vi "COD主界面（列队使用）.vi"() -> (8 "多列列表框":i32(listbox))   [LabVIEW 2016, in "斯坦道CODMn.lvlib"]
uses:
  <vilib>/Analysis/6fits.llb/Curve Fitting Criteria.ctl
  <vilib>/Utility/miscctls.llb/LVPointTypeDef.ctl
  <vilib>/Utility/config.llb/Read Key (I32).vi
  <vilib>/Utility/config.llb/Read Key (Double).vi
  <vilib>/Utility/config.llb/Read Key (Boolean).vi
  <vilib>/Utility/config.llb/Write Key (Double).vi
  <vilib>/Utility/config.llb/Write Key (Boolean).vi
  <vilib>/Utility/config.llb/Write Key (I32).vi
  <vilib>/Waveform/WDTFileIO.llb/Read Waveform from File.vi
  <vilib>/ptbypt/NI_PtbyPt.lvlib
  <vilib>/Utility/config.llb/NI_LVConfig.lvlib
  <vilib>/Analysis/NI_AALPro.lvlib
panel:
  in  "更新程序":bool
  out "进样无液体告警":bool
  out "校准内容显示":string
  out "60分钟超时报警":bool
  in  "远程校准量程":enum16{"L", "H"}(ring)
  in  "远程自动校准浓度":dbl
  in  "仪器参数":bool
  out "CODMn序列号":string
  out "CODMn软件版本：":string
  in  "标样核查量程选择":enum32{"H", "L", "AUTO"}(ring)=enum."AUTO"
  in  "标样浓度":dbl
  in  "零点核查量程选择":enum32{"H", "L", "AUTO"}(ring)=enum."AUTO"
  in  "零点核查浓度":dbl
  out "序列号":string
  in  "采水泵排液时间/s:":i32
  in  "采水泵润洗时间/s:":i32
  in  "采水泵沉淀时间/s:":i32
  in  "采水泵进样时间/s:":i32
  in  "常规版/认证版":enum16{"常规版", "认证版", "浮台版"}(ring)
  in  "释放串口":bool
  in  "打开串口":bool
  in  "保存参数":dbl[](array[numeric])
  out "报警数字":i16
  out "CODMn工作状态":T1(ring)
  out "ORP-K":string
  out "ORP-B":string
  out "ORP-A":string
  out "x = y?":bool
  out "稀释倍数解释":string
  in  "跨度量程选择":enum32{"H", "L", "AUTO"}(ring)=enum."AUTO"
  in  "跨度液浓度":dbl
  in  "水样：":dbl
  in  "蒸馏水：":dbl
  in  "标液：":dbl
  in  "零点核查样：":dbl
  in  "加标回收样：":dbl
  in  "草酸钠":dbl
  in  "高锰酸钾":dbl
  in  "硫酸":dbl
  out "量程解释说明":string
  in  "高切低阈值:":dbl
  in  "低切高阈值:":dbl
  in  "水样量程选择:":enum16{"L", "H", "自动切换测一次", "自动切换测两次"}(ring)
  in  "修正系数：":dbl
  in  "标准液浓度":dbl
  in  "温度":dbl
  in  "恒温时间":dbl
  in  "当前量程：":enum16{"L", "H"}(ring)
  in  "CODMn零点核查选择":enum16{"零点核查走纯水管", "零点核查走零漂管"}(ring)
  in  "锁定按钮":bool
  in  "低量程稀释倍数:":i8=1
  in  "高量程稀释倍数:":i8=2
  in  "一键写入":bool
  in  "测量模式(公式)":u16(ring)=1 items=["水样测试"=1, "标样核查"=2, "零点核查"=3, "跨度核查"=4, "空白测试"=5, "平行样"=6, "加标回收"=7]
  out "基本量程(显示)":string
  out "测量模式(显示)":string
  out "数据时间":string
  out "断电排液标记":bool
  out "COM":string
  in  "启用5":bool
  in  "校准5":bool
  in  "泵滴定数5":dbl
  in  "浓度5":dbl
  in  "启用4":bool
  in  "校准4":bool
  in  "泵滴定数4":dbl
  in  "浓度4":dbl
  out "波形时间":timestamp
  in  "历史波形":bool
  out "滴定数-ORP值":u16[](array[numeric]) caption="数组"
  in  "关闭 3":bool
  in  "滴定曲线":bool
  out "ORP滴定曲线":u16[](graph)
  out "空白测试标记":bool
  out "跨度核查标记":bool
  in  "量程选择":enum16{"低量程", "高量程", "0-2量程"}(ring)
  in  "手动控制":bool
  in  "选用水样":enum16{"葡萄糖", "草酸钠"}(ring)
  in  "方程系数":cluster{"K":dbl, "b":dbl, "X^2":dbl} {"X^2" format="%#.6g"; "b" format="%#.6g"; "K" format="%#.6g"}
  out "多项式系数":dbl[](array[numeric])
  out "XY图":cluster{"X Values":dbl[], "Y Values":dbl[]}[](graph)
  in  "模型":enum32{"线性", "多项式"}(ring)
  out "启动时间":timestamp format="%<%Y/%m/%d %H:%M:%S>T"
  in  "关闭 2":bool
  out "r^2":dbl format="%.8g"
  out "拟合公式":string
  out "b":dbl format="%#.4g"
  out "K":dbl format="%#.4f"
  in  "启用3":bool
  in  "启用2":bool
  in  "启用1":bool
  in  "校准3":bool
  in  "校准2":bool
  in  "校准1":bool
  in  "泵滴定数3":dbl
  in  "泵滴定数2":dbl
  in  "泵滴定数1":dbl
  in  "浓度3":dbl
  in  "浓度2":dbl
  in  "浓度1":dbl
  in  "写入":bool
  out "零点核查标记":bool
  out "排液故障":bool
  out "进水样超量程":bool
  out "标样核查标记":bool
  out "平行样测量":bool
  out "加标回收测量":bool
  out "质控样测量":bool
  out "待机":bool
  out "校标错误":bool
  out "校零错误":bool
  out "测量错误":bool
  out "草酸钠报警":bool
  out "高锰酸钾报警":bool
  out "加热故障":bool
  out "温控器故障":bool
  out "ORP故障":bool
  out "排液标记":bool
  out "故障标记":bool
  out "校标标记":bool
  out "校零标记":bool
  out "通讯状态":bool
  out "水样测量":bool
  in  "读取":bool
  in  "返回":bool
  in  "校准配置":bool
  in  "零点泵计量数 2":dbl
  in  "标度泵计量数 2":dbl
  out "标度滴定值":dbl
  out "零点滴定值":dbl
  in  "保存":bool
  in  "关闭":bool
  out "仪器时间":timestamp format="%<%Y/%m/%d %H:%M:%S>T"
  out "秒":u16
  out "分":u16
  out "COD浓度（mg/L)":dbl format="%.2g"
  out "进样管":dbl
  out "高锰酸钾":dbl
  out "草酸钠":dbl
  out "硫酸":dbl
  out "ORP显示":dbl
  out "温度":dbl
  out "加热":bool
  out "搅拌":bool
  out "进硫酸":bool
  out "进加标回收样":bool
  out "进零点核查样":bool
  out "进标液":bool
  out "进蒸馏水":bool
  out "进水样":bool
  out "进草酸钠":bool
  out "进高锰酸钾":bool
  out "定时启动":bool
  in  "启动":bool
  in  "故障清除":bool
  in  "参数配置":bool
  in  "停止":bool
  in  "单步启动":bool
  out "系统时间":timestamp
  in  "时间校准":bool
  out "模式（受控）":u16
  # "测量时间："
  # "mV"
  # "℃"
  # "注：遇到加热故障和排液故障时仪器不能正常启动，\n必须排查故障并点击报警清除按钮方可运行。"
  # "mg/L"
  # "基本参数设置"
  # "校零校标结果"
  # "泵计量参数设置"
  # "校零结果："
  # "校零滴定值："
  # "加热恒温温度(℃):"
  # "高锰酸钾："
  # "校标结果："
  # "标度滴定值："
  # "恒温时间(分钟):"
  # "草酸钠："
  # "零点泵计量值："
  # "标准液浓度(mg/L):"
  # "硫酸："
  # "标度泵计量值："
  # "跨度核查浓度："
  # "跨度量程选择："
  # "零点核查浓度："
  # "标样浓度："
  # "零点量程选择："
  # "标样量程选择："
  # "远程校准配置区"
  # "公式读取写入区"
  # "mg/L"
  # "是否启用"
  # "泵滴定数"
  # "浓度"
  # "辅\n助\n计\n算\n区"
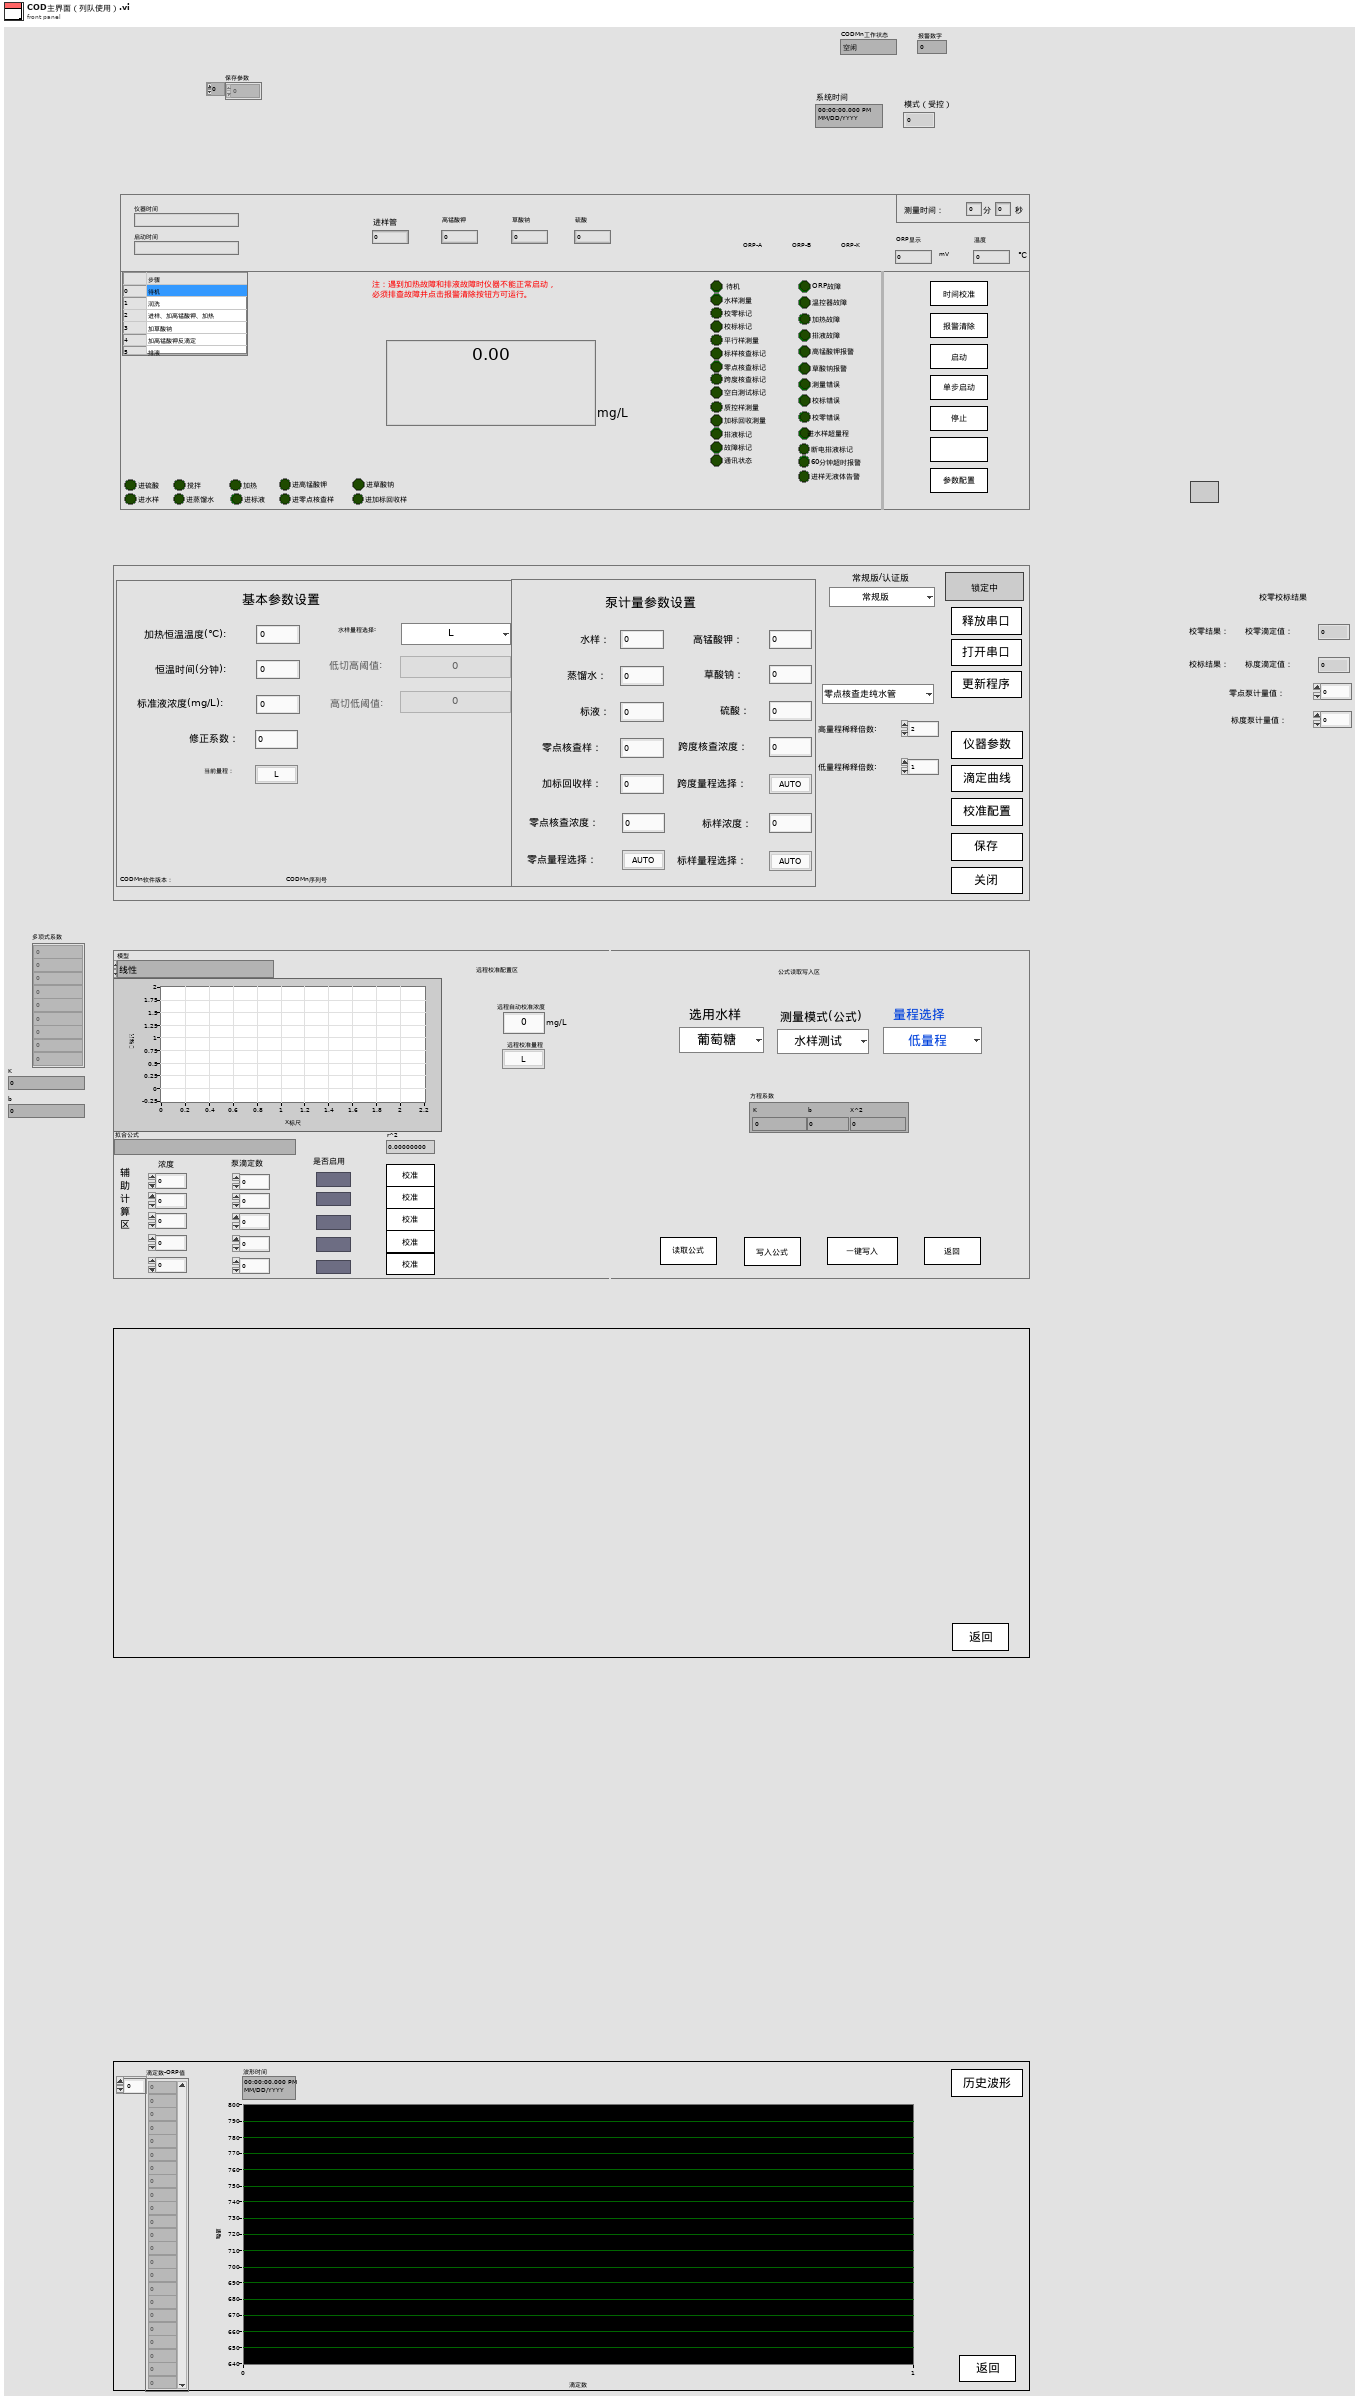
[diagram p1: front panel]
types:
  T1 = enum16{"空闲", "水样测试", "标样核查", "零点核查", "跨度核查", "空白测试", "平行样测试", "质控样", "空白校准", "标样校准", "加标回收"}
  T2 = typedef "NI_AALPro.lvlib/Curve Fitting Criteria.ctl" = u16
  T3 = cluster{"测量量程":dbl, "测量精度":dbl, "测量间隔":dbl, "消解温度":dbl, "消解时长":dbl, "空白校准时间":timestamp, "曲线截距":dbl, "曲线斜率":dbl, "测量检出限":dbl, "测量信号值":dbl, "线性相关系数":dbl, "二次多项式系数":dbl, "标样校准时间":timestamp, "单位":u16}
  T4 = enum8{"Enabled", "Disabled", "Disabled and Grayed Out"}
  T5 = typedef "LVPointTypeDef.ctl" = cluster{"Horizontal":i16, "Vertical":i16}
  T6 = typedef "NI_LVConfig.lvlib/Config Data RefNum.ctl" = refnum<k1>
  T7 = cluster{"时间":timestamp, "测量模式":string, "数据类型":string, "检测值":sgl, "单位":string, "数据标识":string, "因子编码":string, "标样参考值":sgl, "ORP-A":sgl, "ORP-B":sgl, "ORP-K":sgl, "COD滴定值":sgl, "高锰酸钾滴定数":sgl, "温度":sgl, "量程":sgl, "LastTime":timestamp}
  T8 = cluster{"因子编码":u32, "单位":u16, "标样参考值":sgl, "水样数据时间":timestamp, "水样实测值":sgl, "水样数据标识":string, "标样数据时间":timestamp, "标样实测值":sgl, "标样数据标识":string, "空白数据时间":timestamp, "空白实测值":sgl, "空白数据标识":string, "零点核查数据时间":timestamp, "零点核查实测值":sgl, "零点核查数据标识":string, "跨度核查数据时间":timestamp, "跨度核查实测值":sgl, "跨度核查数据标识":string, "加标回收数据时间":timestamp, "加标回收实测值":sgl, "加标回收数据标识":string, "平行样数据时间":timestamp, "平行样实测值":sgl, "平行样数据标识":string}
  T9 = cluster{"控制命令":enum16{"启动测量", "标样核查", "零点核查", "跨度核查", "空白测试", "平行样测试", "加标回收", "空白校准", "标样校准", "初始化（清洗）", "停止测试", "仪器重启", "校时", "模式设置", "测量间隔设置"}, "周期设置类型":enum16{"定点启动", "间隔启动"}, "定时功能启用":bool, "定时间隔":dbl, "24H周期设置":bool[], "零点核查时间":u16, "跨度核查时间":u16, "质控频次":enum16{"关闭", "每天", "星期一", "星期二", "星期三", "星期四", "星期五", "星期六", "星期日"}}
  T10 = cluster{"数组 2[0]":sgl, "数组 2[1]":sgl, "数组 2[2]":sgl, "数组 2[3]":sgl, "数组 2[4]":sgl, "数组 2[5]":sgl, "数组 2[6]":sgl, "数组 2[7]":sgl, "数组 2[8]":sgl, "数组 2[9]":sgl, "数组 2[10]":sgl, "数组 2[11]":sgl, "数组 2[12]":sgl, "数组 2[13]":sgl, "数组 2[14]":sgl, "数组 2[15]":sgl, "数组 2[16]":sgl, "数组 2[17]":sgl, "数组 2[18]":sgl, "数组 2[19]":sgl, "数组 2[20]":sgl, "数组 2[21]":sgl, "数组 2[22]":sgl, "数组 2[23]":sgl, "数组 2[24]":sgl, "数组 2[25]":sgl, "数组 2[26]":sgl, "数组 2[27]":sgl, "数组 2[28]":sgl, "数组 2[29]":sgl, "数组 2[30]":sgl, "数组 2[31]":sgl, "数组 2[32]":sgl, "数组 2[33]":sgl, "数组 2[34]":sgl, "数组 2[35]":sgl, "数组 2[36]":sgl, "数组 2[37]":sgl, "数组 2[38]":sgl, "数组 2[39]":sgl, "数组 2[40]":sgl, "数组 2[41]":sgl}
  T11 = cluster{"ORP故障":bool, "温控器故障":bool, "加热故障":bool, "高锰酸钾报警":bool, "草酸钠报警":bool, "测量错误":bool, "校零错误":bool, "校标错误":bool, " 进水样超量程":bool, "排液阀故障":bool, "60分钟超时报警":bool, "进样无液体报警":bool}
  T12 = cluster{"时间标识":timestamp, "参数":string, "日志信息":string, "流程参数":string}
  T13 = cluster{"控制命令":enum16{"启动测量", "标样核查", "零点核查", "跨度核查", "空白测试", "平行样测试", "加标回收", "空白校准", "标样校准", "初始化（清洗）", "停止测试", "仪器重启", "校时", "模式设置", "测量间隔设置"}, "周期设置类型":enum16{"定点启动", "间隔启动"}, "定时功能启用":bool, "定时间隔":dbl, "24H周期设置":bool[], "空白核查时间":u16, "跨度核查时间":u16, "质控频次":enum16{"关闭", "每天", "星期一", "星期二", "星期三", "星期四", "星期五", "星期六", "星期日"}}
  T14 = cluster{"确定":bool, "测量量程":dbl, "测量精度":dbl, "测量间隔":dbl, "消解温度":dbl, "消解时长":dbl, "空白校准时间":timestamp, "曲线截距":dbl, "曲线斜率":dbl, "测量检出限":dbl, "测量信号值":dbl, "线性相关系数":dbl, "二次多项式系数":dbl, "标样校准时间":timestamp, "单位":u16}
  T15 = cluster{"时间标识":timestamp, "设备":string, "日志信息":string, "流程参数":string}
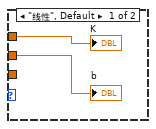
[diagram p5: hidden frame]
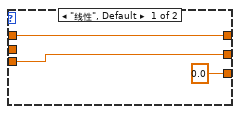
[diagram p7: hidden frame]
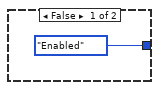
[diagram p8: hidden frame]
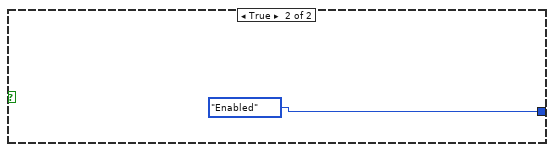
[diagram p9: hidden frame]
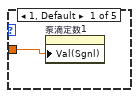
[diagram p14: hidden frame]
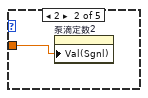
[diagram p15: hidden frame]
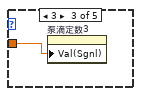
[diagram p16: hidden frame]
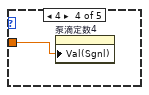
[diagram p17: hidden frame]
diagram:
  n1 = while {
    stop <- FALSE stop-if-true
    w84 = T2 0 items=["最小二乘", "最小绝对残差", "Bisquare"] ("method")
    # "计算线性、多项式公式、远程校准"
    n2 = local read "浓度1"() -> (w57:dbl)
    n3 = local read "浓度2"() -> (w86:dbl)
    n4 = local read "浓度3"() -> (w87:dbl)
    n5 = local read "浓度4"() -> (w79:dbl)
    n6 = local read "浓度5"() -> (w78:dbl)
    n7 = Build Array("泵滴定数1", "泵滴定数2", "泵滴定数3", "泵滴定数4", "泵滴定数5") -> (w85:dbl[])
    n8 = Build Array(w57, w86, w87, w79, w78) -> (w53:dbl[])
    n9 = Build Array("启用1", "启用2", "启用3", "启用4", "启用5") -> (w56:bool[])
    n10 = global read "CODMN外部API.vi" "远程反控校准CODMn"() -> (w54:bool)
    n11 = call "将启用的浓度作为新的浓度数组.vi"("启用布尔数组"=w56, "输入浓度数组"=w53) -> ("启用的浓度数组"=w55:dbl[])  [unwired: 13 in]
    n12 = Unbundle By Name("方程系数") -> ("K"=w65:dbl, "b"=w64:dbl, "X^2"=w63:dbl)
    n13 = case shown="\"多项式\"" "模型" {
      tunnel: w65 -> [w96 w99]
      tunnel: w64 -> [w95 w100]
      tunnel: w63 -> [_ w98]
      frame "线性", Default {
        "K" <- w96
        "b" <- w95
      }
      frame "多项式" {
        n14 = Build Array(w100, w99, w98) -> (→"多项式系数":dbl[])
      }
    }
    n15 = call "线性公式CODMn用.vi"("标液浓度"=w53, "监测浓度"=w85, "启用"=w56, "method"=w84, "模型"="模型", "精度"=6) -> ("拟合方程"=w71:string, "r^2"=→"r^2":dbl, "slope"=w69:dbl, "intercept"=w70:dbl, "XY图"=→"XY图":cluster{"X Values":dbl[], "Y Values":dbl[]}[], "Polynomial Coefficients"=w80:dbl[])  [unwired: 8 in]
    "拟合公式" <- w71
    n16 = call <vilib>:"Boolean Crossing PtByPt.vi"("direction"=enum16{"either", "false-true", "true-false"}."false-true", "input"=w54) -> ("crossing"=w52:bool)  [unwired: 1 in]
    n17 = case shown="真" w52 {
      tunnel: w53 -> [_ w90]
      frame False {
      }
      frame True {
        n18 = global read "CODMn断电保存全局变量.vi" "远程自动校准浓度"() -> (w91:dbl)
        n19 = Search 1D Array(1D array=w90, element=w91) -> (index of element=w92:i32)  [unwired: 1 in]
        n20 = case shown="0, 默认" w92 {
          selector: w92 -> [_ w94]
          frame -1 {
          }
          frame 0, Default {
            n21 = Increment(x=w94) -> (x+1=w93:i32)
            n22 = global write "COD内部交互全局.vi" "当前校准"(w93) -> ()
          }
        }
      }
    }
    n23 = feedback #1(w71) -> (w72:string)
    n24 = feedback-in #1(w71) -> ()
    n25 = Not Equal?(x=w71, y=w72) -> (x != y?=w68:bool)
    n26 = global write "COD内部交互全局.vi" "启用的浓度数组"(w55) -> ()
    n27 = case shown="真" w68 {
      tunnel: w80 -> [_ w107]
      tunnel: w70 -> [_ w108]
      tunnel: w69 -> [_ w109]
      frame False {
      }
      frame True {
        # "当公式发生改变时赋值到右侧公式"
        n28 = local read "模型"() -> (w110:enum32{"线性", "多项式"})
        n29 = case shown="\"多项式\"" w110 {
          tunnel: [w115 w117] -> w103
          tunnel: w109 -> [w115 _]
          tunnel: w108 -> [w114 _]
          tunnel: [w114 w118] -> w104
          tunnel: w107 -> [_ w119]
          tunnel: [0.0 ("数值") w116] -> w102
          frame "线性", Default {
          }
          frame "多项式" {
            # "B,K,X^2"
            n30 = Index Array(array=w119) -> (element #1=w118:dbl, element #2=w117:dbl, element #3=w116:dbl)  [unwired: 3 in]
          }
        }
        n31 = global read "CODMn断电保存全局变量.vi" "CODMn仪器参数"() -> (w106:T3)
        n32 = local read "r^2"() -> (w101:dbl)
        n33 = Bundle By Name(cluster=cluster{"K":dbl, "b":dbl, "X^2":dbl} {"K"=0.0, "b"=0.0, "X^2"=0.0} ("方程系数"), "K"=w103, "b"=w104, "X^2"=w102) -> (w111:cluster{"K":dbl, "b":dbl, "X^2":dbl})
        n34 = Bundle By Name(cluster=w106, "曲线截距"=w104, "曲线斜率"=w103, "二次多项式系数"=w102, "线性相关系数"=w101) -> (w105:T3)
        n35 = global write "CODMn断电保存全局变量.vi" "CODMn仪器参数"(w105) -> ()
        n36 = local write "方程系数"(w111) -> ()
      }
    }
    n37 = Wait (ms)(milliseconds to wait=u32 1000 ("等待时间（毫秒）")) -> ()  [unwired: 1 out]
  }
  n38 = while {
    stop <- FALSE stop-if-true
    n39 = global read "COD内部交互全局.vi" "待机"() -> (w121:bool)
    n40 = Wait (ms)(milliseconds to wait=u32 1000 ("等待时间（毫秒）")) -> ()  [unwired: 1 out]
    n41 = case shown="假" w121 {
      tunnel: [w136 T4."Enabled" ("禁用")] -> w123
      tunnel: [w135 _] -> w122
      frame False {
        # "运行中"
        n42 = global read "COD测量模式全局.vi" "测量模式"() -> (w140:string)
        n43 = global read "COD测量模式全局.vi" "测量模式"() -> (w141:string)
        n44 = Equal?(x=w140, y="校零") -> (x = y?=w138:bool)
        n45 = Equal?(x=w141, y="校标") -> (x = y?=w143:bool)
        n46 = Or(x=w138, y=w143) -> (x .or. y?=w137:bool)
        n47 = case shown="真" w137 {
          tunnel: [T4."Enabled" ("禁用") T4."Disabled and Grayed Out" ("禁用")] -> w136
          tunnel: [_ TRUE] -> w135
          frame False {
          }
          frame True {
          }
        }
      }
      frame True {
      }
    }
    n48 = control-ref of="量程选择"() -> (w129:refnum<vi>)
    n49 = property on="校准内容显示" class="Str"("Visible"=w122) -> ()  [unwired: 2 in, 2 out]
    n50 = control-ref of="选用水样"() -> (w130:refnum<vi>)
    n51 = control-ref of="校准5"() -> (w124:refnum<vi>)
    n52 = control-ref of="校准4"() -> (w125:refnum<vi>)
    n53 = control-ref of="校准3"() -> (w126:refnum<vi>)
    n54 = control-ref of="校准2"() -> (w127:refnum<vi>)
    n55 = control-ref of="校准1"() -> (w128:refnum<vi>)
    n56 = Build Array(w124, w125, w126, w127, w128, w130, w129) -> (w131:refnum<vi>[])
    n57 = for {
      tunnel: w131 -> [w134] mode=indexing
      tunnel: w123 -> [w133]
      n58 = property class="Ctl"(reference=w134, "DisabledEnum"=w133) -> ()  [unwired: 1 in, 2 out]
    }
  }
  n59 = while {
    stop <- FALSE stop-if-true
    # "滚动显示"
    n60 = global read "COD内部交互全局.vi" "待机"() -> (w148:bool)
    n61 = case shown="假" w148 {
      frame False {
        # "运行中"
        n62 = global read "COD内部交互全局.vi" "校准内容显示"() -> (w151:string)
        n63 = while {
          shift-right: [w153] -> _
          shift-left: w151 -> [w158]
          stop <- w152 stop-if-true
          (unwired) "仪器校准中!\n当前校准浓度为:3mg/L" ("校准内容显示")
          n64 = Wait (ms)(milliseconds to wait=u32 500 ("等待时间（毫秒）")) -> ()  [unwired: 1 out]
          n65 = Spreadsheet String To Array(delimiter (Tab)="\n" ("分隔符(Tab)"), format string="" ("格式字符串"), spreadsheet string=w158, array type (2D Dbl)=string[] []) -> (array=w161:string[])
          n66 = for {
            tunnel: w161 -> [w169] mode=indexing
            tunnel: [w167] -> _ mode=indexing
            shift-right: [w165] -> w156
            shift-left: "" ("格式字符串") -> [w166]
            n67 = call "字符串移位显示.vi"("字符框大小"=36, "字符串输入"=w169) -> ("移位后字符串"=w167:string)  [unwired: 8 in, 1 out]
            n68 = Concatenate Strings(w166, w167, "\n" ("分隔符(Tab)")) -> (w165:string)
          }
          n69 = String Length(string=w156) -> (length=w155:i32)
          n70 = Decrement(x=w155) -> (x-1=w154:i32)
          n71 = String Subset(string=w156, length (rest)=w154) -> (substring=w153:string)  [unwired: 1 in]
          "校准内容显示" <- w153
          n72 = global read "COD内部交互全局.vi" "待机"() -> (w152:bool)
        }
      }
      frame True {
      }
    }
    n73 = Wait (ms)(milliseconds to wait=u32 1000 ("等待时间（毫秒）")) -> ()  [unwired: 1 out]
  }
  n74 = while {
    stop <- FALSE stop-if-true
    # "数字键盘输入"
    n75 = event shown="[29] \"远程自动校准浓度\": 鼠标按下" {
      selector: _ -> [_ _ _ _ _ _ _ _ _ _ _ _ _ _ _ _ _ _ _ _ _ _ _ _ _ _ _ _ _ _]
      dyn-events: _ -> [_ _ _ _ _ _ _ _ _ _ _ _ _ _ _ _ _ _ _ _ _ _ _ _ _ _ _ _ _ _]
      timeout: _ -> [_ _ _ _ _ _ _ _ _ _ _ _ _ _ _ _ _ _ _ _ _ _ _ _ _ _ _ _ _ _]
      event Timeout {
        n76 = event-data() -> ()  [unwired: 1 in, 3 out]
      }
      event "温度": Mouse Down {
        n77 = event-data() -> ()  [unwired: 1 in, 8 out]
        n78 = local read "温度"() -> (w172:dbl)
        n79 = call "数字键盘.vi"("OldNumber"=w172) -> ("NewNumber"=w171:sgl)
        n80 = local write "温度"(w171) -> ()
      }
      event "恒温时间": Mouse Down {
        n81 = event-data() -> ()  [unwired: 1 in, 8 out]
        n82 = local read "恒温时间"() -> (w173:dbl)
        n83 = call "数字键盘.vi"("OldNumber"=w173) -> ("NewNumber"=w174:sgl)
        n84 = local write "恒温时间"(w174) -> ()
      }
      event "标准液浓度": Mouse Down {
        n85 = event-data() -> ()  [unwired: 1 in, 8 out]
        n86 = local read "标准液浓度"() -> (w176:dbl)
        n87 = call "数字键盘.vi"("OldNumber"=w176) -> ("NewNumber"=w175:sgl)
        n88 = local write "标准液浓度"(w175) -> ()
      }
      event "修正系数：": Mouse Down {
        n89 = event-data() -> ()  [unwired: 1 in, 8 out]
        n90 = local read "修正系数："() -> (w177:dbl)
        n91 = call "数字键盘.vi"("OldNumber"=w177) -> ("NewNumber"=w178:sgl)
        n92 = local write "修正系数："(w178) -> ()
      }
      event "水样：": Mouse Down {
        n93 = event-data() -> ()  [unwired: 1 in, 8 out]
        n94 = local read "水样："() -> (w179:dbl)
        n95 = call "数字键盘.vi"("OldNumber"=w179) -> ("NewNumber"=w180:sgl)
        n96 = local write "水样："(w180) -> ()
      }
      event "蒸馏水：": Mouse Down {
        n97 = event-data() -> ()  [unwired: 1 in, 8 out]
        n98 = local read "蒸馏水："() -> (w181:dbl)
        n99 = call "数字键盘.vi"("OldNumber"=w181) -> ("NewNumber"=w182:sgl)
        n100 = local write "蒸馏水："(w182) -> ()
      }
      event "标液：": Mouse Down {
        n101 = event-data() -> ()  [unwired: 1 in, 8 out]
        n102 = local read "标液："() -> (w183:dbl)
        n103 = call "数字键盘.vi"("OldNumber"=w183) -> ("NewNumber"=w184:sgl)
        n104 = local write "标液："(w184) -> ()
      }
      event "零点核查样：": Mouse Down {
        n105 = event-data() -> ()  [unwired: 1 in, 8 out]
        n106 = local read "零点核查样："() -> (w185:dbl)
        n107 = call "数字键盘.vi"("OldNumber"=w185) -> ("NewNumber"=w186:sgl)
        n108 = local write "零点核查样："(w186) -> ()
      }
      event "加标回收样：": Mouse Down {
        n109 = event-data() -> ()  [unwired: 1 in, 8 out]
        n110 = local read "加标回收样："() -> (w187:dbl)
        n111 = call "数字键盘.vi"("OldNumber"=w187) -> ("NewNumber"=w188:sgl)
        n112 = local write "加标回收样："(w188) -> ()
      }
      event "草酸钠": Mouse Down {
        n113 = event-data() -> ()  [unwired: 1 in, 8 out]
        n114 = local read "草酸钠"() -> (w189:dbl)
        n115 = call "数字键盘.vi"("OldNumber"=w189) -> ("NewNumber"=w190:sgl)
        n116 = local write "草酸钠"(w190) -> ()
      }
      event "高锰酸钾": Mouse Down {
        n117 = event-data() -> ()  [unwired: 1 in, 8 out]
        n118 = local read "高锰酸钾"() -> (w191:dbl)
        n119 = call "数字键盘.vi"("OldNumber"=w191) -> ("NewNumber"=w192:sgl)
        n120 = local write "高锰酸钾"(w192) -> ()
      }
      event "硫酸": Mouse Down {
        n121 = event-data() -> ()  [unwired: 1 in, 8 out]
        n122 = local read "硫酸"() -> (w193:dbl)
        n123 = call "数字键盘.vi"("OldNumber"=w193) -> ("NewNumber"=w194:sgl)
        n124 = local write "硫酸"(w194) -> ()
      }
      event "零点泵计量数 2": Mouse Down {
        n125 = event-data() -> ()  [unwired: 1 in, 8 out]
        n126 = local read "零点泵计量数 2"() -> (w195:dbl)
        n127 = call "数字键盘.vi"("OldNumber"=w195) -> ("NewNumber"=w196:sgl)
        n128 = local write "零点泵计量数 2"(w196) -> ()
      }
      event "标度泵计量数 2": Mouse Down {
        n129 = event-data() -> ()  [unwired: 1 in, 8 out]
        n130 = local read "标度泵计量数 2"() -> (w197:dbl)
        n131 = call "数字键盘.vi"("OldNumber"=w197) -> ("NewNumber"=w198:sgl)
        n132 = local write "标度泵计量数 2"(w198) -> ()
      }
      event "高量程稀释倍数:": Mouse Down {
        n133 = event-data() -> ()  [unwired: 1 in, 8 out]
        n134 = local read "高量程稀释倍数:"() -> (w200:i8)
        n135 = call "数字键盘.vi"("OldNumber"=w200) -> ("NewNumber"=w199:sgl)
        n136 = local write "高量程稀释倍数:"(w199) -> ()
      }
      event "低量程稀释倍数:": Mouse Down {
        n137 = event-data() -> ()  [unwired: 1 in, 8 out]
        n138 = local read "低量程稀释倍数:"() -> (w202:i8)
        n139 = call "数字键盘.vi"("OldNumber"=w202) -> ("NewNumber"=w201:sgl)
        n140 = local write "低量程稀释倍数:"(w201) -> ()
      }
      event "浓度1": Mouse Down {
        n141 = event-data() -> ()  [unwired: 1 in, 8 out]
        n142 = local read "浓度1"() -> (w204:dbl)
        n143 = call "数字键盘.vi"("OldNumber"=w204) -> ("NewNumber"=w203:sgl)
        n144 = property on="浓度1" class="DigNum (严格)"("Val(Sgnl)"=w203) -> ()  [unwired: 2 in, 2 out]
      }
      event "浓度2": Mouse Down {
        n145 = event-data() -> ()  [unwired: 1 in, 8 out]
        n146 = local read "浓度2"() -> (w206:dbl)
        n147 = call "数字键盘.vi"("OldNumber"=w206) -> ("NewNumber"=w205:sgl)
        n148 = property on="浓度2" class="DigNum (严格)"("Val(Sgnl)"=w205) -> ()  [unwired: 2 in, 2 out]
      }
      event "浓度3": Mouse Down {
        n149 = event-data() -> ()  [unwired: 1 in, 8 out]
        n150 = local read "浓度3"() -> (w208:dbl)
        n151 = call "数字键盘.vi"("OldNumber"=w208) -> ("NewNumber"=w207:sgl)
        n152 = property on="浓度3" class="DigNum (严格)"("Val(Sgnl)"=w207) -> ()  [unwired: 2 in, 2 out]
      }
      event "浓度4": Mouse Down {
        n153 = event-data() -> ()  [unwired: 1 in, 8 out]
        n154 = local read "浓度4"() -> (w210:dbl)
        n155 = call "数字键盘.vi"("OldNumber"=w210) -> ("NewNumber"=w209:sgl)
        n156 = property on="浓度4" class="DigNum (严格)"("Val(Sgnl)"=w209) -> ()  [unwired: 2 in, 2 out]
      }
      event "浓度5": Mouse Down {
        n157 = event-data() -> ()  [unwired: 1 in, 8 out]
        n158 = local read "浓度5"() -> (w212:dbl)
        n159 = call "数字键盘.vi"("OldNumber"=w212) -> ("NewNumber"=w211:sgl)
        n160 = property on="浓度5" class="DigNum (严格)"("Val(Sgnl)"=w211) -> ()  [unwired: 2 in, 2 out]
      }
      event "跨度液浓度", "零点核查浓度", "标样浓度": Mouse Down {
        n161 = event-data() -> ("CtlRef"=w216:refnum<vi>)  [unwired: 1 in, 7 out]
        n162 = property class="DigNum (严格)"(reference=w216) -> (reference out=w213:refnum<vi>, "Value"=w215:dbl)  [unwired: 1 in, 1 out]
        n163 = call "数字键盘.vi"("OldNumber"=w215) -> ("NewNumber"=w214:sgl)
        n164 = property class="DigNum (严格)"(reference=w213, "Val(Sgnl)"=w214) -> ()  [unwired: 1 in, 2 out]
      }
      event "泵滴定数1": Mouse Down {
        n165 = event-data() -> ()  [unwired: 1 in, 8 out]
        n166 = local read "泵滴定数1"() -> (w218:dbl)
        n167 = call "数字键盘.vi"("OldNumber"=w218) -> ("NewNumber"=w217:sgl)
        n168 = property on="泵滴定数1" class="DigNum (严格)"("Val(Sgnl)"=w217) -> ()  [unwired: 2 in, 2 out]
      }
      event "泵滴定数2": Mouse Down {
        n169 = event-data() -> ()  [unwired: 1 in, 8 out]
        n170 = local read "泵滴定数2"() -> (w220:dbl)
        n171 = call "数字键盘.vi"("OldNumber"=w220) -> ("NewNumber"=w219:sgl)
        n172 = property on="泵滴定数2" class="DigNum (严格)"("Val(Sgnl)"=w219) -> ()  [unwired: 2 in, 2 out]
      }
      event "泵滴定数3": Mouse Down {
        n173 = event-data() -> ()  [unwired: 1 in, 8 out]
        n174 = local read "泵滴定数3"() -> (w222:dbl)
        n175 = call "数字键盘.vi"("OldNumber"=w222) -> ("NewNumber"=w221:sgl)
        n176 = property on="泵滴定数3" class="DigNum (严格)"("Val(Sgnl)"=w221) -> ()  [unwired: 2 in, 2 out]
      }
      event "泵滴定数4": Mouse Down {
        n177 = event-data() -> ()  [unwired: 1 in, 8 out]
        n178 = local read "泵滴定数4"() -> (w224:dbl)
        n179 = call "数字键盘.vi"("OldNumber"=w224) -> ("NewNumber"=w223:sgl)
        n180 = property on="泵滴定数4" class="DigNum (严格)"("Val(Sgnl)"=w223) -> ()  [unwired: 2 in, 2 out]
      }
      event "泵滴定数5": Mouse Down {
        n181 = event-data() -> ()  [unwired: 1 in, 8 out]
        n182 = local read "泵滴定数5"() -> (w226:dbl)
        n183 = call "数字键盘.vi"("OldNumber"=w226) -> ("NewNumber"=w225:sgl)
        n184 = property on="泵滴定数5" class="DigNum (严格)"("Val(Sgnl)"=w225) -> ()  [unwired: 2 in, 2 out]
      }
      event "低切高阈值:", "高切低阈值:": Mouse Down {
        n185 = event-data() -> ("CtlRef"=w230:refnum<vi>)  [unwired: 1 in, 7 out]
        n186 = property class="DigNum (严格)"(reference=w230) -> (reference out=w229:refnum<vi>, "Value"=w228:dbl)  [unwired: 1 in, 1 out]
        n187 = call "数字键盘.vi"("OldNumber"=w228) -> ("NewNumber"=w227:sgl)
        n188 = property class="DigNum (严格)"(reference=w229, "Val(Sgnl)"=w227) -> ()  [unwired: 1 in, 2 out]
      }
      event "远程自动校准浓度": Mouse Down {
        n189 = event-data() -> ("CtlRef"=w231:refnum<vi>)  [unwired: 1 in, 7 out]
        n190 = One Button Dialog(message="请输入其中一个在拟合公式中的非零浓度，用于远程校标！" ("消息")) -> (true=w233:bool)  [unwired: 1 in]
        n191 = case shown="真" w233 {
          tunnel: w231 -> [_ w240]
          frame False {
          }
          frame True {
            n192 = property class="DigNum (严格)"(reference=w240) -> (reference out=w235:refnum<vi>, "Value"=w241:dbl)  [unwired: 1 in, 1 out]
            n193 = global read "COD内部交互全局.vi" "启用的浓度数组"() -> (w237:dbl[])
            n194 = call "数字键盘.vi"("OldNumber"=w241) -> ("NewNumber"=w234:sgl)
            n195 = Search 1D Array(1D array=w237, element=w234) -> (index of element=w238:i32)  [unwired: 1 in]
            n196 = Equal?(x=w238, y=-1) -> (x = y?=w236:bool)
            n197 = case shown="真" w236 {
              tunnel: w235 -> [w243 _]
              tunnel: w234 -> [w242 _]
              frame False {
                n198 = property class="DigNum (严格)"(reference=w243, "Val(Sgnl)"=w242) -> ()  [unwired: 1 in, 2 out]
              }
              frame True {
                n199 = One Button Dialog(message="该浓度不属于校准浓度范围，请重新输入！" ("消息")) -> ()  [unwired: 1 in, 1 out]
              }
            }
          }
        }
      }
    }
  }
  n200 = flat-sequence {
    tunnel: [w245] -> w1
    tunnel: [errorcluster {"status"=FALSE, "code"=0, "source"=""} ("错误输出")] -> w38
    frame #0 {
      w258 = "192.168.1.100" ("名称")
      n201 = global write "COD内部交互全局.vi" "量程切换次数"(u8 0 ("量程切换次数")) -> ()
      n202 = global write "COD内部交互全局.vi" "切换量程连续测两次"(FALSE ("切换量程连续测两次")) -> ()
      n203 = global read "COD内部交互全局.vi" "序列号:"() -> (w266:string)
      "序列号" <- w266
      n204 = property on="窗格" class="Pane"("Origin"=T5 {"Horizontal"=0, "Vertical"=0} ("原点")) -> ()  [unwired: 2 in, 2 out]
      n205 = Empty String/Path?(string/path=w266) -> (empty?=w267:bool)
      n206 = case shown="真" w267 {
        tunnel: w266 -> [w282 _]
        tunnel: [w281 "data\\Set.ini" ("名称或相对路径")] -> w246
        frame False {
          # "与生产用上位机交互"
          n207 = Concatenate Strings("data\\" ("字符串"), "序列号" ("字符串"), w282, "Set.ini" ("名称或相对路径")) -> (w281:string)
        }
        frame True {
        }
      }
      n208 = String To IP(1:w258) -> (0:w251:u32)
      n209 = IP To String(2:w251) -> (0:w254:string)  [unwired: 1 in]
      n210 = Not Equal?(x=w258, y=w254) -> (x != y?=w259:bool)
      n211 = Concatenate Strings("\\\\" ("字符串"), w254) -> (w253:string)
      n212 = global write "CODMN外部API.vi" "ping"(w259) -> ()
      n213 = String To Path(string=w253) -> (path=w261:path)
      n214 = Build Path(base path=w261, name or relative path=w246) -> (appended path=w255:path)
      n215 = local write "量程选择"(enum16{"低量程", "高量程", "0-2量程"}."低量程" ("量程选择")) -> ()
      n216 = local write "选用水样"(enum16{"葡萄糖", "草酸钠"}."葡萄糖" ("选用水样")) -> ()
      n217 = global write "COD内部交互全局.vi" "配置文件ini"(w246) -> ()
      n218 = case shown="假" w259 {
        tunnel: w255 -> [w272 w276]
        tunnel: [w272 w275] -> w256
        tunnel: [FALSE w274] -> w257
        frame False {
        }
        frame True {
          n219 = call <vilib>:"Check if File or Folder Exists.vi"("path"=w276) -> ("file or folder exists?"=w274:bool, "dup path"=w275:path)  [unwired: 8 in, 1 out]
        }
      }
      n220 = case shown="假" w257 {
        tunnel: w256 -> [_ w280]
        tunnel: [w278 w280] -> w260
        tunnel: w246 -> [w277 _]
        frame False {
          # "本地文件地址"
          n221 = call <vilib>:"Application Directory.vi"() -> ("Application Directory"=w279:path)
          n222 = Build Path(base path=w279, name or relative path=w277) -> (appended path=w278:path)
        }
        frame True {
          # "网络共享地址"
        }
      }
      n223 = global write "CODMN外部API.vi" "配置文件 path"(w260) -> ()
      n224 = call <vilib>:"Open Config Data.vi"("configuration file path"=w260) -> ("error out"=w247:errorcluster, "refnum"=w248:T6)  [unwired: 8 in, 1 out]
      n225 = vi-ref "斯坦道CODMn.lvlib:CODMn断电保存全局变量.vi"() -> (w262:refnum<vi>)
      n226 = call <userlib>:"Read Panel from INI__ogtk.vi"("error in (no error)"=w247, "VI ref"=w262, "refnum"=w248) -> ("error out"=w249:errorcluster, "refnum out"=w250:T6)  [unwired: 7 in]
      n227 = call <vilib>:"Close Config Data.vi"("error in (no error)"=w249, "refnum"=w250) -> ("error out"=w245:errorcluster)  [unwired: 8 in, 1 out]
      "稀释倍数解释" <- "稀释倍数解释：\n稀释倍数选择1，表示不稀释\n默认低量程系数倍数1，高量程系数倍数2\n则低量程为0~8，高量程为0~16" ("稀释倍数解释")
    }
  }
  n228 = while {
    stop <- FALSE stop-if-true
    # "赋值循环"
    n229 = flat-sequence {
      frame #0 {
        # "测量数据区"
        n230 = global read "COD内部交互全局.vi" "data"() -> (w531:T7)
        n231 = global read "CODMn断电保存全局变量.vi" "测量数据区"() -> (w525:T8)
        n232 = global read "COD测量模式全局.vi" "测量模式"() -> (w527:string)
        "测量模式(显示)" <- w527
        n233 = Unbundle By Name(w531) -> ("时间"=w530:timestamp, "检测值"=w529:sgl, "数据标识"=w528:string)
        n234 = case shown="\"空白测试\"" w527 {
          tunnel: w525 -> [w549 w554 w559 w564 w569 w574 w579 w584 w589 w594]
          tunnel: [w549 w553 w558 w560 w568 w573 w578 w583 w585 w593] -> w526
          tunnel: w530 -> [_ w552 w557 w563 w567 w572 w577 w582 w588 w592]
          tunnel: w529 -> [_ w551 w556 w562 w566 w571 w576 w581 w587 w591]
          tunnel: w528 -> [_ w550 w555 w561 w565 w570 w575 w580 w586 w590]
          frame "", Default {
          }
          frame "水样测试" {
            n235 = Bundle By Name(cluster=w554, "水样数据时间"=w552, "水样实测值"=w551, "水样数据标识"=w550) -> (w553:T8)
          }
          frame "标样核查" {
            n236 = Bundle By Name(cluster=w559, "标样数据时间"=w557, "标样实测值"=w556, "标样数据标识"=w555) -> (w558:T8)
          }
          frame "跨度核查" {
            n237 = Bundle By Name(cluster=w564, "跨度核查数据时间"=w563, "跨度核查实测值"=w562, "跨度核查数据标识"=w561) -> (w560:T8)
          }
          frame "零点核查" {
            n238 = Bundle By Name(cluster=w569, "零点核查数据时间"=w567, "零点核查实测值"=w566, "零点核查数据标识"=w565) -> (w568:T8)
          }
          frame "空白测试" {
            n239 = Bundle By Name(cluster=w574, "空白数据时间"=w572, "空白实测值"=w571, "空白数据标识"=w570) -> (w573:T8)
          }
          frame "加标回收" {
            n240 = Bundle By Name(cluster=w579, "加标回收数据时间"=w577, "加标回收实测值"=w576, "加标回收数据标识"=w575) -> (w578:T8)
          }
          frame "平行样" {
            n241 = Bundle By Name(cluster=w584, "平行样数据时间"=w582, "平行样实测值"=w581, "平行样数据标识"=w580) -> (w583:T8)
          }
          frame "校零" {
            n242 = Bundle By Name(cluster=w589, "空白数据时间"=w588, "空白实测值"=w587, "空白数据标识"=w586) -> (w585:T8)
          }
          frame "校标" {
            n243 = Bundle By Name(cluster=w594, "标样数据时间"=w592, "标样实测值"=w591, "标样数据标识"=w590) -> (w593:T8)
          }
        }
        n244 = Unbundle By Name(w525) -> ("水样实测值"=w522:sgl)
        n245 = feedback-in #2(w525) -> ()
        n246 = feedback #2(w525) -> (w524:T8)
        n247 = Unbundle By Name(w524) -> ("水样实测值"=w523:sgl)
        n248 = Not Equal?(x=w522, y=w523) -> (x != y?=w521:bool)
        n249 = case shown="真" w521 {
          frame False {
          }
          frame True {
            # "水样值发送改变存储本地"
            n250 = global read "CODMN外部API.vi" "ping"() -> (w533:bool)
            n251 = case shown="假" w533 {
              tunnel: [w545 w548] -> w532
              frame False {
                n252 = global read "COD内部交互全局.vi" "配置文件ini"() -> (w547:string)
                n253 = call <vilib>:"Application Directory.vi"() -> ("Application Directory"=w546:path)
                n254 = Build Path(base path=w546, name or relative path=w547) -> (appended path=w545:path)
              }
              frame True {
                n255 = global read "CODMN外部API.vi" "配置文件 path"() -> (w548:path)
              }
            }
            n256 = call <vilib>:"Open Config Data.vi"("configuration file path"=w532) -> ("error out"=w541:errorcluster, "refnum"=w544:T6)  [unwired: 8 in, 1 out]
            n257 = vi-ref "斯坦道CODMn.lvlib:CODMn断电保存全局变量.vi"() -> (w543:refnum<vi>)
            n258 = call <userlib>:"Write Panel to INI__ogtk.vi"("error in (no error)"=w541, "VI ref"=w543, "refnum"=w544) -> ("error out"=w540:errorcluster, "refnum out"=w542:T6)  [unwired: 7 in]
            n259 = call <vilib>:"Close Config Data.vi"("error in (no error)"=w540, "refnum"=w542) -> ("error out"=w535:errorcluster, "file path"=w534:path)  [unwired: 8 in]
            n260 = Open/Create/Replace File(file path (use dialog)=w534, error in=w535) -> (refnum out=w538:refnum<file>, error out=w539:errorcluster)  [unwired: 4 in, 1 out]
            n261 = Flush File(refnum=w538, error in=w539) -> (refnum out=w537:refnum<file>, error out=w536:errorcluster)
            n262 = Close File(refnum=w537, error in=w536) -> ()  [unwired: 2 out]
          }
        }
        n263 = global write "CODMn断电保存全局变量.vi" "测量数据区"(w526) -> ()
      }
    }
    n264 = flat-sequence {
      frame #0 {
        # "局部变量给内部交互用全局变量"
        n265 = local read "温度"() -> (w315:dbl)
        n266 = local read "COD浓度（mg/L)"() -> (w321:dbl)
        n267 = local read "CODMn工作状态"() -> (w324:T1)
        n268 = local read "多列列表框"() -> (w322:i32)
        n269 = local read "标准液浓度"() -> (w320:dbl)
        n270 = local read "高锰酸钾报警"() -> (w318:bool)
        n271 = local read "断电排液标记"() -> (w317:bool)
        n272 = local read "ORP显示"() -> (w314:dbl)
        n273 = local read "故障标记"() -> (w323:bool)
        n274 = local read "高锰酸钾"() -> (w316:dbl)
        n275 = global write "COD内部交互全局.vi" "实时温度"(w315) -> ()
        n276 = local read "待机"() -> (w319:bool)
        n277 = global write "运行时序全局变量.vi" "多列列表框"(w322) -> ()
        n278 = global write "COD内部交互全局.vi" "故障标记"(w323) -> ()
        n279 = global write "COD内部交互全局.vi" "ORP显示"(w314) -> ()
        n280 = global write "COD浓度全局变量.vi" "标准液浓度"(w320) -> ()
        n281 = global write "COD内部交互全局.vi" "高锰酸钾"(w316) -> ()
        n282 = global write "COD内部交互全局.vi" "待机"(w319) -> ()
        n283 = global write "COD测量模式全局.vi" "CODMn工作状态"(w324) -> ()
        n284 = global write "COD内部交互全局.vi" "高锰酸钾报警"(w318) -> ()
        n285 = global write "COD内部交互全局.vi" "断电排液标记"(w317) -> ()
        n286 = global write "COD浓度全局变量.vi" "COD浓度（mg/L)"(w321) -> ()
      }
    }
    n287 = flat-sequence {
      frame #0 {
        # "断电保存全局给局部变量"
        n288 = global read "CODMn断电保存全局变量.vi" "高切低阈值:"() -> (w609:dbl)
        n289 = global read "CODMn断电保存全局变量.vi" "低切高阈值:"() -> (w608:dbl)
        n290 = global read "CODMn断电保存全局变量.vi" "跨度液浓度"() -> (w606:dbl)
        n291 = global read "COD内部交互全局.vi" "波形时间"() -> (w595:timestamp)
        n292 = global read "CODMn断电保存全局变量.vi" "启动时间"() -> (→"启动时间":timestamp)
        n293 = global read "CODMn断电保存全局变量.vi" "标样浓度"() -> (w604:dbl)
        n294 = global read "CODMn断电保存全局变量.vi" "定时控制"() -> (w599:T9)
        n295 = global read "CODMn断电保存全局变量.vi" "CODMn跨度量程选择"() -> (w610:enum32{"H", "L", "AUTO"})
        n296 = global read "CODMn断电保存全局变量.vi" "标样核查量程选择"() -> (w601:enum32{"H", "L", "AUTO"})
        n297 = global read "CODMn断电保存全局变量.vi" "零点核查量程选择"() -> (w603:enum32{"H", "L", "AUTO"})
        n298 = global read "CODMn断电保存全局变量.vi" "测量模式(公式)"() -> (w611:u16)
        n299 = global read "COD内部交互全局.vi" "滴定数-ORP值"() -> (→"滴定数-ORP值":u16[])
        n300 = global read "CODMn断电保存全局变量.vi" "常规版/认证版"() -> (w605:enum16{"常规版", "认证版", "浮台版"})
        n301 = global read "CODMn断电保存全局变量.vi" "自动切换量程:"() -> (w607:enum16{"L", "H", "自动切换测一次", "自动切换测两次"})
        n302 = global read "CODMn断电保存全局变量.vi" "零点核查浓度"() -> (w602:dbl)
        n303 = global read "COD内部交互全局.vi" "ORP滴定曲线"() -> (→"ORP滴定曲线":u16[])
        n304 = local write "高切低阈值:"(w609) -> ()
        n305 = local write "波形时间"(w595) -> ()
        n306 = local write "标样浓度"(w604) -> ()
        n307 = Unbundle By Name(w599) -> ("定时功能启用"=→"定时启动":bool)
        n308 = local write "跨度液浓度"(w606) -> ()
        n309 = local write "低切高阈值:"(w608) -> ()
        n310 = local write "标样核查量程选择"(w601) -> ()
        n311 = local write "水样量程选择:"(w607) -> ()
        n312 = local write "常规版/认证版"(w605) -> ()
        n313 = local write "零点核查浓度"(w602) -> ()
        n314 = local write "零点核查量程选择"(w603) -> ()
        n315 = local write "测量模式(公式)"(w611) -> ()
        n316 = local write "跨度量程选择"(w610) -> ()
      }
    }
    n317 = flat-sequence {
      frame #0 {
        # "保存参数赋值"
        n318 = Multiply(x="温度", y=10.0) -> (x*y=w299:dbl)
        n319 = Multiply(x="标准液浓度", y=100.0) -> (x*y=w293:dbl)
        n320 = Multiply(x="修正系数：", y=100.0) -> (x*y=w296:dbl)
        n321 = Build Array(w299, "恒温时间", w293, w296, "当前量程：", "水样：", "蒸馏水：", "标液：", "零点核查样：", "加标回收样：", "高锰酸钾", "草酸钠", "硫酸", "零点泵计量数 2", "标度泵计量数 2", "高量程稀释倍数:", "低量程稀释倍数:", "CODMn零点核查选择") -> (w290:dbl[])
        n322 = local write "保存参数"(w290) -> ()
      }
    }
    n323 = flat-sequence {
      frame #0 {
        # "显示量程说明"
        n324 = global read "COD内部交互全局.vi" "通讯状态"() -> (→"通讯状态":bool)
        n325 = global read "CODMn断电保存全局变量.vi" "MB通信方式选择"() -> (w612:enum16{"串口", "TCP"})
        n326 = local read "低量程稀释倍数:"() -> (w626:i8)
        n327 = local read "高量程稀释倍数:"() -> (w616:i8)
        n328 = case shown="\"TCP\"" w612 {
          tunnel: [w629 w630] -> w617
          frame "串口", Default {
            n329 = global read "CODMn断电保存全局变量.vi" "VISA resource name"() -> (w629:refnum<visa-resource-name>)
          }
          frame "TCP" {
            n330 = global read "CODMn断电保存全局变量.vi" "IP"() -> (w630:string)
          }
        }
        "COM" <- w617
        n331 = Multiply(x=w626, y=i8 8) -> (x*y=w618:i8)
        n332 = Multiply(x=w616, y=i8 8) -> (x*y=w614:i8)
        n333 = Number To Decimal String(number=w618) -> (decimal integer string=w623:string)  [unwired: 1 in]
        n334 = Number To Decimal String(number=w614) -> (decimal integer string=w621:string)  [unwired: 1 in]
        n335 = Concatenate Strings("L低量程范围:0~" ("量程解释说明"), w623, "(mg/L)\n\nH高量程范围:" ("量程解释说明"), "0" ("字符串"), "~" ("量程解释说明"), w621, "(mg/L)" ("量程解释说明")) -> (→"量程解释说明":string)
      }
    }
    n336 = flat-sequence {
      frame #0 {
        # "参数赋值（只在读取参数时候改变一次）"
        n337 = global read "COD内部交互全局.vi" "读取浮台参数显示"() -> (w326:bool)
        n338 = global read "COD内部交互全局.vi" "读取浮台参数"() -> (w325:u16[])
        n339 = global read "COD内部交互全局.vi" "读取参数显示"() -> (w327:bool)
        n340 = global read "COD内部交互全局.vi" "读取参数"() -> (w328:u16[])
        n341 = case shown="真" w326 {
          tunnel: w325 -> [_ w334]
          frame False {
          }
          frame True {
            n342 = Index Array(array=w334) -> (element #1=w333:u16, element #2=w332:u16, element #3=w331:u16, element #4=w330:u16)  [unwired: 4 in]
            n343 = global write "COD内部交互全局.vi" "读取浮台参数显示"(FALSE ("读取参数显示")) -> ()
            n344 = local write "采水泵进样时间/s:"(w333) -> ()
            n345 = local write "采水泵润洗时间/s:"(w332) -> ()
            n346 = local write "采水泵沉淀时间/s:"(w331) -> ()
            n347 = local write "采水泵排液时间/s:"(w330) -> ()
          }
        }
        n348 = case shown="真" w327 {
          tunnel: w328 -> [_ w351]
          frame False {
          }
          frame True {
            n349 = Index Array(array=w351) -> (element #1=w363:u16, element #2=w375:u16, element #3=w356:u16, element #4=w361:u16, element #5=w359:u16, element #6=w358:u16, element #7=w374:u16, element #8=w373:u16, element #9=w372:u16, element #10=w371:u16, element #11=w370:u16, element #12=w369:u16, element #13=w368:u16, element #14=w367:u16, element #15=w366:u16, element #16=w354:u16, element #17=w353:u16, element #18=w352:u16, element #19=w349:u16, element #20=w348:u16, element #21=w347:u16, element #22=w346:u16, element #23=w345:u16, element #27=w341:u16, element #28=w340:u16, element #29=w339:u16, element #30=w338:u16, element #31=w337:u16)  [unwired: 31 in, 3 out]
            n350 = global write "COD内部交互全局.vi" "读取参数显示"(FALSE ("读取参数显示")) -> ()
            n351 = local write "水样："(w358) -> ()
            n352 = local write "标液："(w373) -> ()
            n353 = local write "硫酸"(w368) -> ()
            n354 = local write "零点核查样："(w372) -> ()
            n355 = local write "加标回收样："(w371) -> ()
            n356 = local write "当前量程："(w359) -> ()
            n357 = local write "蒸馏水："(w374) -> ()
            n358 = local write "恒温时间"(w375) -> ()
            n359 = local write "高锰酸钾"(w370) -> ()
            n360 = local write "草酸钠"(w369) -> ()
            n361 = local write "零点泵计量数 2"(w367) -> ()
            n362 = local write "标度泵计量数 2"(w366) -> ()
            n363 = local write "高量程稀释倍数:"(w354) -> ()
            n364 = local write "低量程稀释倍数:"(w353) -> ()
            n365 = local write "CODMn零点核查选择"(w352) -> ()
            n366 = Build Array(w349, w348, w347, w346, w345) -> (w344:u16[])
            n367 = Build Array(w341, w340, w339, w338, w337) -> (w336:u16[])
            n368 = Divide(x=w363, y=u16 10) -> (x/y=w364:dbl)
            n369 = Divide(x=w356, y=u16 100) -> (x/y=w355:dbl)
            n370 = Divide(x=w361, y=u16 100) -> (x/y=w360:dbl)
            n371 = local write "修正系数："(w360) -> ()
            n372 = local write "温度"(w364) -> ()
            n373 = local write "标准液浓度"(w355) -> ()
            n374 = call "HexToString.vi"("数组"=w336) -> ("字符串"=→"CODMn序列号":string)  [unwired: 10 in]
            n375 = call "FATEK_HexToString.vi"("数组"=w344) -> ("STRING"=w343:string[])  [unwired: 10 in]
            n376 = Index Array(array=w343) -> (element=→"CODMn软件版本：":string)  [unwired: 1 in]
          }
        }
      }
    }
    n377 = flat-sequence {
      frame #0 {
        # "权限隐藏和显示功能"
        n378 = local read "x = y?"() -> (w631:bool)
        n379 = property on="更新程序" class="Bool (严格)"("Visible"=w631) -> ()  [unwired: 2 in, 2 out]
        n380 = property on="释放串口" class="Bool"("Visible"=w631) -> ()  [unwired: 2 in, 2 out]
        n381 = property on="打开串口" class="Bool"("Visible"=w631) -> ()  [unwired: 2 in, 2 out]
        n382 = property on="常规版/认证版" class="Enum (严格)"("Visible"=w631) -> ()  [unwired: 2 in, 2 out]
        n383 = property on="CODMn零点核查选择" class="Enum (严格)"("Visible"=w631) -> ()  [unwired: 2 in, 2 out]
        n384 = property on="低量程稀释倍数:" class="DigNum (严格)"("Visible"=w631) -> ()  [unwired: 2 in, 2 out]
        n385 = property on="稀释倍数解释" class="Str"("Visible"=w631) -> ()  [unwired: 2 in, 2 out]
        n386 = property on="高量程稀释倍数:" class="DigNum (严格)"("Visible"=w631) -> ()  [unwired: 2 in, 2 out]
        n387 = local read "常规版/认证版"() -> (w646:enum16{"常规版", "认证版", "浮台版"})
        n388 = case shown="\"常规版\", 默认" w646 {
          tunnel: [T4."Enabled" ("禁用") T4."Disabled and Grayed Out" ("禁用") T4."Enabled" ("禁用")] -> w645
          tunnel: [i32[] [2] ("禁用项[]") i32[] [] ("禁用项[]") i32[] [2] ("禁用项[]")] -> w644
          tunnel: [w654 T4."Disabled and Grayed Out" ("禁用") w664] -> w643
          tunnel: [FALSE FALSE TRUE] -> w642
          tunnel: [w654 T4."Disabled and Grayed Out" ("禁用") w664] -> w632
          frame "常规版", Default {
            w654 = T4."Enabled" ("禁用")
          }
          frame "认证版" {
            w660 = u16 1 items=["水样测试"=1, "标样核查"=2, "零点核查"=3, "跨度核查"=4, "空白测试"=5, "平行样"=6, "加标回收"=7] ("测量模式(公式)")
            n389 = global write "CODMn断电保存全局变量.vi" "测量模式(公式)"(w660) -> ()
          }
          frame "浮台版" {
            w664 = T4."Enabled" ("禁用")
          }
        }
        n390 = control-ref of="水样："() -> (w641:refnum<vi>)
        n391 = control-ref of="蒸馏水："() -> (w640:refnum<vi>)
        n392 = control-ref of="标液："() -> (w639:refnum<vi>)
        n393 = control-ref of="零点核查样："() -> (w638:refnum<vi>)
        n394 = control-ref of="加标回收样："() -> (w637:refnum<vi>)
        n395 = local read "水样量程选择:"() -> (w648:enum16{"L", "H", "自动切换测一次", "自动切换测两次"})
        n396 = control-ref of="量程解释说明"() -> (w635:refnum<vi>)
        n397 = control-ref of="修正系数："() -> (w636:refnum<vi>)
        n398 = Not Equal To 0?(x=w648) -> (x != 0?=w647:bool)
        n399 = control-ref of="进样管"() -> (w633:refnum<vi>)
        n400 = Build Array(w641, w640, w639, w638, w637, w635, w636, w633) -> (w634:refnum<vi>[])
        n401 = Select(t=T4."Enabled" ("禁用"), s=w647, f=T4."Disabled and Grayed Out" ("禁用")) -> (s? t:f=w649:T4)
        n402 = for {
          tunnel: w634 -> [w653] mode=indexing
          tunnel: w632 -> [w652]
          n403 = property class="Ctl"(reference=w653, "DisabledEnum"=w652) -> ()  [unwired: 1 in, 2 out]
        }
        n404 = property on="低切高阈值:" class="DigNum (严格)"("DisabledEnum"=w649) -> ()  [unwired: 2 in, 2 out]
        n405 = property on="高切低阈值:" class="DigNum (严格)"("DisabledEnum"=w649) -> ()  [unwired: 2 in, 2 out]
        n406 = property on="采水泵润洗时间/s:" class="DigNum (严格)"("Visible"=w642) -> ()  [unwired: 2 in, 2 out]
        n407 = property on="采水泵沉淀时间/s:" class="DigNum (严格)"("Visible"=w642) -> ()  [unwired: 2 in, 2 out]
        n408 = property on="采水泵排液时间/s:" class="DigNum (严格)"("Visible"=w642) -> ()  [unwired: 2 in, 2 out]
        n409 = property on="采水泵进样时间/s:" class="DigNum (严格)"("Visible"=w642) -> ()  [unwired: 2 in, 2 out]
        n410 = property on="一键写入" class="Bool (严格)"("DisabledEnum"=w643) -> ()  [unwired: 2 in, 2 out]
        n411 = property on="量程选择" class="Enum (严格)"("Disabled Items []"=w644) -> ()  [unwired: 2 in, 2 out]
        n412 = property on="测量模式(公式)" class="Ring (严格)"("DisabledEnum"=w645) -> ()  [unwired: 2 in, 2 out]
      }
    }
    n413 = flat-sequence {
      frame #0 {
        # "公式读取显示（只在读取公式的时候改变一次）"
        n414 = global read "COD内部交互全局.vi" "读取公式显示"() -> (w376:bool)
        n415 = case shown="真" w376 {
          frame False {
          }
          frame True {
            n416 = global write "COD内部交互全局.vi" "读取公式显示"(FALSE ("读取参数显示")) -> ()
            n417 = global read "COD内部交互全局.vi" "读取公式"() -> (w386:u16[])
            n418 = Array Subset(array=w386, index=10 ("索引"), length=84 ("长度")) -> (w381:u16[])
            n419 = One Button Dialog(message="公式读取成功！" ("消息")) -> ()  [unwired: 1 in, 1 out]
            n420 = local read "测量模式(公式)"() -> (w384:u16)
            n421 = call "浮点CDAB转换COD.vi"("数组"=w381) -> ("数组 2"=w382:sgl[])  [unwired: 10 in]
            n422 = Array To Cluster(array=w382) -> (cluster=w385:T10)
            n423 = case shown="1" w384 {
              tunnel: [cluster{"X":dbl, "b":dbl, "X^2":dbl} {"X"=999.0, "b"=999.0, "X^2"=999.0} ("方程系数") w389 w408 w427 w446 w465 w484 w503] -> w383
              tunnel: w385 -> [_ w388 w407 w426 w445 w464 w483 w502]
              frame 0, Default {
              }
              frame 1 {
                n424 = local read "量程选择"() -> (w391:enum16{"低量程", "高量程", "0-2量程"})
                n425 = case shown="\"低量程\", 默认" w391 {
                  tunnel: w388 -> [w398 w402 w406]
                  tunnel: [w397 w401 w405] -> w394
                  tunnel: [w396 w400 w404] -> w393
                  tunnel: [w395 w399 w403] -> w392
                  frame "低量程", Default {
                    n426 = Unbundle By Name(w398) -> ("数组 2[0]"=w397:sgl, "数组 2[1]"=w396:sgl, "数组 2[2]"=w395:sgl)
                  }
                  frame "高量程" {
                    n427 = Unbundle By Name(w402) -> ("数组 2[3]"=w401:sgl, "数组 2[4]"=w400:sgl, "数组 2[5]"=w399:sgl)
                  }
                  frame "0-2量程" {
                    n428 = Unbundle By Name(w406) -> ("数组 2[6]"=w405:sgl, "数组 2[7]"=w404:sgl, "数组 2[8]"=w403:sgl)
                  }
                }
                n429 = Bundle By Name(cluster=cluster{"X":dbl, "b":dbl, "X^2":dbl} {"X"=0.0, "b"=0.0, "X^2"=0.0} ("方程系数"), "X"=w394, "b"=w393, "X^2"=w392) -> (w389:cluster{"X":dbl, "b":dbl, "X^2":dbl})
              }
              frame 2 {
                n430 = local read "量程选择"() -> (w410:enum16{"低量程", "高量程", "0-2量程"})
                n431 = case shown="\"高量程\"" w410 {
                  tunnel: w407 -> [w417 w421 w425]
                  tunnel: [w416 w420 w424] -> w413
                  tunnel: [w415 w419 w423] -> w412
                  tunnel: [w414 w418 w422] -> w411
                  frame "低量程", Default {
                    n432 = Unbundle By Name(w417) -> ("数组 2[6]"=w416:sgl, "数组 2[7]"=w415:sgl, "数组 2[8]"=w414:sgl)
                  }
                  frame "高量程" {
                    n433 = Unbundle By Name(w421) -> ("数组 2[9]"=w420:sgl, "数组 2[10]"=w419:sgl, "数组 2[11]"=w418:sgl)
                  }
                  frame "0-2量程" {
                    n434 = Unbundle By Name(w425) -> ("数组 2[6]"=w424:sgl, "数组 2[7]"=w423:sgl, "数组 2[8]"=w422:sgl)
                  }
                }
                n435 = Bundle By Name(cluster=cluster{"X":dbl, "b":dbl, "X^2":dbl} {"X"=0.0, "b"=0.0, "X^2"=0.0} ("方程系数"), "X"=w413, "b"=w412, "X^2"=w411) -> (w408:cluster{"X":dbl, "b":dbl, "X^2":dbl})
              }
              frame 3 {
                n436 = local read "量程选择"() -> (w429:enum16{"低量程", "高量程", "0-2量程"})
                n437 = case shown="\"高量程\"" w429 {
                  tunnel: w426 -> [w436 w440 w444]
                  tunnel: [w435 w439 w443] -> w432
                  tunnel: [w434 w438 w442] -> w431
                  tunnel: [w433 w437 w441] -> w430
                  frame "低量程", Default {
                    n438 = Unbundle By Name(w436) -> ("数组 2[12]"=w435:sgl, "数组 2[13]"=w434:sgl, "数组 2[14]"=w433:sgl)
                  }
                  frame "高量程" {
                    n439 = Unbundle By Name(w440) -> ("数组 2[15]"=w439:sgl, "数组 2[16]"=w438:sgl, "数组 2[17]"=w437:sgl)
                  }
                  frame "0-2量程" {
                    n440 = Unbundle By Name(w444) -> ("数组 2[6]"=w443:sgl, "数组 2[7]"=w442:sgl, "数组 2[8]"=w441:sgl)
                  }
                }
                n441 = Bundle By Name(cluster=cluster{"X":dbl, "b":dbl, "X^2":dbl} {"X"=0.0, "b"=0.0, "X^2"=0.0} ("方程系数"), "X"=w432, "b"=w431, "X^2"=w430) -> (w427:cluster{"X":dbl, "b":dbl, "X^2":dbl})
              }
              frame 4 {
                n442 = local read "量程选择"() -> (w448:enum16{"低量程", "高量程", "0-2量程"})
                n443 = case shown="\"高量程\"" w448 {
                  tunnel: w445 -> [w455 w459 w463]
                  tunnel: [w454 w458 w462] -> w451
                  tunnel: [w453 w457 w461] -> w450
                  tunnel: [w452 w456 w460] -> w449
                  frame "低量程", Default {
                    n444 = Unbundle By Name(w455) -> ("数组 2[18]"=w454:sgl, "数组 2[19]"=w453:sgl, "数组 2[20]"=w452:sgl)
                  }
                  frame "高量程" {
                    n445 = Unbundle By Name(w459) -> ("数组 2[21]"=w458:sgl, "数组 2[22]"=w457:sgl, "数组 2[23]"=w456:sgl)
                  }
                  frame "0-2量程" {
                    n446 = Unbundle By Name(w463) -> ("数组 2[6]"=w462:sgl, "数组 2[7]"=w461:sgl, "数组 2[8]"=w460:sgl)
                  }
                }
                n447 = Bundle By Name(cluster=cluster{"X":dbl, "b":dbl, "X^2":dbl} {"X"=0.0, "b"=0.0, "X^2"=0.0} ("方程系数"), "X"=w451, "b"=w450, "X^2"=w449) -> (w446:cluster{"X":dbl, "b":dbl, "X^2":dbl})
              }
              frame 5 {
                n448 = local read "量程选择"() -> (w467:enum16{"低量程", "高量程", "0-2量程"})
                n449 = case shown="\"高量程\"" w467 {
                  tunnel: w464 -> [w474 w478 w482]
                  tunnel: [w473 w477 w481] -> w470
                  tunnel: [w472 w476 w480] -> w469
                  tunnel: [w471 w475 w479] -> w468
                  frame "低量程", Default {
                    n450 = Unbundle By Name(w474) -> ("数组 2[24]"=w473:sgl, "数组 2[25]"=w472:sgl, "数组 2[26]"=w471:sgl)
                  }
                  frame "高量程" {
                    n451 = Unbundle By Name(w478) -> ("数组 2[27]"=w477:sgl, "数组 2[28]"=w476:sgl, "数组 2[29]"=w475:sgl)
                  }
                  frame "0-2量程" {
                    n452 = Unbundle By Name(w482) -> ("数组 2[6]"=w481:sgl, "数组 2[7]"=w480:sgl, "数组 2[8]"=w479:sgl)
                  }
                }
                n453 = Bundle By Name(cluster=cluster{"X":dbl, "b":dbl, "X^2":dbl} {"X"=0.0, "b"=0.0, "X^2"=0.0} ("方程系数"), "X"=w470, "b"=w469, "X^2"=w468) -> (w465:cluster{"X":dbl, "b":dbl, "X^2":dbl})
              }
              frame 6 {
                n454 = local read "量程选择"() -> (w486:enum16{"低量程", "高量程", "0-2量程"})
                n455 = case shown="\"高量程\"" w486 {
                  tunnel: w483 -> [w493 w497 w501]
                  tunnel: [w492 w496 w500] -> w489
                  tunnel: [w491 w495 w499] -> w488
                  tunnel: [w490 w494 w498] -> w487
                  frame "低量程", Default {
                    n456 = Unbundle By Name(w493) -> ("数组 2[30]"=w492:sgl, "数组 2[31]"=w491:sgl, "数组 2[32]"=w490:sgl)
                  }
                  frame "高量程" {
                    n457 = Unbundle By Name(w497) -> ("数组 2[33]"=w496:sgl, "数组 2[34]"=w495:sgl, "数组 2[35]"=w494:sgl)
                  }
                  frame "0-2量程" {
                    n458 = Unbundle By Name(w501) -> ("数组 2[6]"=w500:sgl, "数组 2[7]"=w499:sgl, "数组 2[8]"=w498:sgl)
                  }
                }
                n459 = Bundle By Name(cluster=cluster{"X":dbl, "b":dbl, "X^2":dbl} {"X"=0.0, "b"=0.0, "X^2"=0.0} ("方程系数"), "X"=w489, "b"=w488, "X^2"=w487) -> (w484:cluster{"X":dbl, "b":dbl, "X^2":dbl})
              }
              frame 7 {
                n460 = local read "量程选择"() -> (w505:enum16{"低量程", "高量程", "0-2量程"})
                n461 = case shown="\"高量程\"" w505 {
                  tunnel: w502 -> [w512 w516 w520]
                  tunnel: [w511 w515 w519] -> w508
                  tunnel: [w510 w514 w518] -> w507
                  tunnel: [w509 w513 w517] -> w506
                  frame "低量程", Default {
                    n462 = Unbundle By Name(w512) -> ("数组 2[36]"=w511:sgl, "数组 2[37]"=w510:sgl, "数组 2[38]"=w509:sgl)
                  }
                  frame "高量程" {
                    n463 = Unbundle By Name(w516) -> ("数组 2[39]"=w515:sgl, "数组 2[40]"=w514:sgl, "数组 2[41]"=w513:sgl)
                  }
                  frame "0-2量程" {
                    n464 = Unbundle By Name(w520) -> ("数组 2[6]"=w519:sgl, "数组 2[7]"=w518:sgl, "数组 2[8]"=w517:sgl)
                  }
                }
                n465 = Bundle By Name(cluster=cluster{"X":dbl, "b":dbl, "X^2":dbl} {"X"=0.0, "b"=0.0, "X^2"=0.0} ("方程系数"), "X"=w508, "b"=w507, "X^2"=w506) -> (w503:cluster{"X":dbl, "b":dbl, "X^2":dbl})
              }
            }
            n466 = local write "方程系数"(w383) -> ()
          }
        }
      }
    }
    n467 = Wait (ms)(milliseconds to wait=u32 1000 ("等待时间（毫秒）")) -> ()  [unwired: 1 out]
  }
  n468 = vi-ref "斯坦道CODMn.lvlib:待机状态数据存储写入和切换量程(子VI).vi"() -> (w37:refnum<vi>)
  n469 = vi-ref "斯坦道CODMn.lvlib:定时启动 (子VI).vi"() -> (w24:refnum<vi>)
  n470 = vi-ref "斯坦道CODMn.lvlib:日志报警状态存储 (子VI).vi"() -> (w23:refnum<vi>)
  n471 = vi-ref "斯坦道CODMn.lvlib:高锰酸钾-ORP滴定曲线(子VI).vi"() -> (w10:refnum<vi>)
  n472 = while {
    stop <- FALSE stop-if-true
    # "相差60秒自动校时"
    n473 = global read "运行时序全局变量.vi" "多列列表框"() -> (w669:i32)
    n474 = local read "仪器时间"() -> (w676:timestamp)
    n475 = local read "系统时间"() -> (w677:timestamp)
    n476 = Wait (ms)(milliseconds to wait=u32 1000 ("等待时间（毫秒）")) -> ()  [unwired: 1 out]
    n477 = Build Array(w676) -> (w675:timestamp[])
    n478 = Build Array(w677) -> (w694:timestamp[])
    n479 = Equal?(x=w669, y=u16 5) -> (x = y?=w671:bool)
    n480 = call <vilib>:"Boolean Crossing PtByPt.vi"("direction"=enum16{"either", "false-true", "true-false"}."false-true", "input"=w671) -> ("crossing"=w668:bool)  [unwired: 1 in]
    n481 = call "DateToHex.vi"("DATE"=w675) -> ("数组"=w688:u16[])  [unwired: 10 in]
    n482 = call "DateToHex.vi"("DATE"=w694) -> ("数组"=w693:u16[])  [unwired: 10 in]
    n483 = case shown="真" w668 {
      frame False {
      }
      frame True {
        # "校准结束后自动更新曲线泵滴定数"
        n484 = global read "COD测量模式全局.vi" "测量模式"() -> (w697:string)
        n485 = global read "CODMN外部API.vi" "远程反控校准CODMn"() -> (w699:bool)
        n486 = global read "COD测量模式全局.vi" "测量模式"() -> (w700:string)
        n487 = global read "COD内部交互全局.vi" "高锰酸钾"() -> (w703:dbl)
        n488 = Equal?(x=w697, y="校零") -> (x = y?=w695:bool)
        n489 = Equal?(x=w700, y="校标") -> (x = y?=w702:bool)
        n490 = Or(x=w695, y=w702) -> (x .or. y?=w698:bool)
        n491 = case shown="真" w698 {
          tunnel: w703 -> [_ w706]
          frame False {
          }
          frame True {
            n492 = global read "COD内部交互全局.vi" "当前校准"() -> (w705:i32)
            n493 = case shown="5" w705 {
              tunnel: w706 -> [w707 w708 w709 w710 w711]
              frame 1, Default {
                n494 = property on="泵滴定数1" class="DigNum (严格)"("Val(Sgnl)"=w707) -> ()  [unwired: 2 in, 2 out]
              }
              frame 2 {
                n495 = property on="泵滴定数2" class="DigNum (严格)"("Val(Sgnl)"=w708) -> ()  [unwired: 2 in, 2 out]
              }
              frame 3 {
                n496 = property on="泵滴定数3" class="DigNum (严格)"("Val(Sgnl)"=w709) -> ()  [unwired: 2 in, 2 out]
              }
              frame 4 {
                n497 = property on="泵滴定数4" class="DigNum (严格)"("Val(Sgnl)"=w710) -> ()  [unwired: 2 in, 2 out]
              }
              frame 5 {
                n498 = property on="泵滴定数5" class="DigNum (严格)"("Val(Sgnl)"=w711) -> ()  [unwired: 2 in, 2 out]
              }
            }
          }
        }
        n499 = case shown="真" w699 {
          frame False {
          }
          frame True {
            # "校准完自动写入公式"
            n500 = global write "CODMN外部API.vi" "远程反控校准CODMn"(FALSE ("远程反控校准CODMn")) -> ()
          }
        }
      }
    }
    n501 = Index Array(array=w688, index=2 ("索引")) -> (element=w690:u16)
    n502 = Index Array(array=w693, index=2 ("索引")) -> (element=w691:u16)
    n503 = Split Number(x=w690) -> (hi(x)=w684:u8)  [unwired: 1 out]
    n504 = Split Number(x=w691) -> (hi(x)=w687:u8)  [unwired: 1 out]
    n505 = To Byte Integer(number=w684) -> (8bit integer=w683:i8)
    n506 = To Byte Integer(number=w687) -> (8bit integer=w686:i8)
    n507 = Subtract(x=w683, y=w686) -> (x-y=w685:i8)
    n508 = Absolute Value(x=w685) -> (abs(x)=w682:i8)
    n509 = local read "通讯状态"() -> (w679:bool)
    n510 = Greater Or Equal?(x=w682, y=i8 5) -> (x >= y?=w680:bool)
    n511 = And(x=w680, y=w679) -> (x .and. y?=w678:bool)
    n512 = case shown="真" w678 {
      frame False {
      }
      frame True {
        # "相差60秒时间自动校准"
        n513 = flat-sequence {
          frame #0 {
            n514 = property on="时间校准" class="Bool (严格)"("Val(Sgnl)"=TRUE ("值(信号)")) -> ()  [unwired: 2 in, 2 out]
          }
          frame #1 {
            n515 = Wait (ms)(milliseconds to wait=u32 500 ("等待时间（毫秒）")) -> ()  [unwired: 1 out]
          }
          frame #2 {
            n516 = property on="时间校准" class="Bool (严格)"("Val(Sgnl)"=FALSE ("值(信号)")) -> ()  [unwired: 2 in, 2 out]
          }
        }
      }
    }
  }
  n517 = property class="VI"(reference=w24, error in=errorcluster {"status"=FALSE, "code"=0, "source"=""} ("错误输出")) -> ("Name"=w25:string)  [unwired: 2 out]
  n518 = property class="VI"(reference=w23, error in=errorcluster {"status"=FALSE, "code"=0, "source"=""} ("错误输出")) -> ("Name"=w22:string)  [unwired: 2 out]
  n519 = property class="VI"(reference=w10, error in=errorcluster {"status"=FALSE, "code"=0, "source"=""} ("错误输出")) -> ("Name"=w11:string)  [unwired: 2 out]
  n520 = Open VI Reference(type specifier VI Refnum (for type only)=refnum<vi> refnum, vi path=w25, options=128 ("选项")) -> (vi reference=w5:refnum<vi>, error out=w27:errorcluster)  [unwired: 3 in]
  n521 = property class="VI"(reference=w37, error in=errorcluster {"status"=FALSE, "code"=0, "source"=""} ("错误输出")) -> ("Name"=w36:string)  [unwired: 2 out]
  n522 = call-by-ref "?"(reference=w5, error in=w27) -> (reference out=w29:refnum<vi>, error out=w28:errorcluster)  [unwired: 12 in]
  n523 = Open VI Reference(type specifier VI Refnum (for type only)=refnum<vi> refnum, vi path=w22, options=128 ("选项")) -> (vi reference=w6:refnum<vi>, error out=w20:errorcluster)  [unwired: 3 in]
  n524 = Open VI Reference(type specifier VI Refnum (for type only)=refnum<vi> refnum, vi path=w11, options=128 ("选项")) -> (vi reference=w9:refnum<vi>, error out=w13:errorcluster)  [unwired: 3 in]
  n525 = call-by-ref "?"(reference=w6, error in=w20) -> (reference out=w18:refnum<vi>, error out=w19:errorcluster)  [unwired: 12 in]
  n526 = Close Reference(reference=w29, error in (no error)=w28) -> ()  [unwired: 1 out]
  n527 = call-by-ref "?"(reference=w9, error in=w13) -> (reference out=w15:refnum<vi>, error out=w14:errorcluster)  [unwired: 12 in]
  n528 = Open VI Reference(type specifier VI Refnum (for type only)=refnum<vi> refnum, vi path=w36, options=128 ("选项")) -> (vi reference=w2:refnum<vi>, error out=w34:errorcluster)  [unwired: 3 in]
  n529 = Close Reference(reference=w18, error in (no error)=w19) -> ()  [unwired: 1 out]
  n530 = call-by-ref "?"(reference=w2, error in=w34) -> (reference out=w32:refnum<vi>, error out=w33:errorcluster)  [unwired: 12 in]
  n531 = Close Reference(reference=w15, error in (no error)=w14) -> ()  [unwired: 1 out]
  n532 = Close Reference(reference=w32, error in (no error)=w33) -> ()  [unwired: 1 out]
  n533 = Obtain Queue(name (unnamed)="CODMn" ("名称（未命名）"), element data type=cluster{"命令":string} {"命令"="启用模块"} ("元素")) -> (queue out=w48:refnum<queue>, error out=w47:errorcluster)  [unwired: 3 in, 1 out]
  n534 = while {
    tunnel: [w722] -> _
    shift-right: [w720] -> _
    shift-left: _ -> [w719]
    tunnel: w1 -> [w716]
    stop <- FALSE stop-if-true
    n535 = global read "CODMN外部API.vi" "配置文件 path"() -> (w715:path)
    n536 = Wait (ms)(milliseconds to wait=u32 1000 ("等待时间（毫秒）")) -> ()  [unwired: 1 out]
    n537 = Get File Size(file=w715, error in=w716) -> (size (in bytes)=w720:i64, 0:w717:errorcluster)  [unwired: 1 out]
    n538 = Not Equal?(x=w720, y=w719) -> (x != y?=w718:bool)
    n539 = case shown="真" w718 {
      tunnel: [w724 w728] -> w722
      tunnel: w715 -> [_ w727]
      tunnel: w717 -> [w724 w726]
      frame False {
      }
      frame True {
        # "文件发生改变进行更新"
        n540 = vi-ref "斯坦道CODMn.lvlib:CODMn断电保存全局变量.vi"() -> (w725:refnum<vi>)
        n541 = call <vilib>:"Open Config Data.vi"("error in (no error)"=w726, "configuration file path"=w727) -> ("error out"=w732:errorcluster, "refnum"=w731:T6)  [unwired: 7 in, 1 out]
        n542 = call <userlib>:"Read Panel from INI__ogtk.vi"("error in (no error)"=w732, "VI ref"=w725, "refnum"=w731) -> ("error out"=w730:errorcluster, "refnum out"=w729:T6)  [unwired: 7 in]
        n543 = call <vilib>:"Close Config Data.vi"("error in (no error)"=w730, "refnum"=w729) -> ("error out"=w728:errorcluster)  [unwired: 8 in, 1 out]
      }
    }
  }
  n544 = vi-ref "CODMn通讯.vi"() -> (w39:refnum<vi>)
  n545 = while {
    tunnel: w48 -> [w742]
    tunnel: w47 -> [w741]
    tunnel: w1 -> [_]
    stop <- FALSE stop-if-true
    # "主循环界面显示"
    n546 = flat-sequence {
      frame #0 {
        # "A，B，K"
        # "CODMn读取状态"
        n547 = global read "COD内部交互全局.vi" "ORP、时间"() -> (w867:u16[])
        n548 = To Word Integer(number=w867) -> (16bit integer=w888:i16[])
        n549 = Split 1D Array(array=w888, index=3 ("索引")) -> (first subarray=w869:i16[], second subarray=w887:i16[])
        n550 = Index Array(array=w869) -> (element #1=w873:i16, element #2=w872:i16, element #3=w871:i16)  [unwired: 3 in]
        n551 = Index Array(array=w887) -> (element #1=w882:i16, element #2=w886:i16, element #3=w885:i16, element #4=w884:i16)  [unwired: 4 in]
        n552 = To Single Precision Float(number=w884) -> (single precision float=w875:sgl)
        n553 = Build Array(w873, w872, w871) -> (w870:i16[])
        n554 = To Single Precision Float(number=w882) -> (single precision float=w881:sgl)
        n555 = To Single Precision Float(number=w886) -> (single precision float=w880:sgl)
        n556 = To Single Precision Float(number=w885) -> (single precision float=w876:sgl)
        n557 = call "HexToDate.vi"("数组"=w870) -> ("DATE"=w874:timestamp[])  [unwired: 10 in]
        n558 = Number To Decimal String(number=w880) -> (decimal integer string=→"ORP-A":string)  [unwired: 1 in]
        n559 = Number To Decimal String(number=w876) -> (decimal integer string=→"ORP-B":string)  [unwired: 1 in]
        n560 = Number To Decimal String(number=w875) -> (decimal integer string=→"ORP-K":string)  [unwired: 1 in]
        n561 = Divide(x=w881, y=sgl 100.0) -> (x/y=→"COD浓度（mg/L)":sgl)
        n562 = Index Array(array=w874) -> (element=w868:timestamp)  [unwired: 1 in]
        n563 = Format Date/Time String(seconds (now)=w868) -> (date/time string=→"数据时间":string)  [unwired: 2 in]
      }
    }
    n564 = flat-sequence {
      frame #0 {
        # "测量状态显示"
        n565 = global read "COD内部交互全局.vi" "测量状态"() -> (w787:u16[])
        n566 = To Word Integer(number=w787) -> (16bit integer=w798:i16[])
        n567 = Index Array(array=w798, index #1=0 ("索引"), index #4=3 ("索引"), index #14=13 ("索引"), index #15=14 ("索引"), index #21=20 ("索引"), index #32=31 ("索引")) -> (element #1=w802:i16, element #2=w801:i16, element #3=w800:i16, element #4=→"CODMn工作状态":i16, element #5=→"模式（受控）":i16, element #6=→"进样管":i16, element #7=→"高锰酸钾":i16, element #8=→"草酸钠":i16, element #9=→"硫酸":i16, element #10=w797:i16, element #11=w817:i16, element #12=w793:i16, element #13=→"报警数字":i16, element #14=w823:i16, element #15=w808:i16, element #16=→"多列列表框":i16, element #21=w785:i16, element #33=→"分":i16, element #34=→"秒":i16)  [unwired: 28 in, 15 out]
        n568 = global write "COD内部交互全局.vi" "基本量程存储数据用"(w785) -> ()
        n569 = Build Array(w802, w801, w800) -> (w803:i16[])
        n570 = To Single Precision Float(number=w797) -> (single precision float=→"ORP显示":sgl)
        n571 = Number To Decimal String(number=w785) -> (decimal integer string=→"基本量程(显示)":string)  [unwired: 1 in]
        n572 = Equal?(x=w793, y=u16 1) -> (x = y?=→"排液标记":bool)
        n573 = Equal?(x=w793, y=u16 2) -> (x = y?=→"断电排液标记":bool)
        n574 = Divide(x=w817, y=u16 10) -> (x/y=→"温度":dbl)
        n575 = Divide(x=w823, y=u16 1000) -> (x/y=→"零点滴定值":dbl)
        n576 = Divide(x=w808, y=u16 1000) -> (x/y=→"标度滴定值":dbl)
        n577 = call "HexToDate.vi"("数组"=w803) -> ("DATE"=w799:timestamp[])  [unwired: 10 in]
        n578 = Index Array(array=w799) -> (element=→"仪器时间":timestamp)  [unwired: 1 in]
      }
    }
    n579 = flat-sequence {
      frame #0 {
        # "报警状态显示"
        n580 = global read "COD内部交互全局.vi" "报警点位"() -> (w840:bool[])
        n581 = Index Array(array=w840, index #1=0 ("索引")) -> (element #1=w837:bool, element #2=w836:bool, element #3=w835:bool, element #4=w834:bool, element #5=w833:bool, element #6=w832:bool, element #7=w831:bool, element #8=w830:bool, element #9=w829:bool, element #11=w828:bool, element #13=w827:bool, element #14=w826:bool)  [unwired: 13 in, 2 out]
        "ORP故障" <- w837
        "温控器故障" <- w836
        "加热故障" <- w829
        "高锰酸钾报警" <- w831
        "草酸钠报警" <- w830
        "测量错误" <- w835
        "校零错误" <- w834
        "校标错误" <- w833
        "进水样超量程" <- w832
        "排液故障" <- w828
        "60分钟超时报警" <- w827
        "进样无液体告警" <- w826
        n582 = Compound Arithmetic op=OR ("复合运算")(w837, w836, w829, w831, w830, w835, w833, w834, w832, w828, w827) -> (→"故障标记":bool)
        n583 = Bundle By Name(cluster=T11 {"ORP故障"=FALSE, "温控器故障"=FALSE, "加热故障"=FALSE, "高锰酸钾报警"=FALSE, "草酸钠报警"=FALSE, "测量错误"=FALSE, "校零错误"=FALSE, "校标错误"=FALSE, " 进水样超量程"=FALSE, "排液阀故障"=FALSE, "60分钟超时报警"=FALSE, "进样无液体报警"=FALSE} ("报警簇"), "ORP故障"=w837, "温控器故障"=w836, "加热故障"=w829, "高锰酸钾报警"=w831, "草酸钠报警"=w830, "测量错误"=w835, "校零错误"=w834, "校标错误"=w833, "进水样超量程"=w832, "排液阀故障"=w828, "60分钟超时报警"=w827, "进样无液体报警"=w826) -> (w838:T11)
        n584 = global write "COD内部交互全局.vi" "报警簇"(w838) -> ()
      }
    }
    n585 = flat-sequence {
      frame #0 {
        # "CODMn读取状态"
        n586 = global read "COD内部交互全局.vi" "温度"() -> (w864:bool[])
        n587 = global read "COD内部交互全局.vi" "M输出点"() -> (w863:bool[])
        n588 = Index Array(array=w864) -> (element=→"加热":bool)  [unwired: 1 in]
        n589 = Index Array(array=w863) -> (element #1=→"搅拌":bool, element #4=→"进水样":bool, element #5=→"进蒸馏水":bool, element #6=→"进标液":bool, element #7=→"进零点核查样":bool, element #8=→"进加标回收样":bool, element #9=→"进高锰酸钾":bool, element #10=→"进草酸钠":bool, element #11=→"进硫酸":bool)  [unwired: 11 in, 2 out]
      }
    }
    n590 = flat-sequence {
      frame #0 {
        # "工作状态显示"
        n591 = local read "CODMn工作状态"() -> (w752:T1)
        n592 = case shown="\"标样校准\"" w752 {
          tunnel: [_ u16 0 ("y") u16 1 ("y") u16 2 ("y") u16 3 ("y") u16 4 ("y") u16 6 ("y") _ u16 7 ("y") u16 8 ("y") u16 5 ("y")] -> w751
          frame "空闲", Default {
          }
          frame "水样测试" {
          }
          frame "标样核查" {
          }
          frame "零点核查" {
          }
          frame "跨度核查" {
          }
          frame "空白测试" {
          }
          frame "平行样测试" {
          }
          frame "质控样" {
          }
          frame "空白校准" {
          }
          frame "标样校准" {
          }
          frame "加标回收" {
          }
        }
        n593 = Equal?(x=w752, y=u16 8) -> (x = y?=→"校零标记":bool)
        n594 = Equal?(x=w752, y=u16 4) -> (x = y?=→"跨度核查标记":bool)
        n595 = Equal?(x=w752, y=u16 0) -> (x = y?=→"待机":bool)
        n596 = Equal?(x=w752, y=u16 3) -> (x = y?=→"零点核查标记":bool)
        n597 = Equal?(x=w752, y=u16 7) -> (x = y?=→"质控样测量":bool)
        n598 = Equal?(x=w752, y=u16 1) -> (x = y?=→"水样测量":bool)
        n599 = Equal?(x=w752, y=u16 2) -> (x = y?=→"标样核查标记":bool)
        n600 = Equal?(x=w752, y=u16 6) -> (x = y?=→"平行样测量":bool)
        n601 = Equal?(x=w752, y=u16 9) -> (x = y?=→"校标标记":bool)
        n602 = Equal?(x=w752, y=u16 5) -> (x = y?=→"空白测试标记":bool)
        n603 = Equal?(x=w752, y=u16 10) -> (x = y?=→"加标回收测量":bool)
        n604 = global write "COD内部交互全局.vi" "测量模式数字"(w751) -> ()
      }
    }
    n605 = Get Date/Time In Seconds() -> (seconds since 1Jan1904=→"系统时间":timestamp)
    n606 = First Call?() -> (First Call?: T/F=w740:bool)
    n607 = Wait (ms)(milliseconds to wait=u32 1000 ("等待时间（毫秒）")) -> ()  [unwired: 1 out]
    n608 = case shown="真" w740 {
      tunnel: w742 -> [w844 w849]
      tunnel: w741 -> [w843 w848]
      tunnel: [w844 w847] -> w738
      tunnel: [w843 w846] -> w737
      frame False {
      }
      frame True {
        n609 = Bundle By Name(cluster=cluster{"命令":string} {"命令"=""} ("元素"), "命令"="CODMn读取参数" ("名称（未命名）")) -> (w852:cluster{"命令":string})
        n610 = Enqueue Element(queue=w849, element=w852, timeout in ms (-1)=1000 ("超时毫秒(-1)"), error in (no error)=w848) -> (queue out=w847:refnum<queue>, error out=w846:errorcluster)  [unwired: 1 out]
      }
    }
    n611 = Get Queue Status(queue=w738, error in (no error)=w737) -> (queue out=w734:refnum<queue>, error out=w733:errorcluster, # elements in queue=w736:i32)  [unwired: 1 in, 5 out]
    n612 = Equal To 0?(x=w736) -> (x = 0?=w735:bool)
    n613 = case shown="真" w735 {
      tunnel: w734 -> [_ w746]
      tunnel: w733 -> [_ w745]
      frame False {
      }
      frame True {
        n614 = Bundle By Name(cluster=cluster{"命令":string} {"命令"=""} ("元素"), "命令"="CODMn读取" ("名称（未命名）")) -> (w748:cluster{"命令":string})
        n615 = Enqueue Element(queue=w746, element=w748, timeout in ms (-1)=1000 ("超时毫秒(-1)"), error in (no error)=w745) -> ()  [unwired: 3 out]
      }
    }
  }
  n616 = while {
    tunnel: w48 -> [w891]
    tunnel: w47 -> [w890]
    stop <- FALSE stop-if-true
    # "主线事件"
    n617 = event shown="[32] \"更新程序\": 值改变" {
      selector: _ -> [_ _ _ _ _ _ _ _ _ _ _ _ _ _ _ _ _ _ _ _ _ _ _ _ _ _ _ _ _ _ _ _ _ _]
      dyn-events: _ -> [_ _ _ _ _ _ _ _ _ _ _ _ _ _ _ _ _ _ _ _ _ _ _ _ _ _ _ _ _ _ _ _ _ _]
      timeout: _ -> [_ _ _ _ _ _ _ _ _ _ _ _ _ _ _ _ _ _ _ _ _ _ _ _ _ _ _ _ _ _ _ _ _ _]
      tunnel: w891 -> [_ _ _ _ _ w974 _ _ _ _ _ _ _ _ _ _ _ _ _ _ _ w1486 _ _ _ w1698 _ _ _ _ w1971 w1978 w2017 _]
      tunnel: w890 -> [_ _ _ _ _ w973 _ _ _ _ _ _ _ _ _ _ _ _ _ _ _ w1483 _ _ _ w1697 _ _ _ _ w1970 w1977 w2016 _]
      event "单步启动": Value Change {
        n618 = event-data() -> ()  [unwired: 1 in, 6 out]
        n619 = call "CODMn手动控制框.vi"() -> ()  [unwired: 12 in]
      }
      event "启动": Mouse Down {
        n620 = event-data() -> ()  [unwired: 1 in, 8 out]
        n621 = global read "COD内部交互全局.vi" "基本量程存储数据用"() -> (w894:enum16{"L", "H", "AUTO"})
        n622 = call "启动测量模式选择对话框.vi"("量程选择"=w894) -> ("量程选择输出"=w893:enum16{"L", "H", "AUTO"}, "启动选择输出"=w898:u16)  [unwired: 9 in]
        n623 = Not Equal?(x=w898, y=u16 8) -> (x != y?=w895:bool)
        n624 = Not Equal?(x=w898, y=u16 7) -> (x != y?=w896:bool)
        n625 = And(x=w896, y=w895) -> (x .and. y?=w900:bool)
        n626 = case shown="真" w900 {
          tunnel: w898 -> [_ w912]
          tunnel: w893 -> [_ w903]
          frame False {
            n627 = One Button Dialog(message="请到校准配置里面进行校准操作！" ("消息")) -> ()  [unwired: 1 in, 1 out]
          }
          frame True {
            n628 = Not Equal?(x=w912, y=u16 9) -> (x != y?=w907:bool)
            n629 = case shown="\"AUTO\"" w903 {
              tunnel: [w913 w917 errorcluster {"status"=FALSE, "code"=0, "source"=""} ("error out")] -> w902
              frame "L", Default {
                n630 = call "CODMnMB_api.vi"("STEP"=enum16{"open", "read", "write", "close"}."write", "values"=u16[] [0], "starting address"=u16 4276) -> ("error out"=w913:errorcluster)  [unwired: 6 in, 2 out]
              }
              frame "H" {
                n631 = call "CODMnMB_api.vi"("STEP"=enum16{"open", "read", "write", "close"}."write", "values"=u16[] [1], "starting address"=u16 4276) -> ("error out"=w917:errorcluster)  [unwired: 6 in, 2 out]
              }
              frame "AUTO" {
              }
            }
            n632 = global write "CODMN外部API.vi" "手动启动CODMn"(w907) -> ()
            n633 = case shown="1" w912 {
              tunnel: [u16 4608 ("address") u16 4608 ("address") u16 4608 ("address") u16 4608 ("address") u16 4608 ("address") u16 4608 ("address") u16 4608 ("address") u16 4608 ("address") u16 4608 ("address") u16 4608 ("address")] -> w905
              tunnel: [u16 1 ("address") u16 2 ("address") u16 3 ("address") u16 4 ("address") u16 5 ("address") u16 7 ("address") u16 6 ("address") u16 8 ("address") u16 9 ("address") u16 0 ("address")] -> w909
              frame 0 {
              }
              frame 1 {
              }
              frame 2 {
              }
              frame 3 {
              }
              frame 4 {
              }
              frame 5 {
              }
              frame 6 {
              }
              frame 7 {
              }
              frame 8 {
              }
              frame 9, Default {
              }
            }
            n634 = Insert Into Array(array=u16[] [] ("values"), index=0 ("索引"), new element=w909) -> (w904:u16[])
            n635 = call "CODMnMB_api.vi"("STEP"=enum16{"open", "read", "write", "close"}."write", "Error in"=w902, "values"=w904, "starting address"=w905) -> ()  [unwired: 5 in, 3 out]
          }
        }
      }
      event "停止": Value Change {
        n636 = event-data() -> ()  [unwired: 1 in, 6 out]
        n637 = Two Button Dialog(message="确认是否停止？" ("消息"), 1:"否" ("F按钮名称（“取消”）"), 2:"是" ("T按钮名称（“确定”）")) -> (T button?=w944:bool)
        n638 = case shown="真" w944 {
          frame False {
          }
          frame True {
            n639 = Obtain Notifier(name (unnamed)="CODMn" ("名称（未命名）"), notification data type=FALSE) -> (notifier out=w950:refnum<notifier>, error out=w948:errorcluster)  [unwired: 2 in, 1 out]
            n640 = Send Notification(notification=TRUE ("通知"), notifier=w950, error in (no error)=w948) -> (notifier out=w947:refnum<notifier>, error out=w946:errorcluster)
            n641 = Release Notifier(notifier=w947, error in (no error)=w946) -> ()  [unwired: 1 in, 3 out]
            n642 = call "CODMnMB_api.vi"("STEP"=enum16{"open", "read", "write", "close"}."write", "values"=u16[] [11], "starting address"=u16 4608) -> ()  [unwired: 6 in, 3 out]
          }
        }
      }
      event "手动控制": Value Change {
        n643 = event-data() -> ()  [unwired: 1 in, 6 out]
        n644 = call "数字密码键盘.vi"() -> ("NewNumber"=w956:sgl)  [unwired: 1 in]
        n645 = Equal?(x=w956, y=8.0) -> (x = y?=w957:bool)
        n646 = case shown="假" w957 {
          frame False {
            n647 = call "窗口弹出对话框(子VI).vi"("消息"="密码错误") -> ()  [unwired: 10 in, 1 out]
          }
          frame True {
          }
        }
      }
      event "锁定按钮": Mouse Down {
        n648 = event-data() -> ("CtlRef"=w962:refnum<vi>)  [unwired: 1 in, 7 out]
        n649 = property class="Bool (严格)"(reference=w962) -> ("Value"=w961:bool)  [unwired: 1 in, 2 out]
        n650 = case shown="真" w961 {
          selector: w961 -> [w963 _]
          tunnel: [w963 w964] -> w960
          frame False {
          }
          frame True {
            n651 = call "数字密码键盘.vi"() -> ("NewNumber"=w965:sgl)  [unwired: 1 in]
            n652 = Equal?(x=w965, y=8.0) -> (x = y?=w964:bool)
            n653 = case shown="假" w964 {
              selector: w964 -> [w968 _]
              frame False {
                n654 = local write "锁定按钮"(w968) -> ()
                n655 = One Button Dialog(message="密码错误!" ("消息")) -> ()  [unwired: 1 in, 1 out]
              }
              frame True {
                n656 = One Button Dialog(message="解锁成功!" ("消息")) -> ()  [unwired: 1 in, 1 out]
              }
            }
          }
        }
        "x = y?" <- w960
      }
      event "参数配置": Value Change {
        (unwired) u16 20 ("number of holding registers")
        (unwired) u16 4272 ("starting address")
        n657 = event-data() -> ()  [unwired: 1 in, 6 out]
        n658 = global read "CODMN外部API.vi" "ping"() -> (w971:bool)
        n659 = property on="窗格" class="Pane"("Origin"=T5 {"Horizontal"=0, "Vertical"=650} ("原点")) -> ()  [unwired: 2 in, 2 out]
        n660 = case shown="假" w971 {
          tunnel: [w986 w989] -> w970
          frame False {
            n661 = global read "COD内部交互全局.vi" "配置文件ini"() -> (w988:string)
            n662 = call <vilib>:"Application Directory.vi"() -> ("Application Directory"=w987:path)
            n663 = Build Path(base path=w987, name or relative path=w988) -> (appended path=w986:path)
          }
          frame True {
            n664 = global read "CODMN外部API.vi" "配置文件 path"() -> (w989:path)
          }
        }
        n665 = Bundle By Name(cluster=cluster{"命令":string} {"命令"=""} ("元素"), "命令"="CODMn读取参数" ("名称（未命名）")) -> (w975:cluster{"命令":string})
        n666 = call <vilib>:"Open Config Data.vi"("configuration file path"=w970) -> ("error out"=w981:errorcluster, "refnum"=w978:T6)  [unwired: 8 in, 1 out]
        n667 = Enqueue Element(queue=w974, element=w975, error in (no error)=w973) -> ()  [unwired: 1 in, 3 out]
        n668 = vi-ref "斯坦道CODMn.lvlib:CODMn断电保存全局变量.vi"() -> (w979:refnum<vi>)
        n669 = call <userlib>:"Read Panel from INI__ogtk.vi"("error in (no error)"=w981, "VI ref"=w979, "refnum"=w978) -> ("error out"=w982:errorcluster, "refnum out"=w980:T6)  [unwired: 7 in]
        n670 = call <vilib>:"Close Config Data.vi"("error in (no error)"=w982, "refnum"=w980) -> ("error out"=w983:errorcluster, "file path"=w984:path)  [unwired: 8 in]
        n671 = Open/Create/Replace File(file path (use dialog)=w984, error in=w983) -> (error out=w972:errorcluster)  [unwired: 4 in, 2 out]
        n672 = call <vilib>:"Clear Errors.vi"("error in (no error)"=w972) -> ()  [unwired: 5 in, 2 out]
      }
      event "保存": Mouse Down {
        n673 = event-data() -> ()  [unwired: 1 in, 8 out]
        n674 = local read "通讯状态"() -> (w990:bool)
        n675 = Two Button Dialog(message="确定保存参数，保存参数将会替换原有参数！" ("消息")) -> (T button?=w992:bool)  [unwired: 2 in]
        n676 = case shown="真" w992 {
          tunnel: w990 -> [_ w993]
          frame False {
          }
          frame True {
            n677 = case shown="真" w993 {
              frame False {
                n678 = One Button Dialog(message="保存失败，当前无通讯！" ("消息")) -> ()  [unwired: 1 in, 1 out]
              }
              frame True {
                n679 = One Button Dialog(message="参数保存成功！" ("消息")) -> ()  [unwired: 1 in, 1 out]
                n680 = Build Array("采水泵进样时间/s:", "采水泵润洗时间/s:", "采水泵沉淀时间/s:", "采水泵排液时间/s:") -> (w996:i32[])
                n681 = call "CODMnMB_api.vi"("STEP"=enum16{"open", "read", "write", "close"}."write", "values"="保存参数", "starting address"=u16 4272) -> ("error out"=w1002:errorcluster)  [unwired: 6 in, 2 out]
                n682 = call "CODMnMB_api.vi"("STEP"=enum16{"open", "read", "write", "close"}."write", "Error in"=w1002, "values"=w996, "starting address"=u16 5596) -> ()  [unwired: 5 in, 3 out]
              }
            }
          }
        }
      }
      event "常规版/认证版": Value Change {
        n683 = event-data() -> ()  [unwired: 1 in, 6 out]
        n684 = flat-sequence {
          frame #0 {
            n685 = global write "CODMn断电保存全局变量.vi" "常规版/认证版"("常规版/认证版") -> ()
          }
          frame #1 {
            n686 = global read "CODMN外部API.vi" "ping"() -> (w1009:bool)
            n687 = case shown="假" w1009 {
              tunnel: [w1021 w1024] -> w1008
              frame False {
                n688 = global read "COD内部交互全局.vi" "配置文件ini"() -> (w1023:string)
                n689 = call <vilib>:"Application Directory.vi"() -> ("Application Directory"=w1022:path)
                n690 = Build Path(base path=w1022, name or relative path=w1023) -> (appended path=w1021:path)
              }
              frame True {
                n691 = global read "CODMN外部API.vi" "配置文件 path"() -> (w1024:path)
              }
            }
            n692 = call <vilib>:"Open Config Data.vi"("configuration file path"=w1008) -> ("error out"=w1017:errorcluster, "refnum"=w1020:T6)  [unwired: 8 in, 1 out]
            n693 = vi-ref "斯坦道CODMn.lvlib:CODMn断电保存全局变量.vi"() -> (w1019:refnum<vi>)
            n694 = call <userlib>:"Write Panel to INI__ogtk.vi"("error in (no error)"=w1017, "VI ref"=w1019, "refnum"=w1020) -> ("error out"=w1016:errorcluster, "refnum out"=w1018:T6)  [unwired: 7 in]
            n695 = call <vilib>:"Close Config Data.vi"("error in (no error)"=w1016, "refnum"=w1018) -> ("error out"=w1011:errorcluster, "file path"=w1010:path)  [unwired: 8 in]
            n696 = Open/Create/Replace File(file path (use dialog)=w1010, error in=w1011) -> (refnum out=w1014:refnum<file>, error out=w1015:errorcluster)  [unwired: 4 in, 1 out]
            n697 = Flush File(refnum=w1014, error in=w1015) -> (refnum out=w1013:refnum<file>, error out=w1012:errorcluster)
            n698 = Close File(refnum=w1013, error in=w1012) -> ()  [unwired: 2 out]
          }
        }
      }
      event "校准配置": Value Change {
        n699 = event-data() -> ()  [unwired: 1 in, 6 out]
        n700 = global read "CODMN外部API.vi" "ping"() -> (w1026:bool)
        n701 = property on="窗格" class="Pane"("Origin"=T5 {"Horizontal"=0, "Vertical"=1300} ("原点")) -> ()  [unwired: 2 in, 2 out]
        n702 = case shown="假" w1026 {
          tunnel: [w1107 w1110] -> w1025
          frame False {
            n703 = global read "COD内部交互全局.vi" "配置文件ini"() -> (w1109:string)
            n704 = call <vilib>:"Application Directory.vi"() -> ("Application Directory"=w1108:path)
            n705 = Build Path(base path=w1108, name or relative path=w1109) -> (appended path=w1107:path)
          }
          frame True {
            n706 = global read "CODMN外部API.vi" "配置文件 path"() -> (w1110:path)
          }
        }
        n707 = call <vilib>:"Open Config Data.vi"("configuration file path"=w1025) -> ("error out"=w1045:errorcluster, "refnum"=w1046:T6)  [unwired: 8 in, 1 out]
        n708 = call-poly <vilib>:"Read Key.vi"("section"="CODMn模型选择" ("key"), "error in (no error)"=w1045, "key"="线性和多项式", "refnum"=w1046) -> ("error out"=w1042:errorcluster, "value"=w1044:i32, "refnum out"=w1043:T6)  [unwired: 4 in, 1 out]
        n709 = local write "模型"(w1044) -> ()
        n710 = call-poly <vilib>:"Read Key.vi"("section"="标线选择", "error in (no error)"=w1042, "key"="选用水样", "refnum"=w1043) -> ("error out"=w1040:errorcluster, "value"=w1027:i32, "refnum out"=w1041:T6)  [unwired: 4 in, 1 out]
        n711 = local write "选用水样"(w1027) -> ()
        n712 = case shown="0, 默认" w1027 {
          tunnel: ["葡萄糖标线" ("section") "草酸钠标线" ("section")] -> w1051
          frame 0, Default {
          }
          frame 1 {
          }
        }
        n713 = local read "量程选择"() -> (w1052:enum16{"低量程", "高量程", "0-2量程"})
        n714 = case shown="\"0-2量程\"" w1052 {
          tunnel: ["低量程" "高量程" "0-2量程"] -> w1050
          frame "低量程", Default {
          }
          frame "高量程" {
          }
          frame "0-2量程" {
          }
        }
        n715 = Concatenate Strings(w1051, w1050) -> (w1049:string)
        n716 = call-poly <vilib>:"Read Key.vi"("section"=w1049, "error in (no error)"=w1040, "key"="浓度1", "refnum"=w1041) -> ("error out"=w1077:errorcluster, "value"=w1075:dbl, "refnum out"=w1076:T6)  [unwired: 4 in, 1 out]
        n717 = local write "浓度1"(w1075) -> ()
        n718 = call-poly <vilib>:"Read Key.vi"("section"=w1049, "error in (no error)"=w1077, "key"="浓度2", "refnum"=w1076) -> ("error out"=w1091:errorcluster, "value"=w1078:dbl, "refnum out"=w1090:T6)  [unwired: 4 in, 1 out]
        n719 = local write "浓度2"(w1078) -> ()
        n720 = call-poly <vilib>:"Read Key.vi"("section"=w1049, "error in (no error)"=w1091, "key"="浓度3", "refnum"=w1090) -> ("error out"=w1092:errorcluster, "value"=w1080:dbl, "refnum out"=w1089:T6)  [unwired: 4 in, 1 out]
        n721 = local write "浓度3"(w1080) -> ()
        n722 = call-poly <vilib>:"Read Key.vi"("section"=w1049, "error in (no error)"=w1092, "key"="泵滴定数1", "refnum"=w1089) -> ("error out"=w1093:errorcluster, "value"=w1082:dbl, "refnum out"=w1088:T6)  [unwired: 4 in, 1 out]
        n723 = local write "泵滴定数1"(w1082) -> ()
        n724 = call-poly <vilib>:"Read Key.vi"("section"=w1049, "error in (no error)"=w1093, "key"="泵滴定数2", "refnum"=w1088) -> ("error out"=w1087:errorcluster, "value"=w1085:dbl, "refnum out"=w1094:T6)  [unwired: 4 in, 1 out]
        n725 = local write "泵滴定数2"(w1085) -> ()
        n726 = call-poly <vilib>:"Read Key.vi"("section"=w1049, "error in (no error)"=w1087, "key"="泵滴定数3", "refnum"=w1094) -> ("error out"=w1099:errorcluster, "value"=w1098:dbl, "refnum out"=w1095:T6)  [unwired: 4 in, 1 out]
        n727 = local write "泵滴定数3"(w1098) -> ()
        n728 = call-poly <vilib>:"Read Key.vi"("section"=w1049, "error in (no error)"=w1099, "key"="浓度4", "refnum"=w1095) -> ("error out"=w1100:errorcluster, "value"=w1033:dbl, "refnum out"=w1096:T6)  [unwired: 4 in, 1 out]
        n729 = local write "浓度4"(w1033) -> ()
        n730 = call-poly <vilib>:"Read Key.vi"("section"=w1049, "error in (no error)"=w1100, "key"="浓度5", "refnum"=w1096) -> ("error out"=w1038:errorcluster, "value"=w1032:dbl, "refnum out"=w1039:T6)  [unwired: 4 in, 1 out]
        n731 = local write "浓度5"(w1032) -> ()
        n732 = call-poly <vilib>:"Read Key.vi"("section"=w1049, "error in (no error)"=w1038, "key"="泵滴定数4", "refnum"=w1039) -> ("error out"=w1101:errorcluster, "value"=w1031:dbl, "refnum out"=w1097:T6)  [unwired: 4 in, 1 out]
        n733 = local write "泵滴定数4"(w1031) -> ()
        n734 = call-poly <vilib>:"Read Key.vi"("section"=w1049, "error in (no error)"=w1101, "key"="泵滴定数5", "refnum"=w1097) -> ("error out"=w1036:errorcluster, "value"=w1030:dbl, "refnum out"=w1037:T6)  [unwired: 4 in, 1 out]
        n735 = local write "泵滴定数5"(w1030) -> ()
        n736 = call-poly <vilib>:"Read Key.vi"("section"=w1049, "error in (no error)"=w1036, "key"="当前选用的校准", "refnum"=w1037) -> ("error out"=w1071:errorcluster, "refnum out"=w1072:T6)  [unwired: 4 in, 2 out]
        n737 = call-poly <vilib>:"Read Key.vi"("section"=w1049, "error in (no error)"=w1071, "key"="启用1", "refnum"=w1072) -> ("error out"=w1068:errorcluster, "value"=w1057:bool, "refnum out"=w1069:T6)  [unwired: 4 in, 1 out]
        n738 = local write "启用1"(w1057) -> ()
        n739 = call-poly <vilib>:"Read Key.vi"("section"=w1049, "error in (no error)"=w1068, "key"="启用2", "refnum"=w1069) -> ("error out"=w1066:errorcluster, "value"=w1056:bool, "refnum out"=w1067:T6)  [unwired: 4 in, 1 out]
        n740 = local write "启用2"(w1056) -> ()
        n741 = call-poly <vilib>:"Read Key.vi"("section"=w1049, "error in (no error)"=w1066, "key"="启用3", "refnum"=w1067) -> ("error out"=w1064:errorcluster, "value"=w1055:bool, "refnum out"=w1065:T6)  [unwired: 4 in, 1 out]
        n742 = local write "启用3"(w1055) -> ()
        n743 = call-poly <vilib>:"Read Key.vi"("section"=w1049, "error in (no error)"=w1064, "key"="启用4", "refnum"=w1065) -> ("error out"=w1062:errorcluster, "value"=w1029:bool, "refnum out"=w1063:T6)  [unwired: 4 in, 1 out]
        n744 = local write "启用4"(w1029) -> ()
        n745 = call-poly <vilib>:"Read Key.vi"("section"=w1049, "error in (no error)"=w1062, "key"="启用5", "refnum"=w1063) -> ("error out"=w1034:errorcluster, "value"=w1028:bool, "refnum out"=w1035:T6)  [unwired: 4 in, 1 out]
        n746 = local write "启用5"(w1028) -> ()
        n747 = call <vilib>:"Close Config Data.vi"("error in (no error)"=w1034, "refnum"=w1035) -> ()  [unwired: 8 in, 2 out]
      }
      event "选用水样": Value Change {
        (unwired) "浓度6" ("key")
        n748 = event-data() -> ()  [unwired: 1 in, 6 out]
        n749 = local read "量程选择"() -> (w1131:enum16{"低量程", "高量程", "0-2量程"})
        n750 = property on="窗格" class="Pane"("Origin"=T5 {"Horizontal"=0, "Vertical"=1300} ("原点")) -> ()  [unwired: 2 in, 2 out]
        n751 = case shown="\"葡萄糖\", 默认" "选用水样" {
          tunnel: ["葡萄糖标线" ("section") "草酸钠标线" ("section")] -> w1133
          frame "葡萄糖", Default {
          }
          frame "草酸钠" {
          }
        }
        n752 = global read "CODMN外部API.vi" "ping"() -> (w1117:bool)
        n753 = case shown="\"0-2量程\"" w1131 {
          tunnel: ["低量程" "高量程" "0-2量程"] -> w1132
          frame "低量程", Default {
          }
          frame "高量程" {
          }
          frame "0-2量程" {
          }
        }
        n754 = case shown="假" w1117 {
          tunnel: [w1189 w1192] -> w1116
          frame False {
            n755 = global read "COD内部交互全局.vi" "配置文件ini"() -> (w1191:string)
            n756 = call <vilib>:"Application Directory.vi"() -> ("Application Directory"=w1190:path)
            n757 = Build Path(base path=w1190, name or relative path=w1191) -> (appended path=w1189:path)
          }
          frame True {
            n758 = global read "CODMN外部API.vi" "配置文件 path"() -> (w1192:path)
          }
        }
        n759 = Concatenate Strings(w1133, w1132) -> (w1130:string)
        n760 = call <vilib>:"Open Config Data.vi"("configuration file path"=w1116) -> ("error out"=w1154:errorcluster, "refnum"=w1155:T6)  [unwired: 8 in, 1 out]
        n761 = call-poly <vilib>:"Read Key.vi"("section"=w1130, "error in (no error)"=w1154, "key"="浓度1", "refnum"=w1155) -> ("error out"=w1159:errorcluster, "value"=w1157:dbl, "refnum out"=w1158:T6)  [unwired: 4 in, 1 out]
        n762 = local write "浓度1"(w1157) -> ()
        n763 = call-poly <vilib>:"Read Key.vi"("section"=w1130, "error in (no error)"=w1159, "key"="浓度2", "refnum"=w1158) -> ("error out"=w1173:errorcluster, "value"=w1160:dbl, "refnum out"=w1172:T6)  [unwired: 4 in, 1 out]
        n764 = local write "浓度2"(w1160) -> ()
        n765 = call-poly <vilib>:"Read Key.vi"("section"=w1130, "error in (no error)"=w1173, "key"="浓度3", "refnum"=w1172) -> ("error out"=w1174:errorcluster, "value"=w1162:dbl, "refnum out"=w1171:T6)  [unwired: 4 in, 1 out]
        n766 = local write "浓度3"(w1162) -> ()
        n767 = call-poly <vilib>:"Read Key.vi"("section"=w1130, "error in (no error)"=w1174, "key"="泵滴定数1", "refnum"=w1171) -> ("error out"=w1175:errorcluster, "value"=w1164:dbl, "refnum out"=w1170:T6)  [unwired: 4 in, 1 out]
        n768 = local write "泵滴定数1"(w1164) -> ()
        n769 = call-poly <vilib>:"Read Key.vi"("section"=w1130, "error in (no error)"=w1175, "key"="泵滴定数2", "refnum"=w1170) -> ("error out"=w1169:errorcluster, "value"=w1167:dbl, "refnum out"=w1176:T6)  [unwired: 4 in, 1 out]
        n770 = local write "泵滴定数2"(w1167) -> ()
        n771 = call-poly <vilib>:"Read Key.vi"("section"=w1130, "error in (no error)"=w1169, "key"="泵滴定数3", "refnum"=w1176) -> ("error out"=w1181:errorcluster, "value"=w1180:dbl, "refnum out"=w1177:T6)  [unwired: 4 in, 1 out]
        n772 = local write "泵滴定数3"(w1180) -> ()
        n773 = call-poly <vilib>:"Read Key.vi"("section"=w1130, "error in (no error)"=w1181, "key"="浓度4", "refnum"=w1177) -> ("error out"=w1182:errorcluster, "value"=w1125:dbl, "refnum out"=w1178:T6)  [unwired: 4 in, 1 out]
        n774 = local write "浓度4"(w1125) -> ()
        n775 = call-poly <vilib>:"Read Key.vi"("section"=w1130, "error in (no error)"=w1182, "key"="浓度5", "refnum"=w1178) -> ("error out"=w1128:errorcluster, "value"=w1124:dbl, "refnum out"=w1129:T6)  [unwired: 4 in, 1 out]
        n776 = local write "浓度5"(w1124) -> ()
        n777 = call-poly <vilib>:"Read Key.vi"("section"=w1130, "error in (no error)"=w1128, "key"="泵滴定数4", "refnum"=w1129) -> ("error out"=w1183:errorcluster, "value"=w1123:dbl, "refnum out"=w1179:T6)  [unwired: 4 in, 1 out]
        n778 = local write "泵滴定数4"(w1123) -> ()
        n779 = call-poly <vilib>:"Read Key.vi"("section"=w1130, "error in (no error)"=w1183, "key"="泵滴定数5", "refnum"=w1179) -> ("error out"=w1126:errorcluster, "value"=w1122:dbl, "refnum out"=w1127:T6)  [unwired: 4 in, 1 out]
        n780 = local write "泵滴定数5"(w1122) -> ()
        n781 = call-poly <vilib>:"Read Key.vi"("section"=w1130, "error in (no error)"=w1126, "key"="当前选用的校准", "refnum"=w1127) -> ("error out"=w1151:errorcluster, "refnum out"=w1152:T6)  [unwired: 4 in, 2 out]
        n782 = call-poly <vilib>:"Read Key.vi"("section"=w1130, "error in (no error)"=w1151, "key"="启用1", "refnum"=w1152) -> ("error out"=w1148:errorcluster, "value"=w1137:bool, "refnum out"=w1149:T6)  [unwired: 4 in, 1 out]
        n783 = local write "启用1"(w1137) -> ()
        n784 = call-poly <vilib>:"Read Key.vi"("section"=w1130, "error in (no error)"=w1148, "key"="启用2", "refnum"=w1149) -> ("error out"=w1146:errorcluster, "value"=w1136:bool, "refnum out"=w1147:T6)  [unwired: 4 in, 1 out]
        n785 = local write "启用2"(w1136) -> ()
        n786 = call-poly <vilib>:"Read Key.vi"("section"=w1130, "error in (no error)"=w1146, "key"="启用3", "refnum"=w1147) -> ("error out"=w1144:errorcluster, "value"=w1135:bool, "refnum out"=w1145:T6)  [unwired: 4 in, 1 out]
        n787 = local write "启用3"(w1135) -> ()
        n788 = call-poly <vilib>:"Read Key.vi"("section"=w1130, "error in (no error)"=w1144, "key"="启用4", "refnum"=w1145) -> ("error out"=w1142:errorcluster, "value"=w1119:bool, "refnum out"=w1143:T6)  [unwired: 4 in, 1 out]
        n789 = local write "启用4"(w1119) -> ()
        n790 = call-poly <vilib>:"Read Key.vi"("section"=w1130, "error in (no error)"=w1142, "key"="启用5", "refnum"=w1143) -> ("error out"=w1120:errorcluster, "value"=w1118:bool, "refnum out"=w1121:T6)  [unwired: 4 in, 1 out]
        n791 = local write "启用5"(w1118) -> ()
        n792 = call <vilib>:"Close Config Data.vi"("error in (no error)"=w1120, "refnum"=w1121) -> ()  [unwired: 8 in, 2 out]
      }
      event "量程选择": Value Change {
        n793 = event-data() -> ()  [unwired: 1 in, 6 out]
        n794 = local read "选用水样"() -> (w1216:enum16{"葡萄糖", "草酸钠"})
        n795 = property on="窗格" class="Pane"("Origin"=T5 {"Horizontal"=0, "Vertical"=1300} ("原点")) -> ()  [unwired: 2 in, 2 out]
        n796 = case shown="\"葡萄糖\", 默认" w1216 {
          tunnel: ["葡萄糖标线" ("section") "草酸钠标线" ("section")] -> w1215
          frame "葡萄糖", Default {
          }
          frame "草酸钠" {
          }
        }
        n797 = case shown="\"0-2量程\"" "量程选择" {
          tunnel: ["低量程" "高量程" "0-2量程"] -> w1212
          frame "低量程", Default {
          }
          frame "高量程" {
          }
          frame "0-2量程" {
          }
        }
        n798 = global read "CODMN外部API.vi" "ping"() -> (w1199:bool)
        n799 = case shown="假" w1199 {
          tunnel: [w1271 w1274] -> w1198
          frame False {
            n800 = global read "COD内部交互全局.vi" "配置文件ini"() -> (w1273:string)
            n801 = call <vilib>:"Application Directory.vi"() -> ("Application Directory"=w1272:path)
            n802 = Build Path(base path=w1272, name or relative path=w1273) -> (appended path=w1271:path)
          }
          frame True {
            n803 = global read "CODMN外部API.vi" "配置文件 path"() -> (w1274:path)
          }
        }
        n804 = Concatenate Strings(w1215, w1212) -> (w1214:string)
        n805 = call <vilib>:"Open Config Data.vi"("configuration file path"=w1198) -> ("error out"=w1236:errorcluster, "refnum"=w1237:T6)  [unwired: 8 in, 1 out]
        n806 = call-poly <vilib>:"Read Key.vi"("section"=w1214, "error in (no error)"=w1236, "key"="浓度1", "refnum"=w1237) -> ("error out"=w1241:errorcluster, "value"=w1239:dbl, "refnum out"=w1240:T6)  [unwired: 4 in, 1 out]
        n807 = local write "浓度1"(w1239) -> ()
        n808 = call-poly <vilib>:"Read Key.vi"("section"=w1214, "error in (no error)"=w1241, "key"="浓度2", "refnum"=w1240) -> ("error out"=w1255:errorcluster, "value"=w1242:dbl, "refnum out"=w1254:T6)  [unwired: 4 in, 1 out]
        n809 = local write "浓度2"(w1242) -> ()
        n810 = call-poly <vilib>:"Read Key.vi"("section"=w1214, "error in (no error)"=w1255, "key"="浓度3", "refnum"=w1254) -> ("error out"=w1256:errorcluster, "value"=w1244:dbl, "refnum out"=w1253:T6)  [unwired: 4 in, 1 out]
        n811 = local write "浓度3"(w1244) -> ()
        n812 = call-poly <vilib>:"Read Key.vi"("section"=w1214, "error in (no error)"=w1256, "key"="泵滴定数1", "refnum"=w1253) -> ("error out"=w1257:errorcluster, "value"=w1246:dbl, "refnum out"=w1252:T6)  [unwired: 4 in, 1 out]
        n813 = local write "泵滴定数1"(w1246) -> ()
        n814 = call-poly <vilib>:"Read Key.vi"("section"=w1214, "error in (no error)"=w1257, "key"="泵滴定数2", "refnum"=w1252) -> ("error out"=w1251:errorcluster, "value"=w1249:dbl, "refnum out"=w1258:T6)  [unwired: 4 in, 1 out]
        n815 = local write "泵滴定数2"(w1249) -> ()
        n816 = call-poly <vilib>:"Read Key.vi"("section"=w1214, "error in (no error)"=w1251, "key"="泵滴定数3", "refnum"=w1258) -> ("error out"=w1263:errorcluster, "value"=w1262:dbl, "refnum out"=w1259:T6)  [unwired: 4 in, 1 out]
        n817 = local write "泵滴定数3"(w1262) -> ()
        n818 = call-poly <vilib>:"Read Key.vi"("section"=w1214, "error in (no error)"=w1263, "key"="浓度4", "refnum"=w1259) -> ("error out"=w1264:errorcluster, "value"=w1203:dbl, "refnum out"=w1260:T6)  [unwired: 4 in, 1 out]
        n819 = local write "浓度4"(w1203) -> ()
        n820 = call-poly <vilib>:"Read Key.vi"("section"=w1214, "error in (no error)"=w1264, "key"="浓度5", "refnum"=w1260) -> ("error out"=w1210:errorcluster, "value"=w1202:dbl, "refnum out"=w1211:T6)  [unwired: 4 in, 1 out]
        n821 = local write "浓度5"(w1202) -> ()
        n822 = call-poly <vilib>:"Read Key.vi"("section"=w1214, "error in (no error)"=w1210, "key"="泵滴定数4", "refnum"=w1211) -> ("error out"=w1265:errorcluster, "value"=w1201:dbl, "refnum out"=w1261:T6)  [unwired: 4 in, 1 out]
        n823 = local write "泵滴定数4"(w1201) -> ()
        n824 = call-poly <vilib>:"Read Key.vi"("section"=w1214, "error in (no error)"=w1265, "key"="泵滴定数5", "refnum"=w1261) -> ("error out"=w1208:errorcluster, "value"=w1200:dbl, "refnum out"=w1209:T6)  [unwired: 4 in, 1 out]
        n825 = local write "泵滴定数5"(w1200) -> ()
        n826 = call-poly <vilib>:"Read Key.vi"("section"=w1214, "error in (no error)"=w1208, "key"="当前选用的校准", "refnum"=w1209) -> ("error out"=w1233:errorcluster, "refnum out"=w1234:T6)  [unwired: 4 in, 2 out]
        n827 = call-poly <vilib>:"Read Key.vi"("section"=w1214, "error in (no error)"=w1233, "key"="启用1", "refnum"=w1234) -> ("error out"=w1230:errorcluster, "value"=w1219:bool, "refnum out"=w1231:T6)  [unwired: 4 in, 1 out]
        n828 = local write "启用1"(w1219) -> ()
        n829 = call-poly <vilib>:"Read Key.vi"("section"=w1214, "error in (no error)"=w1230, "key"="启用2", "refnum"=w1231) -> ("error out"=w1228:errorcluster, "value"=w1218:bool, "refnum out"=w1229:T6)  [unwired: 4 in, 1 out]
        n830 = local write "启用2"(w1218) -> ()
        n831 = call-poly <vilib>:"Read Key.vi"("section"=w1214, "error in (no error)"=w1228, "key"="启用3", "refnum"=w1229) -> ("error out"=w1226:errorcluster, "value"=w1217:bool, "refnum out"=w1227:T6)  [unwired: 4 in, 1 out]
        n832 = local write "启用3"(w1217) -> ()
        n833 = call-poly <vilib>:"Read Key.vi"("section"=w1214, "error in (no error)"=w1226, "key"="启用4", "refnum"=w1227) -> ("error out"=w1224:errorcluster, "value"=w1205:bool, "refnum out"=w1225:T6)  [unwired: 4 in, 1 out]
        n834 = local write "启用4"(w1205) -> ()
        n835 = call-poly <vilib>:"Read Key.vi"("section"=w1214, "error in (no error)"=w1224, "key"="启用5", "refnum"=w1225) -> ("error out"=w1206:errorcluster, "value"=w1204:bool, "refnum out"=w1207:T6)  [unwired: 4 in, 1 out]
        n836 = local write "启用5"(w1204) -> ()
        n837 = call <vilib>:"Close Config Data.vi"("error in (no error)"=w1206, "refnum"=w1207) -> ()  [unwired: 8 in, 2 out]
      }
      event "返回": Value Change {
        w1295 = "CODMn" ("section")
        n838 = event-data() -> ()  [unwired: 1 in, 6 out]
        n839 = property on="窗格" class="Pane"("Origin"=T5 {"Horizontal"=0, "Vertical"=0} ("原点")) -> ()  [unwired: 2 in, 2 out]
        n840 = global read "CODMN外部API.vi" "ping"() -> (w1281:bool)
        n841 = case shown="假" w1281 {
          tunnel: [w1346 w1349] -> w1280
          frame False {
            n842 = global read "COD内部交互全局.vi" "配置文件ini"() -> (w1348:string)
            n843 = call <vilib>:"Application Directory.vi"() -> ("Application Directory"=w1347:path)
            n844 = Build Path(base path=w1347, name or relative path=w1348) -> (appended path=w1346:path)
          }
          frame True {
            n845 = global read "CODMN外部API.vi" "配置文件 path"() -> (w1349:path)
          }
        }
        n846 = call <vilib>:"Open Config Data.vi"("configuration file path"=w1280) -> ("error out"=w1344:errorcluster, "refnum"=w1345:T6)  [unwired: 8 in, 1 out]
        n847 = local read "浓度1"() -> (w1342:dbl)
        n848 = call-poly <vilib>:"Write Key.vi"("section"=w1295, "error in (no error)"=w1344, "value"=w1342, "key"="浓度1", "refnum"=w1345) -> ("error out"=w1341:errorcluster, "refnum out"=w1340:T6)  [unwired: 4 in, 1 out]
        n849 = local read "浓度2"() -> (w1326:dbl)
        n850 = call-poly <vilib>:"Write Key.vi"("section"=w1295, "error in (no error)"=w1341, "value"=w1326, "key"="浓度2", "refnum"=w1340) -> ("error out"=w1339:errorcluster, "refnum out"=w1338:T6)  [unwired: 4 in, 1 out]
        n851 = local read "浓度3"() -> (w1322:dbl)
        n852 = local read "泵滴定数1"() -> (w1320:dbl)
        n853 = call-poly <vilib>:"Write Key.vi"("section"=w1295, "error in (no error)"=w1339, "value"=w1322, "key"="浓度3", "refnum"=w1338) -> ("error out"=w1337:errorcluster, "refnum out"=w1336:T6)  [unwired: 4 in, 1 out]
        n854 = local read "泵滴定数2"() -> (w1318:dbl)
        n855 = call-poly <vilib>:"Write Key.vi"("section"=w1295, "error in (no error)"=w1337, "value"=w1320, "key"="泵滴定数1", "refnum"=w1336) -> ("error out"=w1335:errorcluster, "refnum out"=w1334:T6)  [unwired: 4 in, 1 out]
        n856 = local read "泵滴定数3"() -> (w1316:dbl)
        n857 = call-poly <vilib>:"Write Key.vi"("section"=w1295, "error in (no error)"=w1335, "value"=w1318, "key"="泵滴定数2", "refnum"=w1334) -> ("error out"=w1333:errorcluster, "refnum out"=w1332:T6)  [unwired: 4 in, 1 out]
        n858 = call-poly <vilib>:"Write Key.vi"("section"=w1295, "error in (no error)"=w1333, "value"=w1316, "key"="泵滴定数3", "refnum"=w1332) -> ("error out"=w1331:errorcluster, "refnum out"=w1330:T6)  [unwired: 4 in, 1 out]
        n859 = local read "浓度4"() -> (w1283:dbl)
        n860 = call-poly <vilib>:"Write Key.vi"("section"=w1295, "error in (no error)"=w1331, "value"=w1283, "key"="浓度4", "refnum"=w1330) -> ("error out"=w1324:errorcluster, "refnum out"=w1325:T6)  [unwired: 4 in, 1 out]
        n861 = local read "浓度5"() -> (w1282:dbl)
        n862 = local read "泵滴定数4"() -> (w1284:dbl)
        n863 = call-poly <vilib>:"Write Key.vi"("section"=w1295, "error in (no error)"=w1324, "value"=w1282, "key"="浓度5", "refnum"=w1325) -> ("error out"=w1292:errorcluster, "refnum out"=w1293:T6)  [unwired: 4 in, 1 out]
        n864 = local read "泵滴定数5"() -> (w1285:dbl)
        n865 = call-poly <vilib>:"Write Key.vi"("section"=w1295, "error in (no error)"=w1292, "value"=w1284, "key"="泵滴定数4", "refnum"=w1293) -> ("error out"=w1329:errorcluster, "refnum out"=w1328:T6)  [unwired: 4 in, 1 out]
        n866 = call-poly <vilib>:"Write Key.vi"("section"=w1295, "error in (no error)"=w1329, "value"=w1285, "key"="泵滴定数5", "refnum"=w1328) -> ("error out"=w1290:errorcluster, "refnum out"=w1291:T6)  [unwired: 4 in, 1 out]
        n867 = local read "启用1"() -> (w1304:bool)
        n868 = call-poly <vilib>:"Write Key.vi"("section"=w1295, "error in (no error)"=w1290, "value"=w1304, "key"="启用1", "refnum"=w1291) -> ("error out"=w1300:errorcluster, "refnum out"=w1303:T6)  [unwired: 4 in, 1 out]
        n869 = local read "启用2"() -> (w1301:bool)
        n870 = call-poly <vilib>:"Write Key.vi"("section"=w1295, "error in (no error)"=w1300, "value"=w1301, "key"="启用2", "refnum"=w1303) -> ("error out"=w1311:errorcluster, "refnum out"=w1310:T6)  [unwired: 4 in, 1 out]
        n871 = local read "启用3"() -> (w1299:bool)
        n872 = call-poly <vilib>:"Write Key.vi"("section"=w1295, "error in (no error)"=w1311, "value"=w1299, "key"="启用3", "refnum"=w1310) -> ("error out"=w1309:errorcluster, "refnum out"=w1308:T6)  [unwired: 4 in, 1 out]
        n873 = local read "启用4"() -> (w1287:bool)
        n874 = call-poly <vilib>:"Write Key.vi"("section"=w1295, "error in (no error)"=w1309, "value"=w1287, "key"="启用4", "refnum"=w1308) -> ("error out"=w1307:errorcluster, "refnum out"=w1306:T6)  [unwired: 4 in, 1 out]
        n875 = local read "启用5"() -> (w1286:bool)
        n876 = call-poly <vilib>:"Write Key.vi"("section"=w1295, "error in (no error)"=w1307, "value"=w1286, "key"="启用5", "refnum"=w1306) -> ("error out"=w1288:errorcluster, "refnum out"=w1289:T6)  [unwired: 4 in, 1 out]
        n877 = call <vilib>:"Close Config Data.vi"("error in (no error)"=w1288, "refnum"=w1289) -> ()  [unwired: 8 in, 2 out]
      }
      event "关闭", "关闭 2", "关闭 3": Value Change {
        n878 = event-data() -> ()  [unwired: 1 in, 6 out]
        n879 = property on="窗格" class="Pane"("Origin"=T5 {"Horizontal"=0, "Vertical"=0} ("原点")) -> ()  [unwired: 2 in, 2 out]
      }
      event Application Instance Close {
        n880 = event-data() -> ()  [unwired: 1 in, 4 out]
      }
      event "时间校准": Value Change {
        n881 = event-data() -> ()  [unwired: 1 in, 6 out]
        n882 = Get Date/Time In Seconds() -> (seconds since 1Jan1904=w1359:timestamp)
        n883 = Build Array(w1359) -> (w1358:timestamp[])
        n884 = call "DateToHex.vi"("DATE"=w1358) -> ("数组"=w1356:u16[])  [unwired: 10 in]
        n885 = Insert Into Array(array=u16[] [1] ("values"), index=1 ("索引"), new element=w1356) -> (w1352:u16[])
        n886 = call "CODMnMB_api.vi"("STEP"=enum16{"open", "read", "write", "close"}."write", "values"=w1352, "starting address"=u16 4612) -> ("error out"=w1351:errorcluster)  [unwired: 6 in, 2 out]
        n887 = call <vilib>:"Clear Errors.vi"("error in (no error)"=w1351) -> ()  [unwired: 5 in, 2 out]
      }
      event "故障清除": Value Change {
        n888 = event-data() -> ()  [unwired: 1 in, 6 out]
        n889 = call "CODMnMB_api.vi"("STEP"=enum16{"open", "read", "write", "close"}."write", "values"=u16[] [1], "starting address"=u16 4611) -> ()  [unwired: 6 in, 3 out]
      }
      event "定时启动": Mouse Down {
        n890 = event-data() -> ()  [unwired: 1 in, 8 out]
        n891 = flat-sequence {
          frame #0 {
            n892 = global read "CODMn断电保存全局变量.vi" "间隔已启动次数"() -> (w1364:dbl)
            n893 = global read "CODMn断电保存全局变量.vi" "间隔设定次数"() -> (w1363:dbl)
            n894 = global read "CODMn断电保存全局变量.vi" "定时控制"() -> (w1366:T9)
            n895 = call "周期设置.vi"("间隔已启动次数"=w1364, "间隔设定启动次数"=w1363, "定时控制输入"=w1366) -> ("定时控制输出"=w1365:T13)  [unwired: 8 in]
            n896 = global write "CODMn断电保存全局变量.vi" "定时控制"(w1365) -> ()
          }
          frame #1 {
            n897 = global read "CODMN外部API.vi" "ping"() -> (w1368:bool)
            n898 = case shown="假" w1368 {
              tunnel: [w1380 w1383] -> w1367
              frame False {
                n899 = global read "COD内部交互全局.vi" "配置文件ini"() -> (w1382:string)
                n900 = call <vilib>:"Application Directory.vi"() -> ("Application Directory"=w1381:path)
                n901 = Build Path(base path=w1381, name or relative path=w1382) -> (appended path=w1380:path)
              }
              frame True {
                n902 = global read "CODMN外部API.vi" "配置文件 path"() -> (w1383:path)
              }
            }
            n903 = call <vilib>:"Open Config Data.vi"("configuration file path"=w1367) -> ("error out"=w1376:errorcluster, "refnum"=w1379:T6)  [unwired: 8 in, 1 out]
            n904 = vi-ref "斯坦道CODMn.lvlib:CODMn断电保存全局变量.vi"() -> (w1378:refnum<vi>)
            n905 = call <userlib>:"Write Panel to INI__ogtk.vi"("error in (no error)"=w1376, "VI ref"=w1378, "refnum"=w1379) -> ("error out"=w1375:errorcluster, "refnum out"=w1377:T6)  [unwired: 7 in]
            n906 = call <vilib>:"Close Config Data.vi"("error in (no error)"=w1375, "refnum"=w1377) -> ("error out"=w1370:errorcluster, "file path"=w1369:path)  [unwired: 8 in]
            n907 = Open/Create/Replace File(file path (use dialog)=w1369, error in=w1370) -> (refnum out=w1373:refnum<file>, error out=w1374:errorcluster)  [unwired: 4 in, 1 out]
            n908 = Flush File(refnum=w1373, error in=w1374) -> (refnum out=w1372:refnum<file>, error out=w1371:errorcluster)
            n909 = Close File(refnum=w1372, error in=w1371) -> ()  [unwired: 2 out]
          }
        }
      }
      event "仪器参数": Value Change {
        n910 = event-data() -> ()  [unwired: 1 in, 6 out]
        n911 = global read "CODMn断电保存全局变量.vi" "CODMn仪器参数"() -> (w1384:T3)
        n912 = call "仪器参数设置.vi"("仪器参数设置"=w1384) -> ("仪器参数设置输出"=w1385:T14)  [unwired: 10 in]
        n913 = Unbundle By Name(w1385) -> ("确定"=w1386:bool)
        n914 = case shown="真" w1386 {
          tunnel: w1385 -> [_ w1388]
          tunnel: w1384 -> [_ w1387]
          frame False {
          }
          frame True {
            n915 = flat-sequence {
              tunnel: w1388 -> [w1405]
              tunnel: w1387 -> [w1404]
              frame #0 {
                n916 = Unbundle By Name(w1405) -> ("测量量程"=w1403:dbl, "测量精度"=w1402:dbl, "测量间隔"=w1401:dbl, "消解温度"=w1400:dbl, "消解时长"=w1399:dbl, "空白校准时间"=w1398:timestamp, "曲线截距"=w1397:dbl, "曲线斜率"=w1396:dbl, "测量检出限"=w1395:dbl, "测量信号值"=w1394:dbl, "线性相关系数"=w1393:dbl, "二次多项式系数"=w1392:dbl, "标样校准时间"=w1391:timestamp, "单位"=w1390:u16)
                n917 = Bundle By Name(cluster=w1404, "测量量程"=w1403, "测量精度"=w1402, "测量间隔"=w1401, "消解温度"=w1400, "消解时长"=w1399, "空白校准时间"=w1398, "曲线截距"=w1397, "曲线斜率"=w1396, "测量检出限"=w1395, "测量信号值"=w1394, "线性相关系数"=w1393, "二次多项式系数"=w1392, "标样校准时间"=w1391, "单位"=w1390) -> (w1389:T3)
                n918 = global write "CODMn断电保存全局变量.vi" "CODMn仪器参数"(w1389) -> ()
              }
              frame #1 {
                n919 = global read "CODMN外部API.vi" "ping"() -> (w1407:bool)
                n920 = case shown="假" w1407 {
                  tunnel: [w1419 w1422] -> w1406
                  frame False {
                    n921 = global read "COD内部交互全局.vi" "配置文件ini"() -> (w1421:string)
                    n922 = call <vilib>:"Application Directory.vi"() -> ("Application Directory"=w1420:path)
                    n923 = Build Path(base path=w1420, name or relative path=w1421) -> (appended path=w1419:path)
                  }
                  frame True {
                    n924 = global read "CODMN外部API.vi" "配置文件 path"() -> (w1422:path)
                  }
                }
                n925 = call <vilib>:"Open Config Data.vi"("configuration file path"=w1406) -> ("error out"=w1415:errorcluster, "refnum"=w1418:T6)  [unwired: 8 in, 1 out]
                n926 = vi-ref "斯坦道CODMn.lvlib:CODMn断电保存全局变量.vi"() -> (w1417:refnum<vi>)
                n927 = call <userlib>:"Write Panel to INI__ogtk.vi"("error in (no error)"=w1415, "VI ref"=w1417, "refnum"=w1418) -> ("error out"=w1414:errorcluster, "refnum out"=w1416:T6)  [unwired: 7 in]
                n928 = call <vilib>:"Close Config Data.vi"("error in (no error)"=w1414, "refnum"=w1416) -> ("error out"=w1409:errorcluster, "file path"=w1408:path)  [unwired: 8 in]
                n929 = Open/Create/Replace File(file path (use dialog)=w1408, error in=w1409) -> (refnum out=w1412:refnum<file>, error out=w1413:errorcluster)  [unwired: 4 in, 1 out]
                n930 = Flush File(refnum=w1412, error in=w1413) -> (refnum out=w1411:refnum<file>, error out=w1410:errorcluster)
                n931 = Close File(refnum=w1411, error in=w1410) -> ()  [unwired: 2 out]
              }
            }
          }
        }
      }
      event "远程自动校准浓度", "远程校准量程": Value Change {
        n932 = event-data() -> ()  [unwired: 1 in, 6 out]
        n933 = flat-sequence {
          frame #0 {
            n934 = global write "CODMn断电保存全局变量.vi" "远程校准量程"("远程校准量程") -> ()
            n935 = global write "CODMn断电保存全局变量.vi" "远程自动校准浓度"("远程自动校准浓度") -> ()
          }
          frame #1 {
            n936 = global read "CODMN外部API.vi" "ping"() -> (w1426:bool)
            n937 = case shown="假" w1426 {
              tunnel: [w1438 w1441] -> w1425
              frame False {
                n938 = global read "COD内部交互全局.vi" "配置文件ini"() -> (w1440:string)
                n939 = call <vilib>:"Application Directory.vi"() -> ("Application Directory"=w1439:path)
                n940 = Build Path(base path=w1439, name or relative path=w1440) -> (appended path=w1438:path)
              }
              frame True {
                n941 = global read "CODMN外部API.vi" "配置文件 path"() -> (w1441:path)
              }
            }
            n942 = call <vilib>:"Open Config Data.vi"("configuration file path"=w1425) -> ("error out"=w1434:errorcluster, "refnum"=w1437:T6)  [unwired: 8 in, 1 out]
            n943 = vi-ref "斯坦道CODMn.lvlib:CODMn断电保存全局变量.vi"() -> (w1436:refnum<vi>)
            n944 = call <userlib>:"Write Panel to INI__ogtk.vi"("error in (no error)"=w1434, "VI ref"=w1436, "refnum"=w1437) -> ("error out"=w1433:errorcluster, "refnum out"=w1435:T6)  [unwired: 7 in]
            n945 = call <vilib>:"Close Config Data.vi"("error in (no error)"=w1433, "refnum"=w1435) -> ("error out"=w1428:errorcluster, "file path"=w1427:path)  [unwired: 8 in]
            n946 = Open/Create/Replace File(file path (use dialog)=w1427, error in=w1428) -> (refnum out=w1431:refnum<file>, error out=w1432:errorcluster)  [unwired: 4 in, 1 out]
            n947 = Flush File(refnum=w1431, error in=w1432) -> (refnum out=w1430:refnum<file>, error out=w1429:errorcluster)
            n948 = Close File(refnum=w1430, error in=w1429) -> ()  [unwired: 2 out]
          }
        }
      }
      event "测量模式(公式)": Value Change {
        n949 = event-data() -> ()  [unwired: 1 in, 6 out]
        n950 = flat-sequence {
          frame #0 {
            n951 = global write "CODMn断电保存全局变量.vi" "测量模式(公式)"("测量模式(公式)") -> ()
          }
          frame #1 {
            n952 = global read "CODMN外部API.vi" "ping"() -> (w1444:bool)
            n953 = case shown="假" w1444 {
              tunnel: [w1456 w1459] -> w1443
              frame False {
                n954 = global read "COD内部交互全局.vi" "配置文件ini"() -> (w1458:string)
                n955 = call <vilib>:"Application Directory.vi"() -> ("Application Directory"=w1457:path)
                n956 = Build Path(base path=w1457, name or relative path=w1458) -> (appended path=w1456:path)
              }
              frame True {
                n957 = global read "CODMN外部API.vi" "配置文件 path"() -> (w1459:path)
              }
            }
            n958 = call <vilib>:"Open Config Data.vi"("configuration file path"=w1443) -> ("error out"=w1452:errorcluster, "refnum"=w1455:T6)  [unwired: 8 in, 1 out]
            n959 = vi-ref "斯坦道CODMn.lvlib:CODMn断电保存全局变量.vi"() -> (w1454:refnum<vi>)
            n960 = call <userlib>:"Write Panel to INI__ogtk.vi"("error in (no error)"=w1452, "VI ref"=w1454, "refnum"=w1455) -> ("error out"=w1451:errorcluster, "refnum out"=w1453:T6)  [unwired: 7 in]
            n961 = call <vilib>:"Close Config Data.vi"("error in (no error)"=w1451, "refnum"=w1453) -> ("error out"=w1446:errorcluster, "file path"=w1445:path)  [unwired: 8 in]
            n962 = Open/Create/Replace File(file path (use dialog)=w1445, error in=w1446) -> (refnum out=w1449:refnum<file>, error out=w1450:errorcluster)  [unwired: 4 in, 1 out]
            n963 = Flush File(refnum=w1449, error in=w1450) -> (refnum out=w1448:refnum<file>, error out=w1447:errorcluster)
            n964 = Close File(refnum=w1448, error in=w1447) -> ()  [unwired: 2 out]
          }
        }
      }
      event "跨度量程选择", "跨度液浓度", "零点核查量程选择", "零点核查浓度", "标样浓度", "标样核查量程选择": Value Change {
        n965 = event-data() -> ()  [unwired: 1 in, 6 out]
        n966 = flat-sequence {
          frame #0 {
            n967 = global write "CODMn断电保存全局变量.vi" "标样浓度"("标样浓度") -> ()
            n968 = global write "CODMn断电保存全局变量.vi" "零点核查浓度"("零点核查浓度") -> ()
            n969 = global write "CODMn断电保存全局变量.vi" "跨度液浓度"("跨度液浓度") -> ()
            n970 = global write "CODMn断电保存全局变量.vi" "CODMn跨度量程选择"("跨度量程选择") -> ()
            n971 = global write "CODMn断电保存全局变量.vi" "标样核查量程选择"("标样核查量程选择") -> ()
            n972 = global write "CODMn断电保存全局变量.vi" "零点核查量程选择"("零点核查量程选择") -> ()
          }
          frame #1 {
            n973 = global read "CODMN外部API.vi" "ping"() -> (w1467:bool)
            n974 = case shown="假" w1467 {
              tunnel: [w1479 w1482] -> w1466
              frame False {
                n975 = global read "COD内部交互全局.vi" "配置文件ini"() -> (w1481:string)
                n976 = call <vilib>:"Application Directory.vi"() -> ("Application Directory"=w1480:path)
                n977 = Build Path(base path=w1480, name or relative path=w1481) -> (appended path=w1479:path)
              }
              frame True {
                n978 = global read "CODMN外部API.vi" "配置文件 path"() -> (w1482:path)
              }
            }
            n979 = call <vilib>:"Open Config Data.vi"("configuration file path"=w1466) -> ("error out"=w1475:errorcluster, "refnum"=w1478:T6)  [unwired: 8 in, 1 out]
            n980 = vi-ref "斯坦道CODMn.lvlib:CODMn断电保存全局变量.vi"() -> (w1477:refnum<vi>)
            n981 = call <userlib>:"Write Panel to INI__ogtk.vi"("error in (no error)"=w1475, "VI ref"=w1477, "refnum"=w1478) -> ("error out"=w1474:errorcluster, "refnum out"=w1476:T6)  [unwired: 7 in]
            n982 = call <vilib>:"Close Config Data.vi"("error in (no error)"=w1474, "refnum"=w1476) -> ("error out"=w1469:errorcluster, "file path"=w1468:path)  [unwired: 8 in]
            n983 = Open/Create/Replace File(file path (use dialog)=w1468, error in=w1469) -> (refnum out=w1472:refnum<file>, error out=w1473:errorcluster)  [unwired: 4 in, 1 out]
            n984 = Flush File(refnum=w1472, error in=w1473) -> (refnum out=w1471:refnum<file>, error out=w1470:errorcluster)
            n985 = Close File(refnum=w1471, error in=w1470) -> ()  [unwired: 2 out]
          }
        }
      }
      event "校准1", "校准2", "校准3", "校准4", "校准5": Value Change {
        n986 = event-data() -> ()  [unwired: 1 in, 6 out]
        n987 = flat-sequence {
          tunnel: w1486 -> [w1495]
          tunnel: [w1495] -> w1488
          tunnel: w1483 -> [w1494]
          tunnel: [w1494] -> w1485
          tunnel: w1488 -> [w1531]
          tunnel: [w1531] -> w1487
          tunnel: w1485 -> [w1530]
          tunnel: [w1530] -> w1484
          tunnel: w1487 -> [w1553]
          tunnel: w1484 -> [w1552]
          frame #0 {
            n988 = Build Array("校准1", "校准2", "校准3", "校准4", "校准5") -> (w1498:bool[])
            n989 = for {
              tunnel: w1498 -> [w1513] mode=indexing
              tunnel: [w1505] -> w1489
              i -> [w1506]
              n990 = case shown="4" w1506 {
                tunnel: ["浓度1" "浓度2" "浓度3" "浓度4" "浓度5"] -> w1509
                frame 0, Default {
                }
                frame 1 {
                }
                frame 2 {
                }
                frame 3 {
                }
                frame 4 {
                }
              }
              n991 = Multiply(x=w1509, y=100.0) -> (x*y=w1507:dbl)
              n992 = Insert Into Array(array=u16[] [] ("values"), index=0 ("索引"), new element=w1507) -> (w1510:u16[])
              n993 = case shown="真" w1513 {
                tunnel: w1510 -> [_ w1522]
                tunnel: w1506 -> [_ w1524]
                tunnel: [_ w1519] -> w1505
                frame False {
                }
                frame True {
                  n994 = Increment(x=w1524) -> (x+1=w1520:i32)
                  n995 = global write "COD内部交互全局.vi" "当前校准"(w1520) -> ()
                  n996 = call "CODMnMB_api.vi"("STEP"=enum16{"open", "read", "write", "close"}."write", "values"=w1522, "starting address"=u16 4274) -> ("error out"=w1519:errorcluster)  [unwired: 6 in, 2 out]
                }
              }
            }
            n997 = local read "量程选择"() -> (w1491:enum16{"低量程", "高量程", "0-2量程"})
            n998 = case shown="\"高量程\"" w1491 {
              tunnel: [u16[] [0] ("values") u16[] [1] ("values") u16[] [0] ("values")] -> w1490
              frame "低量程", Default {
              }
              frame "高量程" {
              }
              frame "0-2量程" {
              }
            }
            n999 = call "CODMnMB_api.vi"("STEP"=enum16{"open", "read", "write", "close"}."write", "Error in"=w1489, "values"=w1490, "starting address"=u16 4276) -> ()  [unwired: 5 in, 3 out]
          }
          frame #1 {
            n1000 = global read "COD内部交互全局.vi" "当前校准"() -> (w1532:i32)
            n1001 = case shown="5" w1532 {
              tunnel: [w1541 w1542 w1543 w1544 w1545] -> w1528
              frame 1, Default {
                n1002 = local read "浓度1"() -> (w1541:dbl)
              }
              frame 2 {
                n1003 = local read "浓度2"() -> (w1542:dbl)
              }
              frame 3 {
                n1004 = local read "浓度3"() -> (w1543:dbl)
              }
              frame 4 {
                n1005 = local read "浓度4"() -> (w1544:dbl)
              }
              frame 5 {
                n1006 = local read "浓度5"() -> (w1545:dbl)
              }
            }
            n1007 = Number To Decimal String(number=w1528) -> (decimal integer string=w1527:string)  [unwired: 1 in]
            n1008 = Concatenate Strings("仪器校准中!\n当前校准浓度为:", w1527, "mg/L" ("字符串")) -> (w1525:string)
            n1009 = Not Equal To 0?(x=w1528) -> (x != 0?=w1536:bool)
            n1010 = global write "COD内部交互全局.vi" "校准内容显示"(w1525) -> ()
            n1011 = case shown="真" w1536 {
              tunnel: [u16 8 ("address") u16 9 ("address")] -> w1540
              tunnel: ["校零" ("测量模式") "校标" ("测量模式")] -> w1537
              frame False {
              }
              frame True {
              }
            }
            n1012 = global write "COD测量模式全局.vi" "测量模式"(w1537) -> ()
            n1013 = Insert Into Array(array=u16[] [] ("values"), index=0 ("索引"), new element=w1540) -> (w1533:u16[])
            n1014 = call "CODMnMB_api.vi"("STEP"=enum16{"open", "read", "write", "close"}."write", "values"=w1533, "starting address"=u16 4608 ("address")) -> ()  [unwired: 6 in, 3 out]
          }
          frame #2 {
            n1015 = local read "选用水样"() -> (w1561:enum16{"葡萄糖", "草酸钠"})
            n1016 = global read "CODMN外部API.vi" "ping"() -> (w1551:bool)
            n1017 = case shown="假" w1551 {
              tunnel: [w1569 w1572] -> w1550
              frame False {
                n1018 = global read "COD内部交互全局.vi" "配置文件ini"() -> (w1571:string)
                n1019 = call <vilib>:"Application Directory.vi"() -> ("Application Directory"=w1570:path)
                n1020 = Build Path(base path=w1570, name or relative path=w1571) -> (appended path=w1569:path)
              }
              frame True {
                n1021 = global read "CODMN外部API.vi" "配置文件 path"() -> (w1572:path)
              }
            }
            n1022 = local read "量程选择"() -> (w1560:enum16{"低量程", "高量程", "0-2量程"})
            n1023 = case shown="\"葡萄糖\", 默认" w1561 {
              tunnel: ["葡萄糖标线" ("section") "草酸钠标线" ("section")] -> w1562
              frame "葡萄糖", Default {
              }
              frame "草酸钠" {
              }
            }
            n1024 = Bundle By Name(cluster=cluster{"命令":string} {"命令"=""} ("元素"), "命令"="CODMn读取参数" ("名称（未命名）")) -> (w1557:cluster{"命令":string})
            n1025 = case shown="\"0-2量程\"" w1560 {
              tunnel: ["低量程" "高量程" "0-2量程"] -> w1563
              frame "低量程", Default {
              }
              frame "高量程" {
              }
              frame "0-2量程" {
              }
            }
            n1026 = global read "COD内部交互全局.vi" "当前校准"() -> (w1558:i32)
            n1027 = Enqueue Element(queue=w1553, element=w1557, timeout in ms (-1)=1000 ("超时毫秒(-1)"), error in (no error)=w1552) -> ()  [unwired: 3 out]
            n1028 = Concatenate Strings(w1562, w1563) -> (w1559:string)
            n1029 = call <vilib>:"Open Config Data.vi"("configuration file path"=w1550) -> ("error out"=w1567:errorcluster, "refnum"=w1568:T6)  [unwired: 8 in, 1 out]
            n1030 = call-poly <vilib>:"Write Key.vi"("section"=w1559, "error in (no error)"=w1567, "value"=w1558, "key"="当前选用的校准" ("section"), "refnum"=w1568) -> ("error out"=w1564:errorcluster, "refnum out"=w1565:T6)  [unwired: 4 in, 1 out]
            n1031 = call <vilib>:"Close Config Data.vi"("error in (no error)"=w1564, "refnum"=w1565) -> ()  [unwired: 8 in, 2 out]
          }
        }
      }
      event "水样量程选择:", "低切高阈值:", "高切低阈值:": Value Change {
        n1032 = event-data() -> ()  [unwired: 1 in, 6 out]
        n1033 = flat-sequence {
          frame #0 {
            n1034 = global write "CODMn断电保存全局变量.vi" "高切低阈值:"("高切低阈值:") -> ()
            n1035 = global write "CODMn断电保存全局变量.vi" "自动切换量程:"("水样量程选择:") -> ()
            n1036 = global write "CODMn断电保存全局变量.vi" "低切高阈值:"("低切高阈值:") -> ()
          }
          frame #1 {
            n1037 = global read "CODMN外部API.vi" "ping"() -> (w1582:bool)
            n1038 = case shown="假" w1582 {
              tunnel: [w1594 w1597] -> w1581
              frame False {
                n1039 = global read "COD内部交互全局.vi" "配置文件ini"() -> (w1596:string)
                n1040 = call <vilib>:"Application Directory.vi"() -> ("Application Directory"=w1595:path)
                n1041 = Build Path(base path=w1595, name or relative path=w1596) -> (appended path=w1594:path)
              }
              frame True {
                n1042 = global read "CODMN外部API.vi" "配置文件 path"() -> (w1597:path)
              }
            }
            n1043 = call <vilib>:"Open Config Data.vi"("configuration file path"=w1581) -> ("error out"=w1590:errorcluster, "refnum"=w1593:T6)  [unwired: 8 in, 1 out]
            n1044 = vi-ref "斯坦道CODMn.lvlib:CODMn断电保存全局变量.vi"() -> (w1592:refnum<vi>)
            n1045 = call <userlib>:"Write Panel to INI__ogtk.vi"("error in (no error)"=w1590, "VI ref"=w1592, "refnum"=w1593) -> ("error out"=w1589:errorcluster, "refnum out"=w1591:T6)  [unwired: 7 in]
            n1046 = call <vilib>:"Close Config Data.vi"("error in (no error)"=w1589, "refnum"=w1591) -> ("error out"=w1584:errorcluster, "file path"=w1583:path)  [unwired: 8 in]
            n1047 = Open/Create/Replace File(file path (use dialog)=w1583, error in=w1584) -> (refnum out=w1587:refnum<file>, error out=w1588:errorcluster)  [unwired: 4 in, 1 out]
            n1048 = Flush File(refnum=w1587, error in=w1588) -> (refnum out=w1586:refnum<file>, error out=w1585:errorcluster)
            n1049 = Close File(refnum=w1586, error in=w1585) -> ()  [unwired: 2 out]
          }
        }
      }
      event "模型": Value Change {
        n1050 = event-data() -> ()  [unwired: 1 in, 6 out]
        n1051 = global read "CODMN外部API.vi" "ping"() -> (w1599:bool)
        n1052 = case shown="假" w1599 {
          tunnel: [w1607 w1610] -> w1598
          frame False {
            n1053 = global read "COD内部交互全局.vi" "配置文件ini"() -> (w1609:string)
            n1054 = call <vilib>:"Application Directory.vi"() -> ("Application Directory"=w1608:path)
            n1055 = Build Path(base path=w1608, name or relative path=w1609) -> (appended path=w1607:path)
          }
          frame True {
            n1056 = global read "CODMN外部API.vi" "配置文件 path"() -> (w1610:path)
          }
        }
        n1057 = call <vilib>:"Open Config Data.vi"("configuration file path"=w1598) -> ("error out"=w1605:errorcluster, "refnum"=w1606:T6)  [unwired: 8 in, 1 out]
        n1058 = local read "模型"() -> (w1600:enum32{"线性", "多项式"})
        n1059 = call-poly <vilib>:"Write Key.vi"("section"="CODMn模型选择" ("key"), "error in (no error)"=w1605, "value"=w1600, "key"="线性和多项式", "refnum"=w1606) -> ("error out"=w1601:errorcluster, "refnum out"=w1602:T6)  [unwired: 4 in, 1 out]
        n1060 = call <vilib>:"Close Config Data.vi"("error in (no error)"=w1601, "refnum"=w1602) -> ()  [unwired: 8 in, 2 out]
      }
      event "浓度1", "浓度2", "浓度3", "泵滴定数1", "泵滴定数2", "泵滴定数3", "启用1", "启用2", "启用3", "浓度4", "浓度5", "泵滴定数4", "泵滴定数5", "启用4", "启用5": Value Change {
        n1061 = event-data() -> ()  [unwired: 1 in, 6 out]
        n1062 = local read "选用水样"() -> (w1628:enum16{"葡萄糖", "草酸钠"})
        n1063 = local read "量程选择"() -> (w1627:enum16{"低量程", "高量程", "0-2量程"})
        n1064 = case shown="\"葡萄糖\", 默认" w1628 {
          tunnel: ["葡萄糖标线" ("section") "草酸钠标线" ("section")] -> w1634
          frame "葡萄糖", Default {
          }
          frame "草酸钠" {
          }
        }
        n1065 = case shown="\"0-2量程\"" w1627 {
          tunnel: ["低量程" "高量程" "0-2量程"] -> w1625
          frame "低量程", Default {
          }
          frame "高量程" {
          }
          frame "0-2量程" {
          }
        }
        n1066 = global read "CODMN外部API.vi" "ping"() -> (w1612:bool)
        n1067 = case shown="假" w1612 {
          tunnel: [w1685 w1688] -> w1611
          frame False {
            n1068 = global read "COD内部交互全局.vi" "配置文件ini"() -> (w1687:string)
            n1069 = call <vilib>:"Application Directory.vi"() -> ("Application Directory"=w1686:path)
            n1070 = Build Path(base path=w1686, name or relative path=w1687) -> (appended path=w1685:path)
          }
          frame True {
            n1071 = global read "CODMN外部API.vi" "配置文件 path"() -> (w1688:path)
          }
        }
        n1072 = Concatenate Strings(w1634, w1625) -> (w1626:string)
        n1073 = call <vilib>:"Open Config Data.vi"("configuration file path"=w1611) -> ("error out"=w1683:errorcluster, "refnum"=w1684:T6)  [unwired: 8 in, 1 out]
        n1074 = local read "浓度1"() -> (w1681:dbl)
        n1075 = call-poly <vilib>:"Write Key.vi"("section"=w1626, "error in (no error)"=w1683, "value"=w1681, "key"="浓度1", "refnum"=w1684) -> ("error out"=w1680:errorcluster, "refnum out"=w1679:T6)  [unwired: 4 in, 1 out]
        n1076 = local read "浓度2"() -> (w1665:dbl)
        n1077 = call-poly <vilib>:"Write Key.vi"("section"=w1626, "error in (no error)"=w1680, "value"=w1665, "key"="浓度2", "refnum"=w1679) -> ("error out"=w1678:errorcluster, "refnum out"=w1677:T6)  [unwired: 4 in, 1 out]
        n1078 = local read "浓度3"() -> (w1661:dbl)
        n1079 = local read "泵滴定数1"() -> (w1659:dbl)
        n1080 = call-poly <vilib>:"Write Key.vi"("section"=w1626, "error in (no error)"=w1678, "value"=w1661, "key"="浓度3", "refnum"=w1677) -> ("error out"=w1676:errorcluster, "refnum out"=w1675:T6)  [unwired: 4 in, 1 out]
        n1081 = local read "泵滴定数2"() -> (w1657:dbl)
        n1082 = call-poly <vilib>:"Write Key.vi"("section"=w1626, "error in (no error)"=w1676, "value"=w1659, "key"="泵滴定数1", "refnum"=w1675) -> ("error out"=w1674:errorcluster, "refnum out"=w1673:T6)  [unwired: 4 in, 1 out]
        n1083 = local read "泵滴定数3"() -> (w1655:dbl)
        n1084 = call-poly <vilib>:"Write Key.vi"("section"=w1626, "error in (no error)"=w1674, "value"=w1657, "key"="泵滴定数2", "refnum"=w1673) -> ("error out"=w1672:errorcluster, "refnum out"=w1671:T6)  [unwired: 4 in, 1 out]
        n1085 = call-poly <vilib>:"Write Key.vi"("section"=w1626, "error in (no error)"=w1672, "value"=w1655, "key"="泵滴定数3", "refnum"=w1671) -> ("error out"=w1670:errorcluster, "refnum out"=w1669:T6)  [unwired: 4 in, 1 out]
        n1086 = local read "浓度4"() -> (w1624:dbl)
        n1087 = call-poly <vilib>:"Write Key.vi"("section"=w1626, "error in (no error)"=w1670, "value"=w1624, "key"="浓度4", "refnum"=w1669) -> ("error out"=w1663:errorcluster, "refnum out"=w1664:T6)  [unwired: 4 in, 1 out]
        n1088 = local read "浓度5"() -> (w1623:dbl)
        n1089 = local read "泵滴定数4"() -> (w1620:dbl)
        n1090 = call-poly <vilib>:"Write Key.vi"("section"=w1626, "error in (no error)"=w1663, "value"=w1623, "key"="浓度5", "refnum"=w1664) -> ("error out"=w1621:errorcluster, "refnum out"=w1622:T6)  [unwired: 4 in, 1 out]
        n1091 = local read "泵滴定数5"() -> (w1619:dbl)
        n1092 = call-poly <vilib>:"Write Key.vi"("section"=w1626, "error in (no error)"=w1621, "value"=w1620, "key"="泵滴定数4", "refnum"=w1622) -> ("error out"=w1668:errorcluster, "refnum out"=w1667:T6)  [unwired: 4 in, 1 out]
        n1093 = call-poly <vilib>:"Write Key.vi"("section"=w1626, "error in (no error)"=w1668, "value"=w1619, "key"="泵滴定数5", "refnum"=w1667) -> ("error out"=w1617:errorcluster, "refnum out"=w1618:T6)  [unwired: 4 in, 1 out]
        n1094 = local read "启用1"() -> (w1643:bool)
        n1095 = call-poly <vilib>:"Write Key.vi"("section"=w1626, "error in (no error)"=w1617, "value"=w1643, "key"="启用1", "refnum"=w1618) -> ("error out"=w1639:errorcluster, "refnum out"=w1642:T6)  [unwired: 4 in, 1 out]
        n1096 = local read "启用2"() -> (w1640:bool)
        n1097 = call-poly <vilib>:"Write Key.vi"("section"=w1626, "error in (no error)"=w1639, "value"=w1640, "key"="启用2", "refnum"=w1642) -> ("error out"=w1650:errorcluster, "refnum out"=w1649:T6)  [unwired: 4 in, 1 out]
        n1098 = local read "启用3"() -> (w1638:bool)
        n1099 = call-poly <vilib>:"Write Key.vi"("section"=w1626, "error in (no error)"=w1650, "value"=w1638, "key"="启用3", "refnum"=w1649) -> ("error out"=w1648:errorcluster, "refnum out"=w1647:T6)  [unwired: 4 in, 1 out]
        n1100 = local read "启用4"() -> (w1613:bool)
        n1101 = call-poly <vilib>:"Write Key.vi"("section"=w1626, "error in (no error)"=w1648, "value"=w1613, "key"="启用4", "refnum"=w1647) -> ("error out"=w1646:errorcluster, "refnum out"=w1645:T6)  [unwired: 4 in, 1 out]
        n1102 = local read "启用5"() -> (w1614:bool)
        n1103 = local read "选用水样"() -> (w1633:enum16{"葡萄糖", "草酸钠"})
        n1104 = call-poly <vilib>:"Write Key.vi"("section"=w1626, "error in (no error)"=w1646, "value"=w1614, "key"="启用5", "refnum"=w1645) -> ("error out"=w1615:errorcluster, "refnum out"=w1616:T6)  [unwired: 4 in, 1 out]
        n1105 = call-poly <vilib>:"Write Key.vi"("section"="标线选择", "error in (no error)"=w1615, "value"=w1633, "key"="选用水样", "refnum"=w1616) -> ("error out"=w1630:errorcluster, "refnum out"=w1631:T6)  [unwired: 4 in, 1 out]
        n1106 = call <vilib>:"Close Config Data.vi"("error in (no error)"=w1630, "refnum"=w1631) -> ()  [unwired: 8 in, 2 out]
      }
      event "读取": Value Change {
        (unwired) u16 94 ("number of holding registers")
        (unwired) u16 4616 ("starting address")
        n1107 = event-data() -> ()  [unwired: 1 in, 6 out]
        n1108 = Bundle By Name(cluster=cluster{"命令":string} {"命令"=""} ("元素"), "命令"="CODMn读取公式" ("名称（未命名）")) -> (w1694:cluster{"命令":string})
        n1109 = Enqueue Element(queue=w1698, element=w1694, error in (no error)=w1697) -> ()  [unwired: 1 in, 3 out]
      }
      event "写入": Mouse Down {
        n1110 = event-data() -> ()  [unwired: 1 in, 8 out]
        n1111 = Two Button Dialog(message="是否将上方方程系数K、B、X^2的值写入，写入会覆盖原有公式！" ("消息")) -> (T button?=w1699:bool)  [unwired: 2 in]
        n1112 = case shown="真" w1699 {
          frame False {
          }
          frame True {
            n1113 = local read "模型"() -> (w1710:enum32{"线性", "多项式"})
            n1114 = case shown="\"多项式\"" w1710 {
              tunnel: [w1739 w1783] -> w1708
              tunnel: [w1738 w1782] -> w1707
              frame "线性", Default {
                (unwired) "线性" ("table输入")
                n1115 = local read "测量模式(公式)"() -> (w1740:u16)
                n1116 = case shown="1" w1740 {
                  tunnel: [u16 4626 ("starting address") w1747 w1752 w1757 w1762 w1767 w1772 w1777] -> w1739
                  frame 0, Default {
                  }
                  frame 1 {
                    n1117 = local read "量程选择"() -> (w1746:enum16{"低量程", "高量程", "0-2量程"})
                    n1118 = case shown="\"低量程\", 默认" w1746 {
                      tunnel: [u16 4626 ("starting address") u16 4632 ("starting address") u16 4638 ("starting address")] -> w1747
                      frame "低量程", Default {
                      }
                      frame "高量程" {
                      }
                      frame "0-2量程" {
                      }
                    }
                  }
                  frame 2 {
                    n1119 = local read "量程选择"() -> (w1751:enum16{"低量程", "高量程", "0-2量程"})
                    n1120 = case shown="\"低量程\", 默认" w1751 {
                      tunnel: [u16 4638 ("starting address") u16 4644 ("starting address") u16 4638 ("starting address")] -> w1752
                      frame "低量程", Default {
                      }
                      frame "高量程" {
                      }
                      frame "0-2量程" {
                      }
                    }
                  }
                  frame 3 {
                    n1121 = local read "量程选择"() -> (w1756:enum16{"低量程", "高量程", "0-2量程"})
                    n1122 = case shown="\"低量程\", 默认" w1756 {
                      tunnel: [u16 4650 ("starting address") u16 4656 ("starting address") u16 4638 ("starting address")] -> w1757
                      frame "低量程", Default {
                      }
                      frame "高量程" {
                      }
                      frame "0-2量程" {
                      }
                    }
                  }
                  frame 4 {
                    n1123 = local read "量程选择"() -> (w1761:enum16{"低量程", "高量程", "0-2量程"})
                    n1124 = case shown="\"低量程\", 默认" w1761 {
                      tunnel: [u16 4662 ("starting address") u16 4668 ("starting address") u16 4638 ("starting address")] -> w1762
                      frame "低量程", Default {
                      }
                      frame "高量程" {
                      }
                      frame "0-2量程" {
                      }
                    }
                  }
                  frame 5 {
                    n1125 = local read "量程选择"() -> (w1766:enum16{"低量程", "高量程", "0-2量程"})
                    n1126 = case shown="\"低量程\", 默认" w1766 {
                      tunnel: [u16 4674 ("starting address") u16 4680 ("starting address") u16 4638 ("starting address")] -> w1767
                      frame "低量程", Default {
                      }
                      frame "高量程" {
                      }
                      frame "0-2量程" {
                      }
                    }
                  }
                  frame 6 {
                    n1127 = local read "量程选择"() -> (w1771:enum16{"低量程", "高量程", "0-2量程"})
                    n1128 = case shown="\"低量程\", 默认" w1771 {
                      tunnel: [u16 4686 ("starting address") u16 4692 ("starting address") u16 4638 ("starting address")] -> w1772
                      frame "低量程", Default {
                      }
                      frame "高量程" {
                      }
                      frame "0-2量程" {
                      }
                    }
                  }
                  frame 7 {
                    n1129 = local read "量程选择"() -> (w1776:enum16{"低量程", "高量程", "0-2量程"})
                    n1130 = case shown="\"低量程\", 默认" w1776 {
                      tunnel: [u16 4698 ("starting address") u16 4704 ("starting address") u16 4638 ("starting address")] -> w1777
                      frame "低量程", Default {
                      }
                      frame "高量程" {
                      }
                      frame "0-2量程" {
                      }
                    }
                  }
                }
                n1131 = local read "K"() -> (w1744:dbl)
                n1132 = local read "b"() -> (w1743:dbl)
                n1133 = Build Array(w1744, w1743, 0.0 ("元素")) -> (w1742:dbl[])
                n1134 = call "浮点转CDAB整形cod.vi"("浮点数"=w1742) -> ("CDAB整形输出"=w1738:u16[])  [unwired: 10 in]
              }
              frame "多项式" {
                (unwired) "多项式" ("table输入")
                # "b,k,c"
                n1135 = local read "多项式系数"() -> (w1788:dbl[])
                n1136 = local read "测量模式(公式)"() -> (w1784:u16)
                n1137 = Index Array(array=w1788) -> (element #1=w1786:dbl, element #2=w1781:dbl, element #3=w1785:dbl)  [unwired: 3 in]
                n1138 = case shown="1" w1784 {
                  tunnel: [u16 4626 ("starting address") w1791 w1796 w1801 w1806 w1811 w1816 w1821] -> w1783
                  frame 0, Default {
                  }
                  frame 1 {
                    n1139 = local read "量程选择"() -> (w1790:enum16{"低量程", "高量程", "0-2量程"})
                    n1140 = case shown="\"低量程\", 默认" w1790 {
                      tunnel: [u16 4626 ("starting address") u16 4632 ("starting address") u16 4638 ("starting address")] -> w1791
                      frame "低量程", Default {
                      }
                      frame "高量程" {
                      }
                      frame "0-2量程" {
                      }
                    }
                  }
                  frame 2 {
                    n1141 = local read "量程选择"() -> (w1795:enum16{"低量程", "高量程", "0-2量程"})
                    n1142 = case shown="\"低量程\", 默认" w1795 {
                      tunnel: [u16 4638 ("starting address") u16 4644 ("starting address") u16 4638 ("starting address")] -> w1796
                      frame "低量程", Default {
                      }
                      frame "高量程" {
                      }
                      frame "0-2量程" {
                      }
                    }
                  }
                  frame 3 {
                    n1143 = local read "量程选择"() -> (w1800:enum16{"低量程", "高量程", "0-2量程"})
                    n1144 = case shown="\"低量程\", 默认" w1800 {
                      tunnel: [u16 4650 ("starting address") u16 4656 ("starting address") u16 4638 ("starting address")] -> w1801
                      frame "低量程", Default {
                      }
                      frame "高量程" {
                      }
                      frame "0-2量程" {
                      }
                    }
                  }
                  frame 4 {
                    n1145 = local read "量程选择"() -> (w1805:enum16{"低量程", "高量程", "0-2量程"})
                    n1146 = case shown="\"低量程\", 默认" w1805 {
                      tunnel: [u16 4662 ("starting address") u16 4668 ("starting address") u16 4638 ("starting address")] -> w1806
                      frame "低量程", Default {
                      }
                      frame "高量程" {
                      }
                      frame "0-2量程" {
                      }
                    }
                  }
                  frame 5 {
                    n1147 = local read "量程选择"() -> (w1810:enum16{"低量程", "高量程", "0-2量程"})
                    n1148 = case shown="\"低量程\", 默认" w1810 {
                      tunnel: [u16 4674 ("starting address") u16 4680 ("starting address") u16 4638 ("starting address")] -> w1811
                      frame "低量程", Default {
                      }
                      frame "高量程" {
                      }
                      frame "0-2量程" {
                      }
                    }
                  }
                  frame 6 {
                    n1149 = local read "量程选择"() -> (w1815:enum16{"低量程", "高量程", "0-2量程"})
                    n1150 = case shown="\"低量程\", 默认" w1815 {
                      tunnel: [u16 4686 ("starting address") u16 4692 ("starting address") u16 4638 ("starting address")] -> w1816
                      frame "低量程", Default {
                      }
                      frame "高量程" {
                      }
                      frame "0-2量程" {
                      }
                    }
                  }
                  frame 7 {
                    n1151 = local read "量程选择"() -> (w1820:enum16{"低量程", "高量程", "0-2量程"})
                    n1152 = case shown="\"低量程\", 默认" w1820 {
                      tunnel: [u16 4698 ("starting address") u16 4704 ("starting address") u16 4638 ("starting address")] -> w1821
                      frame "低量程", Default {
                      }
                      frame "高量程" {
                      }
                      frame "0-2量程" {
                      }
                    }
                  }
                }
                n1153 = Build Array(w1781, w1786, w1785) -> (w1787:dbl[])
                n1154 = call "浮点转CDAB整形cod.vi"("浮点数"=w1787) -> ("CDAB整形输出"=w1782:u16[])  [unwired: 10 in]
              }
            }
            n1155 = local read "多项式系数"() -> (w1704:dbl[])
            n1156 = call "CODMnMB_api.vi"("STEP"=enum16{"open", "read", "write", "close"}."write", "values"=w1707, "starting address"=w1708) -> ("error out"=w1706:errorcluster)  [unwired: 6 in, 2 out]
            n1157 = Index Array(array=w1704) -> (element #1=w1703:dbl, element #2=w1702:dbl, element #3=w1701:dbl)  [unwired: 3 in]
            n1158 = case shown="无错误" w1706 {
              tunnel: ["写入成功！" "写入失败！"] -> w1705
              tunnel: w1703 -> [w1716 _]
              tunnel: w1702 -> [w1715 _]
              tunnel: w1701 -> [w1714 _]
              frame No Error {
                n1159 = Number To Fractional String(number=w1716) -> (F-format string=w1712:string)  [unwired: 3 in]
                n1160 = Number To Fractional String(number=w1715) -> (F-format string=w1713:string)  [unwired: 3 in]
                n1161 = Number To Fractional String(number=w1714) -> (F-format string=w1711:string)  [unwired: 3 in]
                n1162 = property on="模型" class="Enum (严格)"() -> ("RingText.Text"=w1726:string)  [unwired: 2 in, 2 out]
                n1163 = property on="测量模式(公式)" class="Ring (严格)"() -> ("RingText.Text"=w1725:string)  [unwired: 2 in, 2 out]
                n1164 = property on="量程选择" class="Enum (严格)"() -> ("RingText.Text"=w1724:string)  [unwired: 2 in, 2 out]
                n1165 = Concatenate Strings("变更后:" ("table输入"), "K:" ("字符串"), w1713, "B:" ("字符串"), w1712, "X^2:" ("字符串"), w1711) -> (w1717:string)
                n1166 = Concatenate Strings(w1726, w1725, w1724, "公式改变" ("日志信息")) -> (w1718:string)
                n1167 = Get Date/Time In Seconds() -> (seconds since 1Jan1904=w1730:timestamp)
                n1168 = Bundle(cluster=T12 {"时间标识"=timestamp(0 s since 1904-01-01), "参数"="", "日志信息"="", "流程参数"=""} ("data in"), "时间标识"=w1730, "参数"="CODMn" ("table输入"), "日志信息"=w1718, "流程参数"=w1717) -> (w1728:T12)
                n1169 = call "流程日志字段定义.vi"("table输入"="操作日志", "data in"=w1728) -> ("table输出"=w1733:string, "columns"=w1734:string[], "data out"=w1735:T15)  [unwired: 7 in]
                n1170 = call "插入数据.vi"("data"=w1735, "columns"=w1734, "database"="database3.mdb", "table"=w1733) -> ()  [unwired: 7 in, 1 out]
              }
              frame Error {
              }
            }
            n1171 = One Button Dialog(message=w1705) -> ()  [unwired: 1 in, 1 out]
          }
        }
      }
      event "一键写入": Value Change {
        n1172 = event-data() -> ()  [unwired: 1 in, 6 out]
        n1173 = Two Button Dialog(message="确认是否写入公式，写入会覆盖原有公式！" ("消息")) -> (T button?=w1825:bool)  [unwired: 2 in]
        n1174 = case shown="真" w1825 {
          frame False {
          }
          frame True {
            n1175 = local read "模型"() -> (w1829:enum32{"线性", "多项式"})
            n1176 = case shown="\"线性\", 默认" w1829 {
              tunnel: [w1858 w1909] -> w1827
              frame "线性", Default {
                n1177 = property on="测量模式(公式)" class="Ring (严格)"() -> ("NumItems"=w1859:u32)  [unwired: 2 in, 2 out]
                n1178 = for {
                  N: w1859 -> [_]
                  tunnel: [w1860] -> w1858
                  i -> [w1865]
                  n1179 = Increment(x=w1865) -> (x+1=w1864:i32)
                  n1180 = local read "K"() -> (w1869:dbl)
                  n1181 = local read "b"() -> (w1870:dbl)
                  n1182 = case shown="1" w1864 {
                    tunnel: [u16 4626 ("starting address") w1875 w1880 w1885 w1890 w1895 w1900 w1905] -> w1862
                    frame 0, Default {
                    }
                    frame 1 {
                      n1183 = local read "量程选择"() -> (w1874:enum16{"低量程", "高量程", "0-2量程"})
                      n1184 = case shown="\"低量程\", 默认" w1874 {
                        tunnel: [u16 4626 ("starting address") u16 4632 ("starting address") u16 4638 ("starting address")] -> w1875
                        frame "低量程", Default {
                        }
                        frame "高量程" {
                        }
                        frame "0-2量程" {
                        }
                      }
                    }
                    frame 2 {
                      n1185 = local read "量程选择"() -> (w1879:enum16{"低量程", "高量程", "0-2量程"})
                      n1186 = case shown="\"低量程\", 默认" w1879 {
                        tunnel: [u16 4638 ("starting address") u16 4644 ("starting address") u16 4638 ("starting address")] -> w1880
                        frame "低量程", Default {
                        }
                        frame "高量程" {
                        }
                        frame "0-2量程" {
                        }
                      }
                    }
                    frame 3 {
                      n1187 = local read "量程选择"() -> (w1884:enum16{"低量程", "高量程", "0-2量程"})
                      n1188 = case shown="\"低量程\", 默认" w1884 {
                        tunnel: [u16 4650 ("starting address") u16 4656 ("starting address") u16 4638 ("starting address")] -> w1885
                        frame "低量程", Default {
                        }
                        frame "高量程" {
                        }
                        frame "0-2量程" {
                        }
                      }
                    }
                    frame 4 {
                      n1189 = local read "量程选择"() -> (w1889:enum16{"低量程", "高量程", "0-2量程"})
                      n1190 = case shown="\"高量程\"" w1889 {
                        tunnel: [u16 4662 ("starting address") u16 4668 ("starting address") u16 4638 ("starting address")] -> w1890
                        frame "低量程", Default {
                        }
                        frame "高量程" {
                        }
                        frame "0-2量程" {
                        }
                      }
                    }
                    frame 5 {
                      n1191 = local read "量程选择"() -> (w1894:enum16{"低量程", "高量程", "0-2量程"})
                      n1192 = case shown="\"低量程\", 默认" w1894 {
                        tunnel: [u16 4674 ("starting address") u16 4680 ("starting address") u16 4638 ("starting address")] -> w1895
                        frame "低量程", Default {
                        }
                        frame "高量程" {
                        }
                        frame "0-2量程" {
                        }
                      }
                    }
                    frame 6 {
                      n1193 = local read "量程选择"() -> (w1899:enum16{"低量程", "高量程", "0-2量程"})
                      n1194 = case shown="\"低量程\", 默认" w1899 {
                        tunnel: [u16 4686 ("starting address") u16 4692 ("starting address") u16 4638 ("starting address")] -> w1900
                        frame "低量程", Default {
                        }
                        frame "高量程" {
                        }
                        frame "0-2量程" {
                        }
                      }
                    }
                    frame 7 {
                      n1195 = local read "量程选择"() -> (w1904:enum16{"低量程", "高量程", "0-2量程"})
                      n1196 = case shown="\"低量程\", 默认" w1904 {
                        tunnel: [u16 4698 ("starting address") u16 4704 ("starting address") u16 4638 ("starting address")] -> w1905
                        frame "低量程", Default {
                        }
                        frame "高量程" {
                        }
                        frame "0-2量程" {
                        }
                      }
                    }
                  }
                  n1197 = Build Array(w1869, w1870, 0.0 ("元素")) -> (w1871:dbl[])
                  n1198 = call "浮点转CDAB整形cod.vi"("浮点数"=w1871) -> ("CDAB整形输出"=w1868:u16[])  [unwired: 10 in]
                  n1199 = Insert Into Array(array=u16[] [], index=0 ("索引"), new element=w1868) -> (w1861:u16[])
                  n1200 = call "CODMnMB_api.vi"("STEP"=enum16{"open", "read", "write", "close"}."write", "values"=w1861, "starting address"=w1862) -> ("error out"=w1860:errorcluster)  [unwired: 6 in, 2 out]
                }
              }
              frame "多项式" {
                # "b,k,c"
                n1201 = property on="测量模式(公式)" class="Ring (严格)"() -> ("NumItems"=w1910:u32)  [unwired: 2 in, 2 out]
                n1202 = for {
                  N: w1910 -> [_]
                  tunnel: [w1911] -> w1909
                  i -> [w1916]
                  n1203 = Increment(x=w1916) -> (x+1=w1915:i32)
                  n1204 = local read "多项式系数"() -> (w1920:dbl[])
                  n1205 = case shown="2" w1915 {
                    tunnel: [u16 4626 ("starting address") w1927 w1932 w1937 w1942 w1947 w1952 w1957] -> w1912
                    frame 0, Default {
                    }
                    frame 1 {
                      n1206 = local read "量程选择"() -> (w1926:enum16{"低量程", "高量程", "0-2量程"})
                      n1207 = case shown="\"低量程\", 默认" w1926 {
                        tunnel: [u16 4626 ("starting address") u16 4632 ("starting address") u16 4638 ("starting address")] -> w1927
                        frame "低量程", Default {
                        }
                        frame "高量程" {
                        }
                        frame "0-2量程" {
                        }
                      }
                    }
                    frame 2 {
                      n1208 = local read "量程选择"() -> (w1931:enum16{"低量程", "高量程", "0-2量程"})
                      n1209 = case shown="\"低量程\", 默认" w1931 {
                        tunnel: [u16 4638 ("starting address") u16 4644 ("starting address") u16 4638 ("starting address")] -> w1932
                        frame "低量程", Default {
                        }
                        frame "高量程" {
                        }
                        frame "0-2量程" {
                        }
                      }
                    }
                    frame 3 {
                      n1210 = local read "量程选择"() -> (w1936:enum16{"低量程", "高量程", "0-2量程"})
                      n1211 = case shown="\"低量程\", 默认" w1936 {
                        tunnel: [u16 4650 ("starting address") u16 4656 ("starting address") u16 4638 ("starting address")] -> w1937
                        frame "低量程", Default {
                        }
                        frame "高量程" {
                        }
                        frame "0-2量程" {
                        }
                      }
                    }
                    frame 4 {
                      n1212 = local read "量程选择"() -> (w1941:enum16{"低量程", "高量程", "0-2量程"})
                      n1213 = case shown="\"低量程\", 默认" w1941 {
                        tunnel: [u16 4662 ("starting address") u16 4668 ("starting address") u16 4638 ("starting address")] -> w1942
                        frame "低量程", Default {
                        }
                        frame "高量程" {
                        }
                        frame "0-2量程" {
                        }
                      }
                    }
                    frame 5 {
                      n1214 = local read "量程选择"() -> (w1946:enum16{"低量程", "高量程", "0-2量程"})
                      n1215 = case shown="\"低量程\", 默认" w1946 {
                        tunnel: [u16 4674 ("starting address") u16 4680 ("starting address") u16 4638 ("starting address")] -> w1947
                        frame "低量程", Default {
                        }
                        frame "高量程" {
                        }
                        frame "0-2量程" {
                        }
                      }
                    }
                    frame 6 {
                      n1216 = local read "量程选择"() -> (w1951:enum16{"低量程", "高量程", "0-2量程"})
                      n1217 = case shown="\"低量程\", 默认" w1951 {
                        tunnel: [u16 4686 ("starting address") u16 4692 ("starting address") u16 4638 ("starting address")] -> w1952
                        frame "低量程", Default {
                        }
                        frame "高量程" {
                        }
                        frame "0-2量程" {
                        }
                      }
                    }
                    frame 7 {
                      n1218 = local read "量程选择"() -> (w1956:enum16{"低量程", "高量程", "0-2量程"})
                      n1219 = case shown="\"低量程\", 默认" w1956 {
                        tunnel: [u16 4698 ("starting address") u16 4704 ("starting address") u16 4638 ("starting address")] -> w1957
                        frame "低量程", Default {
                        }
                        frame "高量程" {
                        }
                        frame "0-2量程" {
                        }
                      }
                    }
                  }
                  n1220 = Index Array(array=w1920) -> (element #1=w1923:dbl, element #2=w1922:dbl, element #3=w1924:dbl)  [unwired: 3 in]
                  n1221 = Build Array(w1922, w1923, w1924) -> (w1921:dbl[])
                  n1222 = call "浮点转CDAB整形cod.vi"("浮点数"=w1921) -> ("CDAB整形输出"=w1919:u16[])  [unwired: 10 in]
                  n1223 = Insert Into Array(array=u16[] [], index=0 ("索引"), new element=w1919) -> (w1913:u16[])
                  n1224 = call "CODMnMB_api.vi"("STEP"=enum16{"open", "read", "write", "close"}."write", "values"=w1913, "starting address"=w1912) -> ("error out"=w1911:errorcluster)  [unwired: 6 in, 2 out]
                }
              }
            }
            n1225 = case shown="无错误" w1827 {
              tunnel: ["写入成功！" "写入失败！"] -> w1828
              frame No Error {
                n1226 = local read "多项式系数"() -> (w1833:dbl[])
                n1227 = Index Array(array=w1833) -> (element #1=w1832:dbl, element #2=w1831:dbl, element #3=w1830:dbl)  [unwired: 3 in]
                n1228 = Number To Fractional String(number=w1832) -> (F-format string=w1836:string)  [unwired: 3 in]
                n1229 = Number To Fractional String(number=w1831) -> (F-format string=w1837:string)  [unwired: 3 in]
                n1230 = Number To Fractional String(number=w1830) -> (F-format string=w1835:string)  [unwired: 3 in]
                n1231 = property on="模型" class="Enum (严格)"() -> ("RingText.Text"=w1846:string)  [unwired: 2 in, 2 out]
                n1232 = property on="量程选择" class="Enum (严格)"() -> ("RingText.Text"=w1845:string)  [unwired: 2 in, 2 out]
                n1233 = Concatenate Strings("变更后:" ("table输入"), "K:" ("字符串"), w1837, "B:" ("字符串"), w1836, "X^2:" ("字符串"), w1835) -> (w1838:string)
                n1234 = Concatenate Strings(w1846, "【一键写入全部模式】" ("日志信息"), w1845, "公式改变" ("日志信息")) -> (w1839:string)
                n1235 = Get Date/Time In Seconds() -> (seconds since 1Jan1904=w1850:timestamp)
                n1236 = Bundle(cluster=T12 {"时间标识"=timestamp(0 s since 1904-01-01), "参数"="", "日志信息"="", "流程参数"=""} ("data in"), "时间标识"=w1850, "参数"="CODMn" ("table输入"), "日志信息"=w1839, "流程参数"=w1838) -> (w1848:T12)
                n1237 = call "流程日志字段定义.vi"("table输入"="操作日志", "data in"=w1848) -> ("table输出"=w1853:string, "columns"=w1854:string[], "data out"=w1855:T15)  [unwired: 7 in]
                n1238 = call "插入数据.vi"("data"=w1855, "columns"=w1854, "database"="database3.mdb", "table"=w1853) -> ()  [unwired: 7 in, 1 out]
              }
              frame Error {
              }
            }
            n1239 = One Button Dialog(message=w1828) -> ()  [unwired: 1 in, 1 out]
          }
        }
      }
      event "滴定曲线": Value Change {
        n1240 = event-data() -> ()  [unwired: 1 in, 6 out]
        n1241 = property on="窗格" class="Pane"("Origin"=T5 {"Horizontal"=0, "Vertical"=3200} ("原点")) -> ()  [unwired: 2 in, 2 out]
      }
      event "历史波形": Value Change {
        n1242 = event-data() -> ()  [unwired: 1 in, 6 out]
        n1243 = call-poly <vilib>:"Read Waveforms from File.vi"() -> ("error out"=w1962:errorcluster, "first waveform in record"=w1963:waveform(dbl))  [unwired: 6 in, 2 out]
        n1244 = case shown="无错误" w1962 {
          tunnel: w1963 -> [w1966 _]
          frame No Error {
            n1245 = Unbundle By Name(w1966) -> ("t0"=→"波形时间":timestamp, "Y"=w1965:dbl[])  [unwired: 2 out]
            n1246 = local write "ORP滴定曲线"(w1965) -> ()
            n1247 = local write "滴定数-ORP值"(w1965) -> ()
          }
          frame Error {
            n1248 = One Button Dialog(message="打开失败" ("消息")) -> ()  [unwired: 1 in, 1 out]
          }
        }
      }
      event "释放串口": Value Change {
        n1249 = event-data() -> ()  [unwired: 1 in, 6 out]
        n1250 = Two Button Dialog(message="确认是否释放串口，释放串口将导致通信失败！" ("消息")) -> (T button?=w1968:bool)  [unwired: 2 in]
        n1251 = case shown="真" w1968 {
          tunnel: w1971 -> [_ w1973]
          tunnel: w1970 -> [_ w1972]
          frame False {
          }
          frame True {
            n1252 = Bundle By Name(cluster=cluster{"命令":string} {"命令"=""} ("元素"), "命令"="停用模块" ("名称（未命名）")) -> (w1974:cluster{"命令":string})
            n1253 = Enqueue Element(queue=w1973, element=w1974, error in (no error)=w1972) -> ()  [unwired: 1 in, 3 out]
          }
        }
      }
      event "打开串口": Value Change {
        n1254 = event-data() -> ()  [unwired: 1 in, 6 out]
        n1255 = flat-sequence {
          tunnel: w1978 -> [w1986]
          tunnel: w1977 -> [w1985]
          frame #0 {
            n1256 = global read "CODMn断电保存全局变量.vi" "VISA resource name"() -> (w1989:refnum<visa-resource-name>)
            n1257 = global read "CODMn断电保存全局变量.vi" "MB通信方式选择"() -> (w1982:enum16{"串口", "TCP"})
            n1258 = global read "CODMn断电保存全局变量.vi" "PORT"() -> (w1980:string)
            n1259 = global read "CODMn断电保存全局变量.vi" "IP"() -> (w1981:string)
            n1260 = call "串口配置.vi"("PORT"=w1980, "IP"=w1981, "MB通信方式选择"=w1982, "请选择串口:"=w1989) -> ("PORT 2"=w1983:string, "IP 2"=w1984:string, "确认 2"=w1987:bool, "VISA资源名称 2"=w1988:refnum<visa-resource-name>, "MB通信方式选择 2"=w1979:enum16{"串口", "TCP"})  [unwired: 3 in]
            n1261 = case shown="真" w1987 {
              tunnel: w1988 -> [_ w1998]
              tunnel: w1986 -> [_ w1994]
              tunnel: w1985 -> [_ w1993]
              tunnel: w1984 -> [_ w1992]
              tunnel: w1983 -> [_ w1991]
              tunnel: w1979 -> [_ w1990]
              frame False {
              }
              frame True {
                n1262 = global write "CODMn断电保存全局变量.vi" "IP"(w1992) -> ()
                n1263 = global write "CODMn断电保存全局变量.vi" "PORT"(w1991) -> ()
                n1264 = global write "CODMn断电保存全局变量.vi" "VISA resource name"(w1998) -> ()
                n1265 = global write "CODMn断电保存全局变量.vi" "MB通信方式选择"(w1990) -> ()
                n1266 = Bundle By Name(cluster=cluster{"命令":string} {"命令"=""} ("元素"), "命令"="启用模块" ("名称（未命名）")) -> (w1995:cluster{"命令":string})
                n1267 = Enqueue Element(queue=w1994, element=w1995, error in (no error)=w1993) -> ()  [unwired: 1 in, 3 out]
              }
            }
          }
          frame #1 {
            n1268 = global read "CODMN外部API.vi" "ping"() -> (w2000:bool)
            n1269 = case shown="假" w2000 {
              tunnel: [w2012 w2015] -> w1999
              frame False {
                n1270 = global read "COD内部交互全局.vi" "配置文件ini"() -> (w2014:string)
                n1271 = call <vilib>:"Application Directory.vi"() -> ("Application Directory"=w2013:path)
                n1272 = Build Path(base path=w2013, name or relative path=w2014) -> (appended path=w2012:path)
              }
              frame True {
                n1273 = global read "CODMN外部API.vi" "配置文件 path"() -> (w2015:path)
              }
            }
            n1274 = call <vilib>:"Open Config Data.vi"("configuration file path"=w1999) -> ("error out"=w2004:errorcluster, "refnum"=w2001:T6)  [unwired: 8 in, 1 out]
            n1275 = vi-ref "斯坦道CODMn.lvlib:CODMn断电保存全局变量.vi"() -> (w2002:refnum<vi>)
            n1276 = call <userlib>:"Write Panel to INI__ogtk.vi"("error in (no error)"=w2004, "VI ref"=w2002, "refnum"=w2001) -> ("error out"=w2005:errorcluster, "refnum out"=w2003:T6)  [unwired: 7 in]
            n1277 = call <vilib>:"Close Config Data.vi"("error in (no error)"=w2005, "refnum"=w2003) -> ("error out"=w2010:errorcluster, "file path"=w2011:path)  [unwired: 8 in]
            n1278 = Open/Create/Replace File(file path (use dialog)=w2011, error in=w2010) -> (refnum out=w2007:refnum<file>, error out=w2006:errorcluster)  [unwired: 4 in, 1 out]
            n1279 = Flush File(refnum=w2007, error in=w2006) -> (refnum out=w2008:refnum<file>, error out=w2009:errorcluster)
            n1280 = Close File(refnum=w2008, error in=w2009) -> ()  [unwired: 2 out]
          }
        }
      }
      event "更新程序": Value Change {
        n1281 = event-data() -> ("CtlRef"=w2018:refnum<vi>, "NewVal"=w2019:bool)  [unwired: 1 in, 4 out]
        n1282 = case shown="真" w2019 {
          tunnel: w2018 -> [_ w2028]
          tunnel: w2017 -> [w2021 w2027]
          tunnel: w2016 -> [w2020 w2026]
          frame False {
            n1283 = Bundle By Name(cluster=cluster{"命令":string} {"命令"=""} ("元素"), "命令"="启用模块" ("名称（未命名）")) -> (w2022:cluster{"命令":string})
            n1284 = Enqueue Element(queue=w2021, element=w2022, error in (no error)=w2020) -> ()  [unwired: 1 in, 3 out]
          }
          frame True {
            n1285 = Two Button Dialog(message="警告，非专业人士请勿进行此操作！！！\n请确认是否继续？" ("消息")) -> (T button?=w2030:bool)  [unwired: 2 in]
            n1286 = case shown="真" w2030 {
              tunnel: w2028 -> [w2046 _]
              tunnel: w2027 -> [_ w2054]
              tunnel: w2026 -> [_ w2053]
              tunnel: [errorcluster {"status"=TRUE, "code"=0, "source"=""} ("error out") w2047] -> w2025
              frame False {
                n1287 = property class="Bool (严格)"(reference=w2046, "Value"=FALSE ("释放串口")) -> ()  [unwired: 1 in, 2 out]
              }
              frame True {
                n1288 = Bundle By Name(cluster=cluster{"命令":string} {"命令"=""} ("元素"), "命令"="CODMn程序更新" ("名称（未命名）")) -> (w2057:cluster{"命令":string})
                n1289 = Enqueue Element(queue=w2054, element=w2057, error in (no error)=w2053) -> (queue out=w2052:refnum<queue>, error out=w2051:errorcluster)  [unwired: 1 in, 1 out]
                n1290 = Bundle By Name(cluster=cluster{"命令":string} {"命令"=""} ("元素"), "命令"="停用模块" ("名称（未命名）")) -> (w2048:cluster{"命令":string})
                n1291 = Enqueue Element(queue=w2052, element=w2048, error in (no error)=w2051) -> (error out=w2047:errorcluster)  [unwired: 1 in, 2 out]
              }
            }
            n1292 = case shown="无错误" w2025 {
              frame No Error {
                n1293 = call "文件对话框"("start path"=path "D:/SRC") -> ("selected path"=w2033:path, "cancelled"=w2031:bool)  [unwired: 11 in, 2 out]
                n1294 = case shown="假" w2031 {
                  tunnel: w2033 -> [w2038 _]
                  frame False {
                    n1295 = Path To String(path=w2038) -> (string=w2035:string)
                    n1296 = Format Into String(format string="  - \"%s\"" ("格式字符串"), initial string="\"C:\\Program Files\\Fatek\\WinProladder\\WProlad.exe\"" ("command line"), w2035) -> (resulting string=w2036:string)  [unwired: 1 in, 1 out]
                    n1297 = call <vilib>:"System Exec.vi"("command line"=w2036) -> ("error out"=w2039:errorcluster)  [unwired: 7 in, 3 out]
                    n1298 = case shown="错误" w2039 {
                      tunnel: w2035 -> [_ w2042]
                      frame No Error {
                      }
                      frame Error {
                        n1299 = Format Into String(format string="  - \"%s\"" ("格式字符串"), initial string="\"C:\\Program Files (x86)\\Fatek\\WinProladder\\WProlad.exe\"" ("command line"), w2042) -> (resulting string=w2040:string)  [unwired: 1 in, 1 out]
                        n1300 = call <vilib>:"System Exec.vi"("command line"=w2040) -> ()  [unwired: 7 in, 4 out]
                      }
                    }
                  }
                  frame True {
                  }
                }
              }
              frame Error {
              }
            }
          }
        }
      }
      event Timeout {
        n1301 = event-data() -> ()  [unwired: 1 in, 3 out]
      }
    }
  }
  n1302 = property class="VI"(reference=w39, error in=w38) -> ("Name"=w40:string)  [unwired: 2 out]
  n1303 = Open VI Reference(type specifier VI Refnum (for type only)=refnum<vi> refnum, vi path=w40, options=128 ("选项")) -> (vi reference=w42:refnum<vi>, error out=w44:errorcluster)  [unwired: 3 in]
  n1304 = call-by-ref "?"(reference=w42, error in=w44) -> (reference out=w46:refnum<vi>, error out=w45:errorcluster)  [unwired: 12 in]
  n1305 = Close Reference(reference=w46, error in (no error)=w45) -> ()  [unwired: 1 out]
